vi "ZDataVIS_Stack_ITX_to_DATs.vi"(0 "File or Folder Path":path=path "G:/My Drive/ansom/Data/PPMS2/SA03008H.20180718/21-BG+SG_Sweep+OVERNIGHT", 1 "attempt to fix filtered time?":bool, 3 "length":i32=50, 5 "base processed path":path=path "C:/Users/voodoo/Desktop/IV_separat_Vsgsweep_2fields_Vbg-2.8V", 9 "pattern":string="*.itx", 12 "decimate files (1 for no)":i32=1, 14 "offset":i32) -> (4 "generated files":path[](array[path]), 6 "Index, Wavenames":string[][](table)=[["0", "'time.SA03008H.20180718.000049'\n"], ["1", "'temp.SA03008H.20180718.000049'\n"], ["2", "'B.SA03008H.20180718.000049'\n"], ["3", "'Vsource.SA03008H.20180718.000049'\n"], ["4", "'Lockin0.SA03008H.20180718.000049'\n"], ["5", "'Lockin1.SA03008H.20180718.000049'\n"], ["6", "'Lockin2.SA03008H.20180718.000049'\n"], ["7", "'Lockin3.SA03008H.20180718.000049'\n"], ["8", "'Lockin4.SA03008H.20180718.000049'\n"], ["9", "'Lockin5.SA03008H.20180718.000049'\n"], ["10", "'B_rate.SA03008H.20180718.000049'\n"], ["11", "'DC0.SA03008H.20180718.000049'\n"], ["12", "'DC1.SA03008H.20180718.000049'\n"], ["13", "'DC2.SA03008H.20180718.000049'\n"], ["14", "'DC3.SA03008H.20180718.000049'\n"], ["15", "'DC4.SA03008H.20180718.000049'\n"], ["16", "'DC5.SA03008H.20180718.000049'\n"], ["17", "'DC6.SA03008H.20180718.000049'\n"], ["18", "'DC7.SA03008H.20180718.000049'\n"], ["", ""]], 10 "\"notes \"":string[](array[string])=["IGOR\nX// Date: 7/18/2018 5:18 PM\nX// SA03008H\nX// \nX// Source 2 Drain 28 (lockin 1 and 7)\nX// Slow sweeping BG -5 to 5 inc. 0.1V \nX// Fast sweep SG -1 to 1 inc. 0.05V\n\nX// DSA_Vsg1=-1.000000\n\nX// \nX// B= 0.000000\n\n\n\n\n\n\n\n\n\n\n\n\n\n\n\n\n\n\n\n\n\n\n\n\n\n\n\n\n\n\n\n\n\n\n\n\n\n\n\n\nX \nX Display/R 'time.SA03008H.20180718.000000'\nX AppendToGraph 'temp.SA03008H.20180718.000000'\nX AppendToGraph 'B.SA03008H.20180718.000000'\nX AppendToGraph 'Vsource.SA03008H.20180718.000000'\nX AppendToGraph 'Lockin0.SA03008H.20180718.000000'\nX AppendToGraph 'Lockin1.SA03008H.20180718.000000'\nX AppendToGraph 'Lockin2.SA03008H.20180718.000000'\nX AppendToGraph 'Lockin3.SA03008H.20180718.000000'\nX AppendToGraph 'Lockin4.SA03008H.20180718.000000'\nX AppendToGraph 'Lockin5.SA03008H.20180718.000000'\nX AppendToGraph 'B_rate.SA03008H.20180718.000000'\nX AppendToGraph 'DC0.SA03008H.20180718.000000'\nX AppendToGraph 'DC1.SA03008H.20180718.000000'\nX AppendToGraph 'DC2.SA03008H.20180718.000000'\nX AppendToGraph 'DC3.SA03008H.20180718.000000'\nX AppendToGraph 'DC4.SA03008H.20180718.000000'\nX AppendToGraph 'DC5.SA03008H.20180718.000000'\nX AppendToGraph 'DC6.SA03008H.20180718.000000'\nX AppendToGraph 'DC7.SA03008H.20180718.000000'\nX Label bottom \"x label\"\nX Label left \"y label\"\nX ModifyGraph rgb('time.SA03008H.20180718.000000')=(65280,0,0)\nX ModifyGraph rgb('temp.SA03008H.20180718.000000')=(65280,18432,0)\nX ModifyGraph rgb('B.SA03008H.20180718.000000')=(65280,36864,0)\nX ModifyGraph rgb('Vsource.SA03008H.20180718.000000')=(65280,55296,0)\nX ModifyGraph rgb('Lockin0.SA03008H.20180718.000000')=(57344,65280,0)\nX ModifyGraph rgb('Lockin1.SA03008H.20180718.000000')=(37376,65280,0)\nX ModifyGraph rgb('Lockin2.SA03008H.20180718.000000')=(18944,65280,0)\nX ModifyGraph rgb('Lockin3.SA03008H.20180718.000000')=(512,65280,0)\nX ModifyGraph rgb('Lockin4.SA03008H.20180718.000000')=(0,65280,17920)\nX ModifyGraph rgb('Lockin5.SA03008H.20180718.000000')=(0,65280,36352)\nX ModifyGraph rgb('B_rate.SA03008H.20180718.000000')=(0,65280,54784)\nX ModifyGraph rgb('DC0.SA03008H.20180718.000000')=(0,57856,65280)\nX ModifyGraph rgb('DC1.SA03008H.20180718.000000')=(0,39424,65280)\nX ModifyGraph rgb('DC2.SA03008H.20180718.000000')=(0,20992,65280)\nX ModifyGraph rgb('DC3.SA03008H.20180718.000000')=(0,2560,65280)\nX ModifyGraph rgb('DC4.SA03008H.20180718.000000')=(17408,0,65280)\nX ModifyGraph rgb('DC5.SA03008H.20180718.000000')=(35840,0,65280)\nX ModifyGraph rgb('DC6.SA03008H.20180718.000000')=(54272,0,65280)\nX ModifyGraph rgb('DC7.SA03008H.20180718.000000')=(65280,0,58368)\nX Legend/C/N=text0/J \"\\\\s('time.SA03008H.20180718.000000') time\\r\\\\s('temp.SA03008H.20180718.000000') temp\\r\\\\s('B.SA03008H.20180718.000000') B\\r\\\\s('Vsource.SA03008H.20180718.000000') Vsource\\r\\\\s('Lockin0.SA03008H.20180718.000000') Lockin0\\r\\\\s('Lockin1.SA03008H.20180718.000000') Lockin1\\r\\\\s('Lockin2.SA03008H.20180718.000000') Lockin2\\r\\\\s('Lockin3.SA03008H.20180718.000000') Lockin3\\r\\\\s('Lockin4.SA03008H.20180718.000000') Lockin4\\r\\\\s('Lockin5.SA03008H.20180718.000000') Lockin5\\r\\\\s('B_rate.SA03008H.20180718.000000') B_rate\\r\\\\s('DC0.SA03008H.20180718.000000') DC0\\r\\\\s('DC1.SA03008H.20180718.000000') DC1\\r\\\\s('DC2.SA03008H.20180718.000000') DC2\\r\\\\s('DC3.SA03008H.20180718.000000') DC3\\r\\\\s('DC4.SA03008H.20180718.000000') DC4\\r\\\\s('DC5.SA03008H.20180718.000000') DC5\\r\\\\s('DC6.SA03008H.20180718.000000') DC6\\r\\\\s('DC7.SA03008H.20180718.000000') DC7\"\nX ModifyGraph mirror(bottom)=1\nX ModifyGraph width=216\nX ModifyGraph height={Aspect,0.6}\nX ModifyGraph Log(bottom)=0\nX ModifyGraph Log(left)=0\nX \n", "IGOR\nX// Date: 7/18/2018 5:18 PM\nX// SA03008H\nX// \nX// Source 2 Drain 28 (lockin 1 and 7)\nX// Slow sweeping BG -5 to 5 inc. 0.1V \nX// Fast sweep SG -1 to 1 inc. 0.05V\n\nX// DSA_Vsg1=-0.950000\n\nX// \nX// B= 0.000000\n\n\n\n\n\n\n\n\n\n\n\n\n\n\n\n\n\n\n\n\n\n\n\n\n\n\n\n\n\n\n\n\n\n\n\n\n\n\n\n\nX \nX Display/R 'time.SA03008H.20180718.000001'\nX AppendToGraph 'temp.SA03008H.20180718.000001'\nX AppendToGraph 'B.SA03008H.20180718.000001'\nX AppendToGraph 'Vsource.SA03008H.20180718.000001'\nX AppendToGraph 'Lockin0.SA03008H.20180718.000001'\nX AppendToGraph 'Lockin1.SA03008H.20180718.000001'\nX AppendToGraph 'Lockin2.SA03008H.20180718.000001'\nX AppendToGraph 'Lockin3.SA03008H.20180718.000001'\nX AppendToGraph 'Lockin4.SA03008H.20180718.000001'\nX AppendToGraph 'Lockin5.SA03008H.20180718.000001'\nX AppendToGraph 'B_rate.SA03008H.20180718.000001'\nX AppendToGraph 'DC0.SA03008H.20180718.000001'\nX AppendToGraph 'DC1.SA03008H.20180718.000001'\nX AppendToGraph 'DC2.SA03008H.20180718.000001'\nX AppendToGraph 'DC3.SA03008H.20180718.000001'\nX AppendToGraph 'DC4.SA03008H.20180718.000001'\nX AppendToGraph 'DC5.SA03008H.20180718.000001'\nX AppendToGraph 'DC6.SA03008H.20180718.000001'\nX AppendToGraph 'DC7.SA03008H.20180718.000001'\nX Label bottom \"x label\"\nX Label left \"y label\"\nX ModifyGraph rgb('time.SA03008H.20180718.000001')=(65280,0,0)\nX ModifyGraph rgb('temp.SA03008H.20180718.000001')=(65280,18432,0)\nX ModifyGraph rgb('B.SA03008H.20180718.000001')=(65280,36864,0)\nX ModifyGraph rgb('Vsource.SA03008H.20180718.000001')=(65280,55296,0)\nX ModifyGraph rgb('Lockin0.SA03008H.20180718.000001')=(57344,65280,0)\nX ModifyGraph rgb('Lockin1.SA03008H.20180718.000001')=(37376,65280,0)\nX ModifyGraph rgb('Lockin2.SA03008H.20180718.000001')=(18944,65280,0)\nX ModifyGraph rgb('Lockin3.SA03008H.20180718.000001')=(512,65280,0)\nX ModifyGraph rgb('Lockin4.SA03008H.20180718.000001')=(0,65280,17920)\nX ModifyGraph rgb('Lockin5.SA03008H.20180718.000001')=(0,65280,36352)\nX ModifyGraph rgb('B_rate.SA03008H.20180718.000001')=(0,65280,54784)\nX ModifyGraph rgb('DC0.SA03008H.20180718.000001')=(0,57856,65280)\nX ModifyGraph rgb('DC1.SA03008H.20180718.000001')=(0,39424,65280)\nX ModifyGraph rgb('DC2.SA03008H.20180718.000001')=(0,20992,65280)\nX ModifyGraph rgb('DC3.SA03008H.20180718.000001')=(0,2560,65280)\nX ModifyGraph rgb('DC4.SA03008H.20180718.000001')=(17408,0,65280)\nX ModifyGraph rgb('DC5.SA03008H.20180718.000001')=(35840,0,65280)\nX ModifyGraph rgb('DC6.SA03008H.20180718.000001')=(54272,0,65280)\nX ModifyGraph rgb('DC7.SA03008H.20180718.000001')=(65280,0,58368)\nX Legend/C/N=text0/J \"\\\\s('time.SA03008H.20180718.000001') time\\r\\\\s('temp.SA03008H.20180718.000001') temp\\r\\\\s('B.SA03008H.20180718.000001') B\\r\\\\s('Vsource.SA03008H.20180718.000001') Vsource\\r\\\\s('Lockin0.SA03008H.20180718.000001') Lockin0\\r\\\\s('Lockin1.SA03008H.20180718.000001') Lockin1\\r\\\\s('Lockin2.SA03008H.20180718.000001') Lockin2\\r\\\\s('Lockin3.SA03008H.20180718.000001') Lockin3\\r\\\\s('Lockin4.SA03008H.20180718.000001') Lockin4\\r\\\\s('Lockin5.SA03008H.20180718.000001') Lockin5\\r\\\\s('B_rate.SA03008H.20180718.000001') B_rate\\r\\\\s('DC0.SA03008H.20180718.000001') DC0\\r\\\\s('DC1.SA03008H.20180718.000001') DC1\\r\\\\s('DC2.SA03008H.20180718.000001') DC2\\r\\\\s('DC3.SA03008H.20180718.000001') DC3\\r\\\\s('DC4.SA03008H.20180718.000001') DC4\\r\\\\s('DC5.SA03008H.20180718.000001') DC5\\r\\\\s('DC6.SA03008H.20180718.000001') DC6\\r\\\\s('DC7.SA03008H.20180718.000001') DC7\"\nX ModifyGraph mirror(bottom)=1\nX ModifyGraph width=216\nX ModifyGraph height={Aspect,0.6}\nX ModifyGraph Log(bottom)=0\nX ModifyGraph Log(left)=0\nX \n", "IGOR\nX// Date: 7/18/2018 5:19 PM\nX// SA03008H\nX// \nX// Source 2 Drain 28 (lockin 1 and 7)\nX// Slow sweeping BG -5 to 5 inc. 0.1V \nX// Fast sweep SG -1 to 1 inc. 0.05V\n\nX// DSA_Vsg1=-0.900000\n\nX// \nX// B= 0.000000\n\n\n\n\n\n\n\n\n\n\n\n\n\n\n\n\n\n\n\n\n\n\n\n\n\n\n\n\n\n\n\n\n\n\n\n\n\n\n\n\nX \nX Display/R 'time.SA03008H.20180718.000002'\nX AppendToGraph 'temp.SA03008H.20180718.000002'\nX AppendToGraph 'B.SA03008H.20180718.000002'\nX AppendToGraph 'Vsource.SA03008H.20180718.000002'\nX AppendToGraph 'Lockin0.SA03008H.20180718.000002'\nX AppendToGraph 'Lockin1.SA03008H.20180718.000002'\nX AppendToGraph 'Lockin2.SA03008H.20180718.000002'\nX AppendToGraph 'Lockin3.SA03008H.20180718.000002'\nX AppendToGraph 'Lockin4.SA03008H.20180718.000002'\nX AppendToGraph 'Lockin5.SA03008H.20180718.000002'\nX AppendToGraph 'B_rate.SA03008H.20180718.000002'\nX AppendToGraph 'DC0.SA03008H.20180718.000002'\nX AppendToGraph 'DC1.SA03008H.20180718.000002'\nX AppendToGraph 'DC2.SA03008H.20180718.000002'\nX AppendToGraph 'DC3.SA03008H.20180718.000002'\nX AppendToGraph 'DC4.SA03008H.20180718.000002'\nX AppendToGraph 'DC5.SA03008H.20180718.000002'\nX AppendToGraph 'DC6.SA03008H.20180718.000002'\nX AppendToGraph 'DC7.SA03008H.20180718.000002'\nX Label bottom \"x label\"\nX Label left \"y label\"\nX ModifyGraph rgb('time.SA03008H.20180718.000002')=(65280,0,0)\nX ModifyGraph rgb('temp.SA03008H.20180718.000002')=(65280,18432,0)\nX ModifyGraph rgb('B.SA03008H.20180718.000002')=(65280,36864,0)\nX ModifyGraph rgb('Vsource.SA03008H.20180718.000002')=(65280,55296,0)\nX ModifyGraph rgb('Lockin0.SA03008H.20180718.000002')=(57344,65280,0)\nX ModifyGraph rgb('Lockin1.SA03008H.20180718.000002')=(37376,65280,0)\nX ModifyGraph rgb('Lockin2.SA03008H.20180718.000002')=(18944,65280,0)\nX ModifyGraph rgb('Lockin3.SA03008H.20180718.000002')=(512,65280,0)\nX ModifyGraph rgb('Lockin4.SA03008H.20180718.000002')=(0,65280,17920)\nX ModifyGraph rgb('Lockin5.SA03008H.20180718.000002')=(0,65280,36352)\nX ModifyGraph rgb('B_rate.SA03008H.20180718.000002')=(0,65280,54784)\nX ModifyGraph rgb('DC0.SA03008H.20180718.000002')=(0,57856,65280)\nX ModifyGraph rgb('DC1.SA03008H.20180718.000002')=(0,39424,65280)\nX ModifyGraph rgb('DC2.SA03008H.20180718.000002')=(0,20992,65280)\nX ModifyGraph rgb('DC3.SA03008H.20180718.000002')=(0,2560,65280)\nX ModifyGraph rgb('DC4.SA03008H.20180718.000002')=(17408,0,65280)\nX ModifyGraph rgb('DC5.SA03008H.20180718.000002')=(35840,0,65280)\nX ModifyGraph rgb('DC6.SA03008H.20180718.000002')=(54272,0,65280)\nX ModifyGraph rgb('DC7.SA03008H.20180718.000002')=(65280,0,58368)\nX Legend/C/N=text0/J \"\\\\s('time.SA03008H.20180718.000002') time\\r\\\\s('temp.SA03008H.20180718.000002') temp\\r\\\\s('B.SA03008H.20180718.000002') B\\r\\\\s('Vsource.SA03008H.20180718.000002') Vsource\\r\\\\s('Lockin0.SA03008H.20180718.000002') Lockin0\\r\\\\s('Lockin1.SA03008H.20180718.000002') Lockin1\\r\\\\s('Lockin2.SA03008H.20180718.000002') Lockin2\\r\\\\s('Lockin3.SA03008H.20180718.000002') Lockin3\\r\\\\s('Lockin4.SA03008H.20180718.000002') Lockin4\\r\\\\s('Lockin5.SA03008H.20180718.000002') Lockin5\\r\\\\s('B_rate.SA03008H.20180718.000002') B_rate\\r\\\\s('DC0.SA03008H.20180718.000002') DC0\\r\\\\s('DC1.SA03008H.20180718.000002') DC1\\r\\\\s('DC2.SA03008H.20180718.000002') DC2\\r\\\\s('DC3.SA03008H.20180718.000002') DC3\\r\\\\s('DC4.SA03008H.20180718.000002') DC4\\r\\\\s('DC5.SA03008H.20180718.000002') DC5\\r\\\\s('DC6.SA03008H.20180718.000002') DC6\\r\\\\s('DC7.SA03008H.20180718.000002') DC7\"\nX ModifyGraph mirror(bottom)=1\nX ModifyGraph width=216\nX ModifyGraph height={Aspect,0.6}\nX ModifyGraph Log(bottom)=0\nX ModifyGraph Log(left)=0\nX \n", "IGOR\nX// Date: 7/18/2018 5:19 PM\nX// SA03008H\nX// \nX// Source 2 Drain 28 (lockin 1 and 7)\nX// Slow sweeping BG -5 to 5 inc. 0.1V \nX// Fast sweep SG -1 to 1 inc. 0.05V\n\nX// DSA_Vsg1=-0.850000\n\nX// \nX// B= 0.000000\n\n\n\n\n\n\n\n\n\n\n\n\n\n\n\n\n\n\n\n\n\n\n\n\n\n\n\n\n\n\n\n\n\n\n\n\n\n\n\n\nX \nX Display/R 'time.SA03008H.20180718.000003'\nX AppendToGraph 'temp.SA03008H.20180718.000003'\nX AppendToGraph 'B.SA03008H.20180718.000003'\nX AppendToGraph 'Vsource.SA03008H.20180718.000003'\nX AppendToGraph 'Lockin0.SA03008H.20180718.000003'\nX AppendToGraph 'Lockin1.SA03008H.20180718.000003'\nX AppendToGraph 'Lockin2.SA03008H.20180718.000003'\nX AppendToGraph 'Lockin3.SA03008H.20180718.000003'\nX AppendToGraph 'Lockin4.SA03008H.20180718.000003'\nX AppendToGraph 'Lockin5.SA03008H.20180718.000003'\nX AppendToGraph 'B_rate.SA03008H.20180718.000003'\nX AppendToGraph 'DC0.SA03008H.20180718.000003'\nX AppendToGraph 'DC1.SA03008H.20180718.000003'\nX AppendToGraph 'DC2.SA03008H.20180718.000003'\nX AppendToGraph 'DC3.SA03008H.20180718.000003'\nX AppendToGraph 'DC4.SA03008H.20180718.000003'\nX AppendToGraph 'DC5.SA03008H.20180718.000003'\nX AppendToGraph 'DC6.SA03008H.20180718.000003'\nX AppendToGraph 'DC7.SA03008H.20180718.000003'\nX Label bottom \"x label\"\nX Label left \"y label\"\nX ModifyGraph rgb('time.SA03008H.20180718.000003')=(65280,0,0)\nX ModifyGraph rgb('temp.SA03008H.20180718.000003')=(65280,18432,0)\nX ModifyGraph rgb('B.SA03008H.20180718.000003')=(65280,36864,0)\nX ModifyGraph rgb('Vsource.SA03008H.20180718.000003')=(65280,55296,0)\nX ModifyGraph rgb('Lockin0.SA03008H.20180718.000003')=(57344,65280,0)\nX ModifyGraph rgb('Lockin1.SA03008H.20180718.000003')=(37376,65280,0)\nX ModifyGraph rgb('Lockin2.SA03008H.20180718.000003')=(18944,65280,0)\nX ModifyGraph rgb('Lockin3.SA03008H.20180718.000003')=(512,65280,0)\nX ModifyGraph rgb('Lockin4.SA03008H.20180718.000003')=(0,65280,17920)\nX ModifyGraph rgb('Lockin5.SA03008H.20180718.000003')=(0,65280,36352)\nX ModifyGraph rgb('B_rate.SA03008H.20180718.000003')=(0,65280,54784)\nX ModifyGraph rgb('DC0.SA03008H.20180718.000003')=(0,57856,65280)\nX ModifyGraph rgb('DC1.SA03008H.20180718.000003')=(0,39424,65280)\nX ModifyGraph rgb('DC2.SA03008H.20180718.000003')=(0,20992,65280)\nX ModifyGraph rgb('DC3.SA03008H.20180718.000003')=(0,2560,65280)\nX ModifyGraph rgb('DC4.SA03008H.20180718.000003')=(17408,0,65280)\nX ModifyGraph rgb('DC5.SA03008H.20180718.000003')=(35840,0,65280)\nX ModifyGraph rgb('DC6.SA03008H.20180718.000003')=(54272,0,65280)\nX ModifyGraph rgb('DC7.SA03008H.20180718.000003')=(65280,0,58368)\nX Legend/C/N=text0/J \"\\\\s('time.SA03008H.20180718.000003') time\\r\\\\s('temp.SA03008H.20180718.000003') temp\\r\\\\s('B.SA03008H.20180718.000003') B\\r\\\\s('Vsource.SA03008H.20180718.000003') Vsource\\r\\\\s('Lockin0.SA03008H.20180718.000003') Lockin0\\r\\\\s('Lockin1.SA03008H.20180718.000003') Lockin1\\r\\\\s('Lockin2.SA03008H.20180718.000003') Lockin2\\r\\\\s('Lockin3.SA03008H.20180718.000003') Lockin3\\r\\\\s('Lockin4.SA03008H.20180718.000003') Lockin4\\r\\\\s('Lockin5.SA03008H.20180718.000003') Lockin5\\r\\\\s('B_rate.SA03008H.20180718.000003') B_rate\\r\\\\s('DC0.SA03008H.20180718.000003') DC0\\r\\\\s('DC1.SA03008H.20180718.000003') DC1\\r\\\\s('DC2.SA03008H.20180718.000003') DC2\\r\\\\s('DC3.SA03008H.20180718.000003') DC3\\r\\\\s('DC4.SA03008H.20180718.000003') DC4\\r\\\\s('DC5.SA03008H.20180718.000003') DC5\\r\\\\s('DC6.SA03008H.20180718.000003') DC6\\r\\\\s('DC7.SA03008H.20180718.000003') DC7\"\nX ModifyGraph mirror(bottom)=1\nX ModifyGraph width=216\nX ModifyGraph height={Aspect,0.6}\nX ModifyGraph Log(bottom)=0\nX ModifyGraph Log(left)=0\nX \n", "IGOR\nX// Date: 7/18/2018 5:19 PM\nX// SA03008H\nX// \nX// Source 2 Drain 28 (lockin 1 and 7)\nX// Slow sweeping BG -5 to 5 inc. 0.1V \nX// Fast sweep SG -1 to 1 inc. 0.05V\n\nX// DSA_Vsg1=-0.800000\n\nX// \nX// B= 0.000000\n\n\n\n\n\n\n\n\n\n\n\n\n\n\n\n\n\n\n\n\n\n\n\n\n\n\n\n\n\n\n\n\n\n\n\n\n\n\n\n\nX \nX Display/R 'time.SA03008H.20180718.000004'\nX AppendToGraph 'temp.SA03008H.20180718.000004'\nX AppendToGraph 'B.SA03008H.20180718.000004'\nX AppendToGraph 'Vsource.SA03008H.20180718.000004'\nX AppendToGraph 'Lockin0.SA03008H.20180718.000004'\nX AppendToGraph 'Lockin1.SA03008H.20180718.000004'\nX AppendToGraph 'Lockin2.SA03008H.20180718.000004'\nX AppendToGraph 'Lockin3.SA03008H.20180718.000004'\nX AppendToGraph 'Lockin4.SA03008H.20180718.000004'\nX AppendToGraph 'Lockin5.SA03008H.20180718.000004'\nX AppendToGraph 'B_rate.SA03008H.20180718.000004'\nX AppendToGraph 'DC0.SA03008H.20180718.000004'\nX AppendToGraph 'DC1.SA03008H.20180718.000004'\nX AppendToGraph 'DC2.SA03008H.20180718.000004'\nX AppendToGraph 'DC3.SA03008H.20180718.000004'\nX AppendToGraph 'DC4.SA03008H.20180718.000004'\nX AppendToGraph 'DC5.SA03008H.20180718.000004'\nX AppendToGraph 'DC6.SA03008H.20180718.000004'\nX AppendToGraph 'DC7.SA03008H.20180718.000004'\nX Label bottom \"x label\"\nX Label left \"y label\"\nX ModifyGraph rgb('time.SA03008H.20180718.000004')=(65280,0,0)\nX ModifyGraph rgb('temp.SA03008H.20180718.000004')=(65280,18432,0)\nX ModifyGraph rgb('B.SA03008H.20180718.000004')=(65280,36864,0)\nX ModifyGraph rgb('Vsource.SA03008H.20180718.000004')=(65280,55296,0)\nX ModifyGraph rgb('Lockin0.SA03008H.20180718.000004')=(57344,65280,0)\nX ModifyGraph rgb('Lockin1.SA03008H.20180718.000004')=(37376,65280,0)\nX ModifyGraph rgb('Lockin2.SA03008H.20180718.000004')=(18944,65280,0)\nX ModifyGraph rgb('Lockin3.SA03008H.20180718.000004')=(512,65280,0)\nX ModifyGraph rgb('Lockin4.SA03008H.20180718.000004')=(0,65280,17920)\nX ModifyGraph rgb('Lockin5.SA03008H.20180718.000004')=(0,65280,36352)\nX ModifyGraph rgb('B_rate.SA03008H.20180718.000004')=(0,65280,54784)\nX ModifyGraph rgb('DC0.SA03008H.20180718.000004')=(0,57856,65280)\nX ModifyGraph rgb('DC1.SA03008H.20180718.000004')=(0,39424,65280)\nX ModifyGraph rgb('DC2.SA03008H.20180718.000004')=(0,20992,65280)\nX ModifyGraph rgb('DC3.SA03008H.20180718.000004')=(0,2560,65280)\nX ModifyGraph rgb('DC4.SA03008H.20180718.000004')=(17408,0,65280)\nX ModifyGraph rgb('DC5.SA03008H.20180718.000004')=(35840,0,65280)\nX ModifyGraph rgb('DC6.SA03008H.20180718.000004')=(54272,0,65280)\nX ModifyGraph rgb('DC7.SA03008H.20180718.000004')=(65280,0,58368)\nX Legend/C/N=text0/J \"\\\\s('time.SA03008H.20180718.000004') time\\r\\\\s('temp.SA03008H.20180718.000004') temp\\r\\\\s('B.SA03008H.20180718.000004') B\\r\\\\s('Vsource.SA03008H.20180718.000004') Vsource\\r\\\\s('Lockin0.SA03008H.20180718.000004') Lockin0\\r\\\\s('Lockin1.SA03008H.20180718.000004') Lockin1\\r\\\\s('Lockin2.SA03008H.20180718.000004') Lockin2\\r\\\\s('Lockin3.SA03008H.20180718.000004') Lockin3\\r\\\\s('Lockin4.SA03008H.20180718.000004') Lockin4\\r\\\\s('Lockin5.SA03008H.20180718.000004') Lockin5\\r\\\\s('B_rate.SA03008H.20180718.000004') B_rate\\r\\\\s('DC0.SA03008H.20180718.000004') DC0\\r\\\\s('DC1.SA03008H.20180718.000004') DC1\\r\\\\s('DC2.SA03008H.20180718.000004') DC2\\r\\\\s('DC3.SA03008H.20180718.000004') DC3\\r\\\\s('DC4.SA03008H.20180718.000004') DC4\\r\\\\s('DC5.SA03008H.20180718.000004') DC5\\r\\\\s('DC6.SA03008H.20180718.000004') DC6\\r\\\\s('DC7.SA03008H.20180718.000004') DC7\"\nX ModifyGraph mirror(bottom)=1\nX ModifyGraph width=216\nX ModifyGraph height={Aspect,0.6}\nX ModifyGraph Log(bottom)=0\nX ModifyGraph Log(left)=0\nX \n", "IGOR\nX// Date: 7/18/2018 5:19 PM\nX// SA03008H\nX// \nX// Source 2 Drain 28 (lockin 1 and 7)\nX// Slow sweeping BG -5 to 5 inc. 0.1V \nX// Fast sweep SG -1 to 1 inc. 0.05V\n\nX// DSA_Vsg1=-0.750000\n\nX// \nX// B= 0.000000\n\n\n\n\n\n\n\n\n\n\n\n\n\n\n\n\n\n\n\n\n\n\n\n\n\n\n\n\n\n\n\n\n\n\n\n\n\n\n\n\nX \nX Display/R 'time.SA03008H.20180718.000005'\nX AppendToGraph 'temp.SA03008H.20180718.000005'\nX AppendToGraph 'B.SA03008H.20180718.000005'\nX AppendToGraph 'Vsource.SA03008H.20180718.000005'\nX AppendToGraph 'Lockin0.SA03008H.20180718.000005'\nX AppendToGraph 'Lockin1.SA03008H.20180718.000005'\nX AppendToGraph 'Lockin2.SA03008H.20180718.000005'\nX AppendToGraph 'Lockin3.SA03008H.20180718.000005'\nX AppendToGraph 'Lockin4.SA03008H.20180718.000005'\nX AppendToGraph 'Lockin5.SA03008H.20180718.000005'\nX AppendToGraph 'B_rate.SA03008H.20180718.000005'\nX AppendToGraph 'DC0.SA03008H.20180718.000005'\nX AppendToGraph 'DC1.SA03008H.20180718.000005'\nX AppendToGraph 'DC2.SA03008H.20180718.000005'\nX AppendToGraph 'DC3.SA03008H.20180718.000005'\nX AppendToGraph 'DC4.SA03008H.20180718.000005'\nX AppendToGraph 'DC5.SA03008H.20180718.000005'\nX AppendToGraph 'DC6.SA03008H.20180718.000005'\nX AppendToGraph 'DC7.SA03008H.20180718.000005'\nX Label bottom \"x label\"\nX Label left \"y label\"\nX ModifyGraph rgb('time.SA03008H.20180718.000005')=(65280,0,0)\nX ModifyGraph rgb('temp.SA03008H.20180718.000005')=(65280,18432,0)\nX ModifyGraph rgb('B.SA03008H.20180718.000005')=(65280,36864,0)\nX ModifyGraph rgb('Vsource.SA03008H.20180718.000005')=(65280,55296,0)\nX ModifyGraph rgb('Lockin0.SA03008H.20180718.000005')=(57344,65280,0)\nX ModifyGraph rgb('Lockin1.SA03008H.20180718.000005')=(37376,65280,0)\nX ModifyGraph rgb('Lockin2.SA03008H.20180718.000005')=(18944,65280,0)\nX ModifyGraph rgb('Lockin3.SA03008H.20180718.000005')=(512,65280,0)\nX ModifyGraph rgb('Lockin4.SA03008H.20180718.000005')=(0,65280,17920)\nX ModifyGraph rgb('Lockin5.SA03008H.20180718.000005')=(0,65280,36352)\nX ModifyGraph rgb('B_rate.SA03008H.20180718.000005')=(0,65280,54784)\nX ModifyGraph rgb('DC0.SA03008H.20180718.000005')=(0,57856,65280)\nX ModifyGraph rgb('DC1.SA03008H.20180718.000005')=(0,39424,65280)\nX ModifyGraph rgb('DC2.SA03008H.20180718.000005')=(0,20992,65280)\nX ModifyGraph rgb('DC3.SA03008H.20180718.000005')=(0,2560,65280)\nX ModifyGraph rgb('DC4.SA03008H.20180718.000005')=(17408,0,65280)\nX ModifyGraph rgb('DC5.SA03008H.20180718.000005')=(35840,0,65280)\nX ModifyGraph rgb('DC6.SA03008H.20180718.000005')=(54272,0,65280)\nX ModifyGraph rgb('DC7.SA03008H.20180718.000005')=(65280,0,58368)\nX Legend/C/N=text0/J \"\\\\s('time.SA03008H.20180718.000005') time\\r\\\\s('temp.SA03008H.20180718.000005') temp\\r\\\\s('B.SA03008H.20180718.000005') B\\r\\\\s('Vsource.SA03008H.20180718.000005') Vsource\\r\\\\s('Lockin0.SA03008H.20180718.000005') Lockin0\\r\\\\s('Lockin1.SA03008H.20180718.000005') Lockin1\\r\\\\s('Lockin2.SA03008H.20180718.000005') Lockin2\\r\\\\s('Lockin3.SA03008H.20180718.000005') Lockin3\\r\\\\s('Lockin4.SA03008H.20180718.000005') Lockin4\\r\\\\s('Lockin5.SA03008H.20180718.000005') Lockin5\\r\\\\s('B_rate.SA03008H.20180718.000005') B_rate\\r\\\\s('DC0.SA03008H.20180718.000005') DC0\\r\\\\s('DC1.SA03008H.20180718.000005') DC1\\r\\\\s('DC2.SA03008H.20180718.000005') DC2\\r\\\\s('DC3.SA03008H.20180718.000005') DC3\\r\\\\s('DC4.SA03008H.20180718.000005') DC4\\r\\\\s('DC5.SA03008H.20180718.000005') DC5\\r\\\\s('DC6.SA03008H.20180718.000005') DC6\\r\\\\s('DC7.SA03008H.20180718.000005') DC7\"\nX ModifyGraph mirror(bottom)=1\nX ModifyGraph width=216\nX ModifyGraph height={Aspect,0.6}\nX ModifyGraph Log(bottom)=0\nX ModifyGraph Log(left)=0\nX \n", "IGOR\nX// Date: 7/18/2018 5:19 PM\nX// SA03008H\nX// \nX// Source 2 Drain 28 (lockin 1 and 7)\nX// Slow sweeping BG -5 to 5 inc. 0.1V \nX// Fast sweep SG -1 to 1 inc. 0.05V\n\nX// DSA_Vsg1=-0.700000\n\nX// \nX// B= 0.000000\n\n\n\n\n\n\n\n\n\n\n\n\n\n\n\n\n\n\n\n\n\n\n\n\n\n\n\n\n\n\n\n\n\n\n\n\n\n\n\n\nX \nX Display/R 'time.SA03008H.20180718.000006'\nX AppendToGraph 'temp.SA03008H.20180718.000006'\nX AppendToGraph 'B.SA03008H.20180718.000006'\nX AppendToGraph 'Vsource.SA03008H.20180718.000006'\nX AppendToGraph 'Lockin0.SA03008H.20180718.000006'\nX AppendToGraph 'Lockin1.SA03008H.20180718.000006'\nX AppendToGraph 'Lockin2.SA03008H.20180718.000006'\nX AppendToGraph 'Lockin3.SA03008H.20180718.000006'\nX AppendToGraph 'Lockin4.SA03008H.20180718.000006'\nX AppendToGraph 'Lockin5.SA03008H.20180718.000006'\nX AppendToGraph 'B_rate.SA03008H.20180718.000006'\nX AppendToGraph 'DC0.SA03008H.20180718.000006'\nX AppendToGraph 'DC1.SA03008H.20180718.000006'\nX AppendToGraph 'DC2.SA03008H.20180718.000006'\nX AppendToGraph 'DC3.SA03008H.20180718.000006'\nX AppendToGraph 'DC4.SA03008H.20180718.000006'\nX AppendToGraph 'DC5.SA03008H.20180718.000006'\nX AppendToGraph 'DC6.SA03008H.20180718.000006'\nX AppendToGraph 'DC7.SA03008H.20180718.000006'\nX Label bottom \"x label\"\nX Label left \"y label\"\nX ModifyGraph rgb('time.SA03008H.20180718.000006')=(65280,0,0)\nX ModifyGraph rgb('temp.SA03008H.20180718.000006')=(65280,18432,0)\nX ModifyGraph rgb('B.SA03008H.20180718.000006')=(65280,36864,0)\nX ModifyGraph rgb('Vsource.SA03008H.20180718.000006')=(65280,55296,0)\nX ModifyGraph rgb('Lockin0.SA03008H.20180718.000006')=(57344,65280,0)\nX ModifyGraph rgb('Lockin1.SA03008H.20180718.000006')=(37376,65280,0)\nX ModifyGraph rgb('Lockin2.SA03008H.20180718.000006')=(18944,65280,0)\nX ModifyGraph rgb('Lockin3.SA03008H.20180718.000006')=(512,65280,0)\nX ModifyGraph rgb('Lockin4.SA03008H.20180718.000006')=(0,65280,17920)\nX ModifyGraph rgb('Lockin5.SA03008H.20180718.000006')=(0,65280,36352)\nX ModifyGraph rgb('B_rate.SA03008H.20180718.000006')=(0,65280,54784)\nX ModifyGraph rgb('DC0.SA03008H.20180718.000006')=(0,57856,65280)\nX ModifyGraph rgb('DC1.SA03008H.20180718.000006')=(0,39424,65280)\nX ModifyGraph rgb('DC2.SA03008H.20180718.000006')=(0,20992,65280)\nX ModifyGraph rgb('DC3.SA03008H.20180718.000006')=(0,2560,65280)\nX ModifyGraph rgb('DC4.SA03008H.20180718.000006')=(17408,0,65280)\nX ModifyGraph rgb('DC5.SA03008H.20180718.000006')=(35840,0,65280)\nX ModifyGraph rgb('DC6.SA03008H.20180718.000006')=(54272,0,65280)\nX ModifyGraph rgb('DC7.SA03008H.20180718.000006')=(65280,0,58368)\nX Legend/C/N=text0/J \"\\\\s('time.SA03008H.20180718.000006') time\\r\\\\s('temp.SA03008H.20180718.000006') temp\\r\\\\s('B.SA03008H.20180718.000006') B\\r\\\\s('Vsource.SA03008H.20180718.000006') Vsource\\r\\\\s('Lockin0.SA03008H.20180718.000006') Lockin0\\r\\\\s('Lockin1.SA03008H.20180718.000006') Lockin1\\r\\\\s('Lockin2.SA03008H.20180718.000006') Lockin2\\r\\\\s('Lockin3.SA03008H.20180718.000006') Lockin3\\r\\\\s('Lockin4.SA03008H.20180718.000006') Lockin4\\r\\\\s('Lockin5.SA03008H.20180718.000006') Lockin5\\r\\\\s('B_rate.SA03008H.20180718.000006') B_rate\\r\\\\s('DC0.SA03008H.20180718.000006') DC0\\r\\\\s('DC1.SA03008H.20180718.000006') DC1\\r\\\\s('DC2.SA03008H.20180718.000006') DC2\\r\\\\s('DC3.SA03008H.20180718.000006') DC3\\r\\\\s('DC4.SA03008H.20180718.000006') DC4\\r\\\\s('DC5.SA03008H.20180718.000006') DC5\\r\\\\s('DC6.SA03008H.20180718.000006') DC6\\r\\\\s('DC7.SA03008H.20180718.000006') DC7\"\nX ModifyGraph mirror(bottom)=1\nX ModifyGraph width=216\nX ModifyGraph height={Aspect,0.6}\nX ModifyGraph Log(bottom)=0\nX ModifyGraph Log(left)=0\nX \n", "IGOR\nX// Date: 7/18/2018 5:20 PM\nX// SA03008H\nX// \nX// Source 2 Drain 28 (lockin 1 and 7)\nX// Slow sweeping BG -5 to 5 inc. 0.1V \nX// Fast sweep SG -1 to 1 inc. 0.05V\n\nX// DSA_Vsg1=-0.650000\n\nX// \nX// B= 0.000000\n\n\n\n\n\n\n\n\n\n\n\n\n\n\n\n\n\n\n\n\n\n\n\n\n\n\n\n\n\n\n\n\n\n\n\n\n\n\n\n\nX \nX Display/R 'time.SA03008H.20180718.000007'\nX AppendToGraph 'temp.SA03008H.20180718.000007'\nX AppendToGraph 'B.SA03008H.20180718.000007'\nX AppendToGraph 'Vsource.SA03008H.20180718.000007'\nX AppendToGraph 'Lockin0.SA03008H.20180718.000007'\nX AppendToGraph 'Lockin1.SA03008H.20180718.000007'\nX AppendToGraph 'Lockin2.SA03008H.20180718.000007'\nX AppendToGraph 'Lockin3.SA03008H.20180718.000007'\nX AppendToGraph 'Lockin4.SA03008H.20180718.000007'\nX AppendToGraph 'Lockin5.SA03008H.20180718.000007'\nX AppendToGraph 'B_rate.SA03008H.20180718.000007'\nX AppendToGraph 'DC0.SA03008H.20180718.000007'\nX AppendToGraph 'DC1.SA03008H.20180718.000007'\nX AppendToGraph 'DC2.SA03008H.20180718.000007'\nX AppendToGraph 'DC3.SA03008H.20180718.000007'\nX AppendToGraph 'DC4.SA03008H.20180718.000007'\nX AppendToGraph 'DC5.SA03008H.20180718.000007'\nX AppendToGraph 'DC6.SA03008H.20180718.000007'\nX AppendToGraph 'DC7.SA03008H.20180718.000007'\nX Label bottom \"x label\"\nX Label left \"y label\"\nX ModifyGraph rgb('time.SA03008H.20180718.000007')=(65280,0,0)\nX ModifyGraph rgb('temp.SA03008H.20180718.000007')=(65280,18432,0)\nX ModifyGraph rgb('B.SA03008H.20180718.000007')=(65280,36864,0)\nX ModifyGraph rgb('Vsource.SA03008H.20180718.000007')=(65280,55296,0)\nX ModifyGraph rgb('Lockin0.SA03008H.20180718.000007')=(57344,65280,0)\nX ModifyGraph rgb('Lockin1.SA03008H.20180718.000007')=(37376,65280,0)\nX ModifyGraph rgb('Lockin2.SA03008H.20180718.000007')=(18944,65280,0)\nX ModifyGraph rgb('Lockin3.SA03008H.20180718.000007')=(512,65280,0)\nX ModifyGraph rgb('Lockin4.SA03008H.20180718.000007')=(0,65280,17920)\nX ModifyGraph rgb('Lockin5.SA03008H.20180718.000007')=(0,65280,36352)\nX ModifyGraph rgb('B_rate.SA03008H.20180718.000007')=(0,65280,54784)\nX ModifyGraph rgb('DC0.SA03008H.20180718.000007')=(0,57856,65280)\nX ModifyGraph rgb('DC1.SA03008H.20180718.000007')=(0,39424,65280)\nX ModifyGraph rgb('DC2.SA03008H.20180718.000007')=(0,20992,65280)\nX ModifyGraph rgb('DC3.SA03008H.20180718.000007')=(0,2560,65280)\nX ModifyGraph rgb('DC4.SA03008H.20180718.000007')=(17408,0,65280)\nX ModifyGraph rgb('DC5.SA03008H.20180718.000007')=(35840,0,65280)\nX ModifyGraph rgb('DC6.SA03008H.20180718.000007')=(54272,0,65280)\nX ModifyGraph rgb('DC7.SA03008H.20180718.000007')=(65280,0,58368)\nX Legend/C/N=text0/J \"\\\\s('time.SA03008H.20180718.000007') time\\r\\\\s('temp.SA03008H.20180718.000007') temp\\r\\\\s('B.SA03008H.20180718.000007') B\\r\\\\s('Vsource.SA03008H.20180718.000007') Vsource\\r\\\\s('Lockin0.SA03008H.20180718.000007') Lockin0\\r\\\\s('Lockin1.SA03008H.20180718.000007') Lockin1\\r\\\\s('Lockin2.SA03008H.20180718.000007') Lockin2\\r\\\\s('Lockin3.SA03008H.20180718.000007') Lockin3\\r\\\\s('Lockin4.SA03008H.20180718.000007') Lockin4\\r\\\\s('Lockin5.SA03008H.20180718.000007') Lockin5\\r\\\\s('B_rate.SA03008H.20180718.000007') B_rate\\r\\\\s('DC0.SA03008H.20180718.000007') DC0\\r\\\\s('DC1.SA03008H.20180718.000007') DC1\\r\\\\s('DC2.SA03008H.20180718.000007') DC2\\r\\\\s('DC3.SA03008H.20180718.000007') DC3\\r\\\\s('DC4.SA03008H.20180718.000007') DC4\\r\\\\s('DC5.SA03008H.20180718.000007') DC5\\r\\\\s('DC6.SA03008H.20180718.000007') DC6\\r\\\\s('DC7.SA03008H.20180718.000007') DC7\"\nX ModifyGraph mirror(bottom)=1\nX ModifyGraph width=216\nX ModifyGraph height={Aspect,0.6}\nX ModifyGraph Log(bottom)=0\nX ModifyGraph Log(left)=0\nX \n", "IGOR\nX// Date: 7/18/2018 5:20 PM\nX// SA03008H\nX// \nX// Source 2 Drain 28 (lockin 1 and 7)\nX// Slow sweeping BG -5 to 5 inc. 0.1V \nX// Fast sweep SG -1 to 1 inc. 0.05V\n\nX// DSA_Vsg1=-0.600000\n\nX// \nX// B= 0.000000\n\n\n\n\n\n\n\n\n\n\n\n\n\n\n\n\n\n\n\n\n\n\n\n\n\n\n\n\n\n\n\n\n\n\n\n\n\n\n\n\nX \nX Display/R 'time.SA03008H.20180718.000008'\nX AppendToGraph 'temp.SA03008H.20180718.000008'\nX AppendToGraph 'B.SA03008H.20180718.000008'\nX AppendToGraph 'Vsource.SA03008H.20180718.000008'\nX AppendToGraph 'Lockin0.SA03008H.20180718.000008'\nX AppendToGraph 'Lockin1.SA03008H.20180718.000008'\nX AppendToGraph 'Lockin2.SA03008H.20180718.000008'\nX AppendToGraph 'Lockin3.SA03008H.20180718.000008'\nX AppendToGraph 'Lockin4.SA03008H.20180718.000008'\nX AppendToGraph 'Lockin5.SA03008H.20180718.000008'\nX AppendToGraph 'B_rate.SA03008H.20180718.000008'\nX AppendToGraph 'DC0.SA03008H.20180718.000008'\nX AppendToGraph 'DC1.SA03008H.20180718.000008'\nX AppendToGraph 'DC2.SA03008H.20180718.000008'\nX AppendToGraph 'DC3.SA03008H.20180718.000008'\nX AppendToGraph 'DC4.SA03008H.20180718.000008'\nX AppendToGraph 'DC5.SA03008H.20180718.000008'\nX AppendToGraph 'DC6.SA03008H.20180718.000008'\nX AppendToGraph 'DC7.SA03008H.20180718.000008'\nX Label bottom \"x label\"\nX Label left \"y label\"\nX ModifyGraph rgb('time.SA03008H.20180718.000008')=(65280,0,0)\nX ModifyGraph rgb('temp.SA03008H.20180718.000008')=(65280,18432,0)\nX ModifyGraph rgb('B.SA03008H.20180718.000008')=(65280,36864,0)\nX ModifyGraph rgb('Vsource.SA03008H.20180718.000008')=(65280,55296,0)\nX ModifyGraph rgb('Lockin0.SA03008H.20180718.000008')=(57344,65280,0)\nX ModifyGraph rgb('Lockin1.SA03008H.20180718.000008')=(37376,65280,0)\nX ModifyGraph rgb('Lockin2.SA03008H.20180718.000008')=(18944,65280,0)\nX ModifyGraph rgb('Lockin3.SA03008H.20180718.000008')=(512,65280,0)\nX ModifyGraph rgb('Lockin4.SA03008H.20180718.000008')=(0,65280,17920)\nX ModifyGraph rgb('Lockin5.SA03008H.20180718.000008')=(0,65280,36352)\nX ModifyGraph rgb('B_rate.SA03008H.20180718.000008')=(0,65280,54784)\nX ModifyGraph rgb('DC0.SA03008H.20180718.000008')=(0,57856,65280)\nX ModifyGraph rgb('DC1.SA03008H.20180718.000008')=(0,39424,65280)\nX ModifyGraph rgb('DC2.SA03008H.20180718.000008')=(0,20992,65280)\nX ModifyGraph rgb('DC3.SA03008H.20180718.000008')=(0,2560,65280)\nX ModifyGraph rgb('DC4.SA03008H.20180718.000008')=(17408,0,65280)\nX ModifyGraph rgb('DC5.SA03008H.20180718.000008')=(35840,0,65280)\nX ModifyGraph rgb('DC6.SA03008H.20180718.000008')=(54272,0,65280)\nX ModifyGraph rgb('DC7.SA03008H.20180718.000008')=(65280,0,58368)\nX Legend/C/N=text0/J \"\\\\s('time.SA03008H.20180718.000008') time\\r\\\\s('temp.SA03008H.20180718.000008') temp\\r\\\\s('B.SA03008H.20180718.000008') B\\r\\\\s('Vsource.SA03008H.20180718.000008') Vsource\\r\\\\s('Lockin0.SA03008H.20180718.000008') Lockin0\\r\\\\s('Lockin1.SA03008H.20180718.000008') Lockin1\\r\\\\s('Lockin2.SA03008H.20180718.000008') Lockin2\\r\\\\s('Lockin3.SA03008H.20180718.000008') Lockin3\\r\\\\s('Lockin4.SA03008H.20180718.000008') Lockin4\\r\\\\s('Lockin5.SA03008H.20180718.000008') Lockin5\\r\\\\s('B_rate.SA03008H.20180718.000008') B_rate\\r\\\\s('DC0.SA03008H.20180718.000008') DC0\\r\\\\s('DC1.SA03008H.20180718.000008') DC1\\r\\\\s('DC2.SA03008H.20180718.000008') DC2\\r\\\\s('DC3.SA03008H.20180718.000008') DC3\\r\\\\s('DC4.SA03008H.20180718.000008') DC4\\r\\\\s('DC5.SA03008H.20180718.000008') DC5\\r\\\\s('DC6.SA03008H.20180718.000008') DC6\\r\\\\s('DC7.SA03008H.20180718.000008') DC7\"\nX ModifyGraph mirror(bottom)=1\nX ModifyGraph width=216\nX ModifyGraph height={Aspect,0.6}\nX ModifyGraph Log(bottom)=0\nX ModifyGraph Log(left)=0\nX \n", "IGOR\nX// Date: 7/18/2018 5:20 PM\nX// SA03008H\nX// \nX// Source 2 Drain 28 (lockin 1 and 7)\nX// Slow sweeping BG -5 to 5 inc. 0.1V \nX// Fast sweep SG -1 to 1 inc. 0.05V\n\nX// DSA_Vsg1=-0.550000\n\nX// \nX// B= 0.000000\n\n\n\n\n\n\n\n\n\n\n\n\n\n\n\n\n\n\n\n\n\n\n\n\n\n\n\n\n\n\n\n\n\n\n\n\n\n\n\n\nX \nX Display/R 'time.SA03008H.20180718.000009'\nX AppendToGraph 'temp.SA03008H.20180718.000009'\nX AppendToGraph 'B.SA03008H.20180718.000009'\nX AppendToGraph 'Vsource.SA03008H.20180718.000009'\nX AppendToGraph 'Lockin0.SA03008H.20180718.000009'\nX AppendToGraph 'Lockin1.SA03008H.20180718.000009'\nX AppendToGraph 'Lockin2.SA03008H.20180718.000009'\nX AppendToGraph 'Lockin3.SA03008H.20180718.000009'\nX AppendToGraph 'Lockin4.SA03008H.20180718.000009'\nX AppendToGraph 'Lockin5.SA03008H.20180718.000009'\nX AppendToGraph 'B_rate.SA03008H.20180718.000009'\nX AppendToGraph 'DC0.SA03008H.20180718.000009'\nX AppendToGraph 'DC1.SA03008H.20180718.000009'\nX AppendToGraph 'DC2.SA03008H.20180718.000009'\nX AppendToGraph 'DC3.SA03008H.20180718.000009'\nX AppendToGraph 'DC4.SA03008H.20180718.000009'\nX AppendToGraph 'DC5.SA03008H.20180718.000009'\nX AppendToGraph 'DC6.SA03008H.20180718.000009'\nX AppendToGraph 'DC7.SA03008H.20180718.000009'\nX Label bottom \"x label\"\nX Label left \"y label\"\nX ModifyGraph rgb('time.SA03008H.20180718.000009')=(65280,0,0)\nX ModifyGraph rgb('temp.SA03008H.20180718.000009')=(65280,18432,0)\nX ModifyGraph rgb('B.SA03008H.20180718.000009')=(65280,36864,0)\nX ModifyGraph rgb('Vsource.SA03008H.20180718.000009')=(65280,55296,0)\nX ModifyGraph rgb('Lockin0.SA03008H.20180718.000009')=(57344,65280,0)\nX ModifyGraph rgb('Lockin1.SA03008H.20180718.000009')=(37376,65280,0)\nX ModifyGraph rgb('Lockin2.SA03008H.20180718.000009')=(18944,65280,0)\nX ModifyGraph rgb('Lockin3.SA03008H.20180718.000009')=(512,65280,0)\nX ModifyGraph rgb('Lockin4.SA03008H.20180718.000009')=(0,65280,17920)\nX ModifyGraph rgb('Lockin5.SA03008H.20180718.000009')=(0,65280,36352)\nX ModifyGraph rgb('B_rate.SA03008H.20180718.000009')=(0,65280,54784)\nX ModifyGraph rgb('DC0.SA03008H.20180718.000009')=(0,57856,65280)\nX ModifyGraph rgb('DC1.SA03008H.20180718.000009')=(0,39424,65280)\nX ModifyGraph rgb('DC2.SA03008H.20180718.000009')=(0,20992,65280)\nX ModifyGraph rgb('DC3.SA03008H.20180718.000009')=(0,2560,65280)\nX ModifyGraph rgb('DC4.SA03008H.20180718.000009')=(17408,0,65280)\nX ModifyGraph rgb('DC5.SA03008H.20180718.000009')=(35840,0,65280)\nX ModifyGraph rgb('DC6.SA03008H.20180718.000009')=(54272,0,65280)\nX ModifyGraph rgb('DC7.SA03008H.20180718.000009')=(65280,0,58368)\nX Legend/C/N=text0/J \"\\\\s('time.SA03008H.20180718.000009') time\\r\\\\s('temp.SA03008H.20180718.000009') temp\\r\\\\s('B.SA03008H.20180718.000009') B\\r\\\\s('Vsource.SA03008H.20180718.000009') Vsource\\r\\\\s('Lockin0.SA03008H.20180718.000009') Lockin0\\r\\\\s('Lockin1.SA03008H.20180718.000009') Lockin1\\r\\\\s('Lockin2.SA03008H.20180718.000009') Lockin2\\r\\\\s('Lockin3.SA03008H.20180718.000009') Lockin3\\r\\\\s('Lockin4.SA03008H.20180718.000009') Lockin4\\r\\\\s('Lockin5.SA03008H.20180718.000009') Lockin5\\r\\\\s('B_rate.SA03008H.20180718.000009') B_rate\\r\\\\s('DC0.SA03008H.20180718.000009') DC0\\r\\\\s('DC1.SA03008H.20180718.000009') DC1\\r\\\\s('DC2.SA03008H.20180718.000009') DC2\\r\\\\s('DC3.SA03008H.20180718.000009') DC3\\r\\\\s('DC4.SA03008H.20180718.000009') DC4\\r\\\\s('DC5.SA03008H.20180718.000009') DC5\\r\\\\s('DC6.SA03008H.20180718.000009') DC6\\r\\\\s('DC7.SA03008H.20180718.000009') DC7\"\nX ModifyGraph mirror(bottom)=1\nX ModifyGraph width=216\nX ModifyGraph height={Aspect,0.6}\nX ModifyGraph Log(bottom)=0\nX ModifyGraph Log(left)=0\nX \n", "IGOR\nX// Date: 7/18/2018 5:20 PM\nX// SA03008H\nX// \nX// Source 2 Drain 28 (lockin 1 and 7)\nX// Slow sweeping BG -5 to 5 inc. 0.1V \nX// Fast sweep SG -1 to 1 inc. 0.05V\n\nX// DSA_Vsg1=-0.500000\n\nX// \nX// B= 0.000000\n\n\n\n\n\n\n\n\n\n\n\n\n\n\n\n\n\n\n\n\n\n\n\n\n\n\n\n\n\n\n\n\n\n\n\n\n\n\n\n\nX \nX Display/R 'time.SA03008H.20180718.000010'\nX AppendToGraph 'temp.SA03008H.20180718.000010'\nX AppendToGraph 'B.SA03008H.20180718.000010'\nX AppendToGraph 'Vsource.SA03008H.20180718.000010'\nX AppendToGraph 'Lockin0.SA03008H.20180718.000010'\nX AppendToGraph 'Lockin1.SA03008H.20180718.000010'\nX AppendToGraph 'Lockin2.SA03008H.20180718.000010'\nX AppendToGraph 'Lockin3.SA03008H.20180718.000010'\nX AppendToGraph 'Lockin4.SA03008H.20180718.000010'\nX AppendToGraph 'Lockin5.SA03008H.20180718.000010'\nX AppendToGraph 'B_rate.SA03008H.20180718.000010'\nX AppendToGraph 'DC0.SA03008H.20180718.000010'\nX AppendToGraph 'DC1.SA03008H.20180718.000010'\nX AppendToGraph 'DC2.SA03008H.20180718.000010'\nX AppendToGraph 'DC3.SA03008H.20180718.000010'\nX AppendToGraph 'DC4.SA03008H.20180718.000010'\nX AppendToGraph 'DC5.SA03008H.20180718.000010'\nX AppendToGraph 'DC6.SA03008H.20180718.000010'\nX AppendToGraph 'DC7.SA03008H.20180718.000010'\nX Label bottom \"x label\"\nX Label left \"y label\"\nX ModifyGraph rgb('time.SA03008H.20180718.000010')=(65280,0,0)\nX ModifyGraph rgb('temp.SA03008H.20180718.000010')=(65280,18432,0)\nX ModifyGraph rgb('B.SA03008H.20180718.000010')=(65280,36864,0)\nX ModifyGraph rgb('Vsource.SA03008H.20180718.000010')=(65280,55296,0)\nX ModifyGraph rgb('Lockin0.SA03008H.20180718.000010')=(57344,65280,0)\nX ModifyGraph rgb('Lockin1.SA03008H.20180718.000010')=(37376,65280,0)\nX ModifyGraph rgb('Lockin2.SA03008H.20180718.000010')=(18944,65280,0)\nX ModifyGraph rgb('Lockin3.SA03008H.20180718.000010')=(512,65280,0)\nX ModifyGraph rgb('Lockin4.SA03008H.20180718.000010')=(0,65280,17920)\nX ModifyGraph rgb('Lockin5.SA03008H.20180718.000010')=(0,65280,36352)\nX ModifyGraph rgb('B_rate.SA03008H.20180718.000010')=(0,65280,54784)\nX ModifyGraph rgb('DC0.SA03008H.20180718.000010')=(0,57856,65280)\nX ModifyGraph rgb('DC1.SA03008H.20180718.000010')=(0,39424,65280)\nX ModifyGraph rgb('DC2.SA03008H.20180718.000010')=(0,20992,65280)\nX ModifyGraph rgb('DC3.SA03008H.20180718.000010')=(0,2560,65280)\nX ModifyGraph rgb('DC4.SA03008H.20180718.000010')=(17408,0,65280)\nX ModifyGraph rgb('DC5.SA03008H.20180718.000010')=(35840,0,65280)\nX ModifyGraph rgb('DC6.SA03008H.20180718.000010')=(54272,0,65280)\nX ModifyGraph rgb('DC7.SA03008H.20180718.000010')=(65280,0,58368)\nX Legend/C/N=text0/J \"\\\\s('time.SA03008H.20180718.000010') time\\r\\\\s('temp.SA03008H.20180718.000010') temp\\r\\\\s('B.SA03008H.20180718.000010') B\\r\\\\s('Vsource.SA03008H.20180718.000010') Vsource\\r\\\\s('Lockin0.SA03008H.20180718.000010') Lockin0\\r\\\\s('Lockin1.SA03008H.20180718.000010') Lockin1\\r\\\\s('Lockin2.SA03008H.20180718.000010') Lockin2\\r\\\\s('Lockin3.SA03008H.20180718.000010') Lockin3\\r\\\\s('Lockin4.SA03008H.20180718.000010') Lockin4\\r\\\\s('Lockin5.SA03008H.20180718.000010') Lockin5\\r\\\\s('B_rate.SA03008H.20180718.000010') B_rate\\r\\\\s('DC0.SA03008H.20180718.000010') DC0\\r\\\\s('DC1.SA03008H.20180718.000010') DC1\\r\\\\s('DC2.SA03008H.20180718.000010') DC2\\r\\\\s('DC3.SA03008H.20180718.000010') DC3\\r\\\\s('DC4.SA03008H.20180718.000010') DC4\\r\\\\s('DC5.SA03008H.20180718.000010') DC5\\r\\\\s('DC6.SA03008H.20180718.000010') DC6\\r\\\\s('DC7.SA03008H.20180718.000010') DC7\"\nX ModifyGraph mirror(bottom)=1\nX ModifyGraph width=216\nX ModifyGraph height={Aspect,0.6}\nX ModifyGraph Log(bottom)=0\nX ModifyGraph Log(left)=0\nX \n", "IGOR\nX// Date: 7/18/2018 5:20 PM\nX// SA03008H\nX// \nX// Source 2 Drain 28 (lockin 1 and 7)\nX// Slow sweeping BG -5 to 5 inc. 0.1V \nX// Fast sweep SG -1 to 1 inc. 0.05V\n\nX// DSA_Vsg1=-0.450000\n\nX// \nX// B= 0.000000\n\n\n\n\n\n\n\n\n\n\n\n\n\n\n\n\n\n\n\n\n\n\n\n\n\n\n\n\n\n\n\n\n\n\n\n\n\n\n\n\nX \nX Display/R 'time.SA03008H.20180718.000011'\nX AppendToGraph 'temp.SA03008H.20180718.000011'\nX AppendToGraph 'B.SA03008H.20180718.000011'\nX AppendToGraph 'Vsource.SA03008H.20180718.000011'\nX AppendToGraph 'Lockin0.SA03008H.20180718.000011'\nX AppendToGraph 'Lockin1.SA03008H.20180718.000011'\nX AppendToGraph 'Lockin2.SA03008H.20180718.000011'\nX AppendToGraph 'Lockin3.SA03008H.20180718.000011'\nX AppendToGraph 'Lockin4.SA03008H.20180718.000011'\nX AppendToGraph 'Lockin5.SA03008H.20180718.000011'\nX AppendToGraph 'B_rate.SA03008H.20180718.000011'\nX AppendToGraph 'DC0.SA03008H.20180718.000011'\nX AppendToGraph 'DC1.SA03008H.20180718.000011'\nX AppendToGraph 'DC2.SA03008H.20180718.000011'\nX AppendToGraph 'DC3.SA03008H.20180718.000011'\nX AppendToGraph 'DC4.SA03008H.20180718.000011'\nX AppendToGraph 'DC5.SA03008H.20180718.000011'\nX AppendToGraph 'DC6.SA03008H.20180718.000011'\nX AppendToGraph 'DC7.SA03008H.20180718.000011'\nX Label bottom \"x label\"\nX Label left \"y label\"\nX ModifyGraph rgb('time.SA03008H.20180718.000011')=(65280,0,0)\nX ModifyGraph rgb('temp.SA03008H.20180718.000011')=(65280,18432,0)\nX ModifyGraph rgb('B.SA03008H.20180718.000011')=(65280,36864,0)\nX ModifyGraph rgb('Vsource.SA03008H.20180718.000011')=(65280,55296,0)\nX ModifyGraph rgb('Lockin0.SA03008H.20180718.000011')=(57344,65280,0)\nX ModifyGraph rgb('Lockin1.SA03008H.20180718.000011')=(37376,65280,0)\nX ModifyGraph rgb('Lockin2.SA03008H.20180718.000011')=(18944,65280,0)\nX ModifyGraph rgb('Lockin3.SA03008H.20180718.000011')=(512,65280,0)\nX ModifyGraph rgb('Lockin4.SA03008H.20180718.000011')=(0,65280,17920)\nX ModifyGraph rgb('Lockin5.SA03008H.20180718.000011')=(0,65280,36352)\nX ModifyGraph rgb('B_rate.SA03008H.20180718.000011')=(0,65280,54784)\nX ModifyGraph rgb('DC0.SA03008H.20180718.000011')=(0,57856,65280)\nX ModifyGraph rgb('DC1.SA03008H.20180718.000011')=(0,39424,65280)\nX ModifyGraph rgb('DC2.SA03008H.20180718.000011')=(0,20992,65280)\nX ModifyGraph rgb('DC3.SA03008H.20180718.000011')=(0,2560,65280)\nX ModifyGraph rgb('DC4.SA03008H.20180718.000011')=(17408,0,65280)\nX ModifyGraph rgb('DC5.SA03008H.20180718.000011')=(35840,0,65280)\nX ModifyGraph rgb('DC6.SA03008H.20180718.000011')=(54272,0,65280)\nX ModifyGraph rgb('DC7.SA03008H.20180718.000011')=(65280,0,58368)\nX Legend/C/N=text0/J \"\\\\s('time.SA03008H.20180718.000011') time\\r\\\\s('temp.SA03008H.20180718.000011') temp\\r\\\\s('B.SA03008H.20180718.000011') B\\r\\\\s('Vsource.SA03008H.20180718.000011') Vsource\\r\\\\s('Lockin0.SA03008H.20180718.000011') Lockin0\\r\\\\s('Lockin1.SA03008H.20180718.000011') Lockin1\\r\\\\s('Lockin2.SA03008H.20180718.000011') Lockin2\\r\\\\s('Lockin3.SA03008H.20180718.000011') Lockin3\\r\\\\s('Lockin4.SA03008H.20180718.000011') Lockin4\\r\\\\s('Lockin5.SA03008H.20180718.000011') Lockin5\\r\\\\s('B_rate.SA03008H.20180718.000011') B_rate\\r\\\\s('DC0.SA03008H.20180718.000011') DC0\\r\\\\s('DC1.SA03008H.20180718.000011') DC1\\r\\\\s('DC2.SA03008H.20180718.000011') DC2\\r\\\\s('DC3.SA03008H.20180718.000011') DC3\\r\\\\s('DC4.SA03008H.20180718.000011') DC4\\r\\\\s('DC5.SA03008H.20180718.000011') DC5\\r\\\\s('DC6.SA03008H.20180718.000011') DC6\\r\\\\s('DC7.SA03008H.20180718.000011') DC7\"\nX ModifyGraph mirror(bottom)=1\nX ModifyGraph width=216\nX ModifyGraph height={Aspect,0.6}\nX ModifyGraph Log(bottom)=0\nX ModifyGraph Log(left)=0\nX \n", "IGOR\nX// Date: 7/18/2018 5:21 PM\nX// SA03008H\nX// \nX// Source 2 Drain 28 (lockin 1 and 7)\nX// Slow sweeping BG -5 to 5 inc. 0.1V \nX// Fast sweep SG -1 to 1 inc. 0.05V\n\nX// DSA_Vsg1=-0.400000\n\nX// \nX// B= 0.000000\n\n\n\n\n\n\n\n\n\n\n\n\n\n\n\n\n\n\n\n\n\n\n\n\n\n\n\n\n\n\n\n\n\n\n\n\n\n\n\n\nX \nX Display/R 'time.SA03008H.20180718.000012'\nX AppendToGraph 'temp.SA03008H.20180718.000012'\nX AppendToGraph 'B.SA03008H.20180718.000012'\nX AppendToGraph 'Vsource.SA03008H.20180718.000012'\nX AppendToGraph 'Lockin0.SA03008H.20180718.000012'\nX AppendToGraph 'Lockin1.SA03008H.20180718.000012'\nX AppendToGraph 'Lockin2.SA03008H.20180718.000012'\nX AppendToGraph 'Lockin3.SA03008H.20180718.000012'\nX AppendToGraph 'Lockin4.SA03008H.20180718.000012'\nX AppendToGraph 'Lockin5.SA03008H.20180718.000012'\nX AppendToGraph 'B_rate.SA03008H.20180718.000012'\nX AppendToGraph 'DC0.SA03008H.20180718.000012'\nX AppendToGraph 'DC1.SA03008H.20180718.000012'\nX AppendToGraph 'DC2.SA03008H.20180718.000012'\nX AppendToGraph 'DC3.SA03008H.20180718.000012'\nX AppendToGraph 'DC4.SA03008H.20180718.000012'\nX AppendToGraph 'DC5.SA03008H.20180718.000012'\nX AppendToGraph 'DC6.SA03008H.20180718.000012'\nX AppendToGraph 'DC7.SA03008H.20180718.000012'\nX Label bottom \"x label\"\nX Label left \"y label\"\nX ModifyGraph rgb('time.SA03008H.20180718.000012')=(65280,0,0)\nX ModifyGraph rgb('temp.SA03008H.20180718.000012')=(65280,18432,0)\nX ModifyGraph rgb('B.SA03008H.20180718.000012')=(65280,36864,0)\nX ModifyGraph rgb('Vsource.SA03008H.20180718.000012')=(65280,55296,0)\nX ModifyGraph rgb('Lockin0.SA03008H.20180718.000012')=(57344,65280,0)\nX ModifyGraph rgb('Lockin1.SA03008H.20180718.000012')=(37376,65280,0)\nX ModifyGraph rgb('Lockin2.SA03008H.20180718.000012')=(18944,65280,0)\nX ModifyGraph rgb('Lockin3.SA03008H.20180718.000012')=(512,65280,0)\nX ModifyGraph rgb('Lockin4.SA03008H.20180718.000012')=(0,65280,17920)\nX ModifyGraph rgb('Lockin5.SA03008H.20180718.000012')=(0,65280,36352)\nX ModifyGraph rgb('B_rate.SA03008H.20180718.000012')=(0,65280,54784)\nX ModifyGraph rgb('DC0.SA03008H.20180718.000012')=(0,57856,65280)\nX ModifyGraph rgb('DC1.SA03008H.20180718.000012')=(0,39424,65280)\nX ModifyGraph rgb('DC2.SA03008H.20180718.000012')=(0,20992,65280)\nX ModifyGraph rgb('DC3.SA03008H.20180718.000012')=(0,2560,65280)\nX ModifyGraph rgb('DC4.SA03008H.20180718.000012')=(17408,0,65280)\nX ModifyGraph rgb('DC5.SA03008H.20180718.000012')=(35840,0,65280)\nX ModifyGraph rgb('DC6.SA03008H.20180718.000012')=(54272,0,65280)\nX ModifyGraph rgb('DC7.SA03008H.20180718.000012')=(65280,0,58368)\nX Legend/C/N=text0/J \"\\\\s('time.SA03008H.20180718.000012') time\\r\\\\s('temp.SA03008H.20180718.000012') temp\\r\\\\s('B.SA03008H.20180718.000012') B\\r\\\\s('Vsource.SA03008H.20180718.000012') Vsource\\r\\\\s('Lockin0.SA03008H.20180718.000012') Lockin0\\r\\\\s('Lockin1.SA03008H.20180718.000012') Lockin1\\r\\\\s('Lockin2.SA03008H.20180718.000012') Lockin2\\r\\\\s('Lockin3.SA03008H.20180718.000012') Lockin3\\r\\\\s('Lockin4.SA03008H.20180718.000012') Lockin4\\r\\\\s('Lockin5.SA03008H.20180718.000012') Lockin5\\r\\\\s('B_rate.SA03008H.20180718.000012') B_rate\\r\\\\s('DC0.SA03008H.20180718.000012') DC0\\r\\\\s('DC1.SA03008H.20180718.000012') DC1\\r\\\\s('DC2.SA03008H.20180718.000012') DC2\\r\\\\s('DC3.SA03008H.20180718.000012') DC3\\r\\\\s('DC4.SA03008H.20180718.000012') DC4\\r\\\\s('DC5.SA03008H.20180718.000012') DC5\\r\\\\s('DC6.SA03008H.20180718.000012') DC6\\r\\\\s('DC7.SA03008H.20180718.000012') DC7\"\nX ModifyGraph mirror(bottom)=1\nX ModifyGraph width=216\nX ModifyGraph height={Aspect,0.6}\nX ModifyGraph Log(bottom)=0\nX ModifyGraph Log(left)=0\nX \n", "IGOR\nX// Date: 7/18/2018 5:21 PM\nX// SA03008H\nX// \nX// Source 2 Drain 28 (lockin 1 and 7)\nX// Slow sweeping BG -5 to 5 inc. 0.1V \nX// Fast sweep SG -1 to 1 inc. 0.05V\n\nX// DSA_Vsg1=-0.350000\n\nX// \nX// B= 0.000000\n\n\n\n\n\n\n\n\n\n\n\n\n\n\n\n\n\n\n\n\n\n\n\n\n\n\n\n\n\n\n\n\n\n\n\n\n\n\n\n\nX \nX Display/R 'time.SA03008H.20180718.000013'\nX AppendToGraph 'temp.SA03008H.20180718.000013'\nX AppendToGraph 'B.SA03008H.20180718.000013'\nX AppendToGraph 'Vsource.SA03008H.20180718.000013'\nX AppendToGraph 'Lockin0.SA03008H.20180718.000013'\nX AppendToGraph 'Lockin1.SA03008H.20180718.000013'\nX AppendToGraph 'Lockin2.SA03008H.20180718.000013'\nX AppendToGraph 'Lockin3.SA03008H.20180718.000013'\nX AppendToGraph 'Lockin4.SA03008H.20180718.000013'\nX AppendToGraph 'Lockin5.SA03008H.20180718.000013'\nX AppendToGraph 'B_rate.SA03008H.20180718.000013'\nX AppendToGraph 'DC0.SA03008H.20180718.000013'\nX AppendToGraph 'DC1.SA03008H.20180718.000013'\nX AppendToGraph 'DC2.SA03008H.20180718.000013'\nX AppendToGraph 'DC3.SA03008H.20180718.000013'\nX AppendToGraph 'DC4.SA03008H.20180718.000013'\nX AppendToGraph 'DC5.SA03008H.20180718.000013'\nX AppendToGraph 'DC6.SA03008H.20180718.000013'\nX AppendToGraph 'DC7.SA03008H.20180718.000013'\nX Label bottom \"x label\"\nX Label left \"y label\"\nX ModifyGraph rgb('time.SA03008H.20180718.000013')=(65280,0,0)\nX ModifyGraph rgb('temp.SA03008H.20180718.000013')=(65280,18432,0)\nX ModifyGraph rgb('B.SA03008H.20180718.000013')=(65280,36864,0)\nX ModifyGraph rgb('Vsource.SA03008H.20180718.000013')=(65280,55296,0)\nX ModifyGraph rgb('Lockin0.SA03008H.20180718.000013')=(57344,65280,0)\nX ModifyGraph rgb('Lockin1.SA03008H.20180718.000013')=(37376,65280,0)\nX ModifyGraph rgb('Lockin2.SA03008H.20180718.000013')=(18944,65280,0)\nX ModifyGraph rgb('Lockin3.SA03008H.20180718.000013')=(512,65280,0)\nX ModifyGraph rgb('Lockin4.SA03008H.20180718.000013')=(0,65280,17920)\nX ModifyGraph rgb('Lockin5.SA03008H.20180718.000013')=(0,65280,36352)\nX ModifyGraph rgb('B_rate.SA03008H.20180718.000013')=(0,65280,54784)\nX ModifyGraph rgb('DC0.SA03008H.20180718.000013')=(0,57856,65280)\nX ModifyGraph rgb('DC1.SA03008H.20180718.000013')=(0,39424,65280)\nX ModifyGraph rgb('DC2.SA03008H.20180718.000013')=(0,20992,65280)\nX ModifyGraph rgb('DC3.SA03008H.20180718.000013')=(0,2560,65280)\nX ModifyGraph rgb('DC4.SA03008H.20180718.000013')=(17408,0,65280)\nX ModifyGraph rgb('DC5.SA03008H.20180718.000013')=(35840,0,65280)\nX ModifyGraph rgb('DC6.SA03008H.20180718.000013')=(54272,0,65280)\nX ModifyGraph rgb('DC7.SA03008H.20180718.000013')=(65280,0,58368)\nX Legend/C/N=text0/J \"\\\\s('time.SA03008H.20180718.000013') time\\r\\\\s('temp.SA03008H.20180718.000013') temp\\r\\\\s('B.SA03008H.20180718.000013') B\\r\\\\s('Vsource.SA03008H.20180718.000013') Vsource\\r\\\\s('Lockin0.SA03008H.20180718.000013') Lockin0\\r\\\\s('Lockin1.SA03008H.20180718.000013') Lockin1\\r\\\\s('Lockin2.SA03008H.20180718.000013') Lockin2\\r\\\\s('Lockin3.SA03008H.20180718.000013') Lockin3\\r\\\\s('Lockin4.SA03008H.20180718.000013') Lockin4\\r\\\\s('Lockin5.SA03008H.20180718.000013') Lockin5\\r\\\\s('B_rate.SA03008H.20180718.000013') B_rate\\r\\\\s('DC0.SA03008H.20180718.000013') DC0\\r\\\\s('DC1.SA03008H.20180718.000013') DC1\\r\\\\s('DC2.SA03008H.20180718.000013') DC2\\r\\\\s('DC3.SA03008H.20180718.000013') DC3\\r\\\\s('DC4.SA03008H.20180718.000013') DC4\\r\\\\s('DC5.SA03008H.20180718.000013') DC5\\r\\\\s('DC6.SA03008H.20180718.000013') DC6\\r\\\\s('DC7.SA03008H.20180718.000013') DC7\"\nX ModifyGraph mirror(bottom)=1\nX ModifyGraph width=216\nX ModifyGraph height={Aspect,0.6}\nX ModifyGraph Log(bottom)=0\nX ModifyGraph Log(left)=0\nX \n", "IGOR\nX// Date: 7/18/2018 5:21 PM\nX// SA03008H\nX// \nX// Source 2 Drain 28 (lockin 1 and 7)\nX// Slow sweeping BG -5 to 5 inc. 0.1V \nX// Fast sweep SG -1 to 1 inc. 0.05V\n\nX// DSA_Vsg1=-0.300000\n\nX// \nX// B= 0.000000\n\n\n\n\n\n\n\n\n\n\n\n\n\n\n\n\n\n\n\n\n\n\n\n\n\n\n\n\n\n\n\n\n\n\n\n\n\n\n\n\nX \nX Display/R 'time.SA03008H.20180718.000014'\nX AppendToGraph 'temp.SA03008H.20180718.000014'\nX AppendToGraph 'B.SA03008H.20180718.000014'\nX AppendToGraph 'Vsource.SA03008H.20180718.000014'\nX AppendToGraph 'Lockin0.SA03008H.20180718.000014'\nX AppendToGraph 'Lockin1.SA03008H.20180718.000014'\nX AppendToGraph 'Lockin2.SA03008H.20180718.000014'\nX AppendToGraph 'Lockin3.SA03008H.20180718.000014'\nX AppendToGraph 'Lockin4.SA03008H.20180718.000014'\nX AppendToGraph 'Lockin5.SA03008H.20180718.000014'\nX AppendToGraph 'B_rate.SA03008H.20180718.000014'\nX AppendToGraph 'DC0.SA03008H.20180718.000014'\nX AppendToGraph 'DC1.SA03008H.20180718.000014'\nX AppendToGraph 'DC2.SA03008H.20180718.000014'\nX AppendToGraph 'DC3.SA03008H.20180718.000014'\nX AppendToGraph 'DC4.SA03008H.20180718.000014'\nX AppendToGraph 'DC5.SA03008H.20180718.000014'\nX AppendToGraph 'DC6.SA03008H.20180718.000014'\nX AppendToGraph 'DC7.SA03008H.20180718.000014'\nX Label bottom \"x label\"\nX Label left \"y label\"\nX ModifyGraph rgb('time.SA03008H.20180718.000014')=(65280,0,0)\nX ModifyGraph rgb('temp.SA03008H.20180718.000014')=(65280,18432,0)\nX ModifyGraph rgb('B.SA03008H.20180718.000014')=(65280,36864,0)\nX ModifyGraph rgb('Vsource.SA03008H.20180718.000014')=(65280,55296,0)\nX ModifyGraph rgb('Lockin0.SA03008H.20180718.000014')=(57344,65280,0)\nX ModifyGraph rgb('Lockin1.SA03008H.20180718.000014')=(37376,65280,0)\nX ModifyGraph rgb('Lockin2.SA03008H.20180718.000014')=(18944,65280,0)\nX ModifyGraph rgb('Lockin3.SA03008H.20180718.000014')=(512,65280,0)\nX ModifyGraph rgb('Lockin4.SA03008H.20180718.000014')=(0,65280,17920)\nX ModifyGraph rgb('Lockin5.SA03008H.20180718.000014')=(0,65280,36352)\nX ModifyGraph rgb('B_rate.SA03008H.20180718.000014')=(0,65280,54784)\nX ModifyGraph rgb('DC0.SA03008H.20180718.000014')=(0,57856,65280)\nX ModifyGraph rgb('DC1.SA03008H.20180718.000014')=(0,39424,65280)\nX ModifyGraph rgb('DC2.SA03008H.20180718.000014')=(0,20992,65280)\nX ModifyGraph rgb('DC3.SA03008H.20180718.000014')=(0,2560,65280)\nX ModifyGraph rgb('DC4.SA03008H.20180718.000014')=(17408,0,65280)\nX ModifyGraph rgb('DC5.SA03008H.20180718.000014')=(35840,0,65280)\nX ModifyGraph rgb('DC6.SA03008H.20180718.000014')=(54272,0,65280)\nX ModifyGraph rgb('DC7.SA03008H.20180718.000014')=(65280,0,58368)\nX Legend/C/N=text0/J \"\\\\s('time.SA03008H.20180718.000014') time\\r\\\\s('temp.SA03008H.20180718.000014') temp\\r\\\\s('B.SA03008H.20180718.000014') B\\r\\\\s('Vsource.SA03008H.20180718.000014') Vsource\\r\\\\s('Lockin0.SA03008H.20180718.000014') Lockin0\\r\\\\s('Lockin1.SA03008H.20180718.000014') Lockin1\\r\\\\s('Lockin2.SA03008H.20180718.000014') Lockin2\\r\\\\s('Lockin3.SA03008H.20180718.000014') Lockin3\\r\\\\s('Lockin4.SA03008H.20180718.000014') Lockin4\\r\\\\s('Lockin5.SA03008H.20180718.000014') Lockin5\\r\\\\s('B_rate.SA03008H.20180718.000014') B_rate\\r\\\\s('DC0.SA03008H.20180718.000014') DC0\\r\\\\s('DC1.SA03008H.20180718.000014') DC1\\r\\\\s('DC2.SA03008H.20180718.000014') DC2\\r\\\\s('DC3.SA03008H.20180718.000014') DC3\\r\\\\s('DC4.SA03008H.20180718.000014') DC4\\r\\\\s('DC5.SA03008H.20180718.000014') DC5\\r\\\\s('DC6.SA03008H.20180718.000014') DC6\\r\\\\s('DC7.SA03008H.20180718.000014') DC7\"\nX ModifyGraph mirror(bottom)=1\nX ModifyGraph width=216\nX ModifyGraph height={Aspect,0.6}\nX ModifyGraph Log(bottom)=0\nX ModifyGraph Log(left)=0\nX \n", "IGOR\nX// Date: 7/18/2018 5:21 PM\nX// SA03008H\nX// \nX// Source 2 Drain 28 (lockin 1 and 7)\nX// Slow sweeping BG -5 to 5 inc. 0.1V \nX// Fast sweep SG -1 to 1 inc. 0.05V\n\nX// DSA_Vsg1=-0.250000\n\nX// \nX// B= 0.000000\n\n\n\n\n\n\n\n\n\n\n\n\n\n\n\n\n\n\n\n\n\n\n\n\n\n\n\n\n\n\n\n\n\n\n\n\n\n\n\n\nX \nX Display/R 'time.SA03008H.20180718.000015'\nX AppendToGraph 'temp.SA03008H.20180718.000015'\nX AppendToGraph 'B.SA03008H.20180718.000015'\nX AppendToGraph 'Vsource.SA03008H.20180718.000015'\nX AppendToGraph 'Lockin0.SA03008H.20180718.000015'\nX AppendToGraph 'Lockin1.SA03008H.20180718.000015'\nX AppendToGraph 'Lockin2.SA03008H.20180718.000015'\nX AppendToGraph 'Lockin3.SA03008H.20180718.000015'\nX AppendToGraph 'Lockin4.SA03008H.20180718.000015'\nX AppendToGraph 'Lockin5.SA03008H.20180718.000015'\nX AppendToGraph 'B_rate.SA03008H.20180718.000015'\nX AppendToGraph 'DC0.SA03008H.20180718.000015'\nX AppendToGraph 'DC1.SA03008H.20180718.000015'\nX AppendToGraph 'DC2.SA03008H.20180718.000015'\nX AppendToGraph 'DC3.SA03008H.20180718.000015'\nX AppendToGraph 'DC4.SA03008H.20180718.000015'\nX AppendToGraph 'DC5.SA03008H.20180718.000015'\nX AppendToGraph 'DC6.SA03008H.20180718.000015'\nX AppendToGraph 'DC7.SA03008H.20180718.000015'\nX Label bottom \"x label\"\nX Label left \"y label\"\nX ModifyGraph rgb('time.SA03008H.20180718.000015')=(65280,0,0)\nX ModifyGraph rgb('temp.SA03008H.20180718.000015')=(65280,18432,0)\nX ModifyGraph rgb('B.SA03008H.20180718.000015')=(65280,36864,0)\nX ModifyGraph rgb('Vsource.SA03008H.20180718.000015')=(65280,55296,0)\nX ModifyGraph rgb('Lockin0.SA03008H.20180718.000015')=(57344,65280,0)\nX ModifyGraph rgb('Lockin1.SA03008H.20180718.000015')=(37376,65280,0)\nX ModifyGraph rgb('Lockin2.SA03008H.20180718.000015')=(18944,65280,0)\nX ModifyGraph rgb('Lockin3.SA03008H.20180718.000015')=(512,65280,0)\nX ModifyGraph rgb('Lockin4.SA03008H.20180718.000015')=(0,65280,17920)\nX ModifyGraph rgb('Lockin5.SA03008H.20180718.000015')=(0,65280,36352)\nX ModifyGraph rgb('B_rate.SA03008H.20180718.000015')=(0,65280,54784)\nX ModifyGraph rgb('DC0.SA03008H.20180718.000015')=(0,57856,65280)\nX ModifyGraph rgb('DC1.SA03008H.20180718.000015')=(0,39424,65280)\nX ModifyGraph rgb('DC2.SA03008H.20180718.000015')=(0,20992,65280)\nX ModifyGraph rgb('DC3.SA03008H.20180718.000015')=(0,2560,65280)\nX ModifyGraph rgb('DC4.SA03008H.20180718.000015')=(17408,0,65280)\nX ModifyGraph rgb('DC5.SA03008H.20180718.000015')=(35840,0,65280)\nX ModifyGraph rgb('DC6.SA03008H.20180718.000015')=(54272,0,65280)\nX ModifyGraph rgb('DC7.SA03008H.20180718.000015')=(65280,0,58368)\nX Legend/C/N=text0/J \"\\\\s('time.SA03008H.20180718.000015') time\\r\\\\s('temp.SA03008H.20180718.000015') temp\\r\\\\s('B.SA03008H.20180718.000015') B\\r\\\\s('Vsource.SA03008H.20180718.000015') Vsource\\r\\\\s('Lockin0.SA03008H.20180718.000015') Lockin0\\r\\\\s('Lockin1.SA03008H.20180718.000015') Lockin1\\r\\\\s('Lockin2.SA03008H.20180718.000015') Lockin2\\r\\\\s('Lockin3.SA03008H.20180718.000015') Lockin3\\r\\\\s('Lockin4.SA03008H.20180718.000015') Lockin4\\r\\\\s('Lockin5.SA03008H.20180718.000015') Lockin5\\r\\\\s('B_rate.SA03008H.20180718.000015') B_rate\\r\\\\s('DC0.SA03008H.20180718.000015') DC0\\r\\\\s('DC1.SA03008H.20180718.000015') DC1\\r\\\\s('DC2.SA03008H.20180718.000015') DC2\\r\\\\s('DC3.SA03008H.20180718.000015') DC3\\r\\\\s('DC4.SA03008H.20180718.000015') DC4\\r\\\\s('DC5.SA03008H.20180718.000015') DC5\\r\\\\s('DC6.SA03008H.20180718.000015') DC6\\r\\\\s('DC7.SA03008H.20180718.000015') DC7\"\nX ModifyGraph mirror(bottom)=1\nX ModifyGraph width=216\nX ModifyGraph height={Aspect,0.6}\nX ModifyGraph Log(bottom)=0\nX ModifyGraph Log(left)=0\nX \n", "IGOR\nX// Date: 7/18/2018 5:21 PM\nX// SA03008H\nX// \nX// Source 2 Drain 28 (lockin 1 and 7)\nX// Slow sweeping BG -5 to 5 inc. 0.1V \nX// Fast sweep SG -1 to 1 inc. 0.05V\n\nX// DSA_Vsg1=-0.200000\n\nX// \nX// B= 0.000000\n\n\n\n\n\n\n\n\n\n\n\n\n\n\n\n\n\n\n\n\n\n\n\n\n\n\n\n\n\n\n\n\n\n\n\n\n\n\n\n\nX \nX Display/R 'time.SA03008H.20180718.000016'\nX AppendToGraph 'temp.SA03008H.20180718.000016'\nX AppendToGraph 'B.SA03008H.20180718.000016'\nX AppendToGraph 'Vsource.SA03008H.20180718.000016'\nX AppendToGraph 'Lockin0.SA03008H.20180718.000016'\nX AppendToGraph 'Lockin1.SA03008H.20180718.000016'\nX AppendToGraph 'Lockin2.SA03008H.20180718.000016'\nX AppendToGraph 'Lockin3.SA03008H.20180718.000016'\nX AppendToGraph 'Lockin4.SA03008H.20180718.000016'\nX AppendToGraph 'Lockin5.SA03008H.20180718.000016'\nX AppendToGraph 'B_rate.SA03008H.20180718.000016'\nX AppendToGraph 'DC0.SA03008H.20180718.000016'\nX AppendToGraph 'DC1.SA03008H.20180718.000016'\nX AppendToGraph 'DC2.SA03008H.20180718.000016'\nX AppendToGraph 'DC3.SA03008H.20180718.000016'\nX AppendToGraph 'DC4.SA03008H.20180718.000016'\nX AppendToGraph 'DC5.SA03008H.20180718.000016'\nX AppendToGraph 'DC6.SA03008H.20180718.000016'\nX AppendToGraph 'DC7.SA03008H.20180718.000016'\nX Label bottom \"x label\"\nX Label left \"y label\"\nX ModifyGraph rgb('time.SA03008H.20180718.000016')=(65280,0,0)\nX ModifyGraph rgb('temp.SA03008H.20180718.000016')=(65280,18432,0)\nX ModifyGraph rgb('B.SA03008H.20180718.000016')=(65280,36864,0)\nX ModifyGraph rgb('Vsource.SA03008H.20180718.000016')=(65280,55296,0)\nX ModifyGraph rgb('Lockin0.SA03008H.20180718.000016')=(57344,65280,0)\nX ModifyGraph rgb('Lockin1.SA03008H.20180718.000016')=(37376,65280,0)\nX ModifyGraph rgb('Lockin2.SA03008H.20180718.000016')=(18944,65280,0)\nX ModifyGraph rgb('Lockin3.SA03008H.20180718.000016')=(512,65280,0)\nX ModifyGraph rgb('Lockin4.SA03008H.20180718.000016')=(0,65280,17920)\nX ModifyGraph rgb('Lockin5.SA03008H.20180718.000016')=(0,65280,36352)\nX ModifyGraph rgb('B_rate.SA03008H.20180718.000016')=(0,65280,54784)\nX ModifyGraph rgb('DC0.SA03008H.20180718.000016')=(0,57856,65280)\nX ModifyGraph rgb('DC1.SA03008H.20180718.000016')=(0,39424,65280)\nX ModifyGraph rgb('DC2.SA03008H.20180718.000016')=(0,20992,65280)\nX ModifyGraph rgb('DC3.SA03008H.20180718.000016')=(0,2560,65280)\nX ModifyGraph rgb('DC4.SA03008H.20180718.000016')=(17408,0,65280)\nX ModifyGraph rgb('DC5.SA03008H.20180718.000016')=(35840,0,65280)\nX ModifyGraph rgb('DC6.SA03008H.20180718.000016')=(54272,0,65280)\nX ModifyGraph rgb('DC7.SA03008H.20180718.000016')=(65280,0,58368)\nX Legend/C/N=text0/J \"\\\\s('time.SA03008H.20180718.000016') time\\r\\\\s('temp.SA03008H.20180718.000016') temp\\r\\\\s('B.SA03008H.20180718.000016') B\\r\\\\s('Vsource.SA03008H.20180718.000016') Vsource\\r\\\\s('Lockin0.SA03008H.20180718.000016') Lockin0\\r\\\\s('Lockin1.SA03008H.20180718.000016') Lockin1\\r\\\\s('Lockin2.SA03008H.20180718.000016') Lockin2\\r\\\\s('Lockin3.SA03008H.20180718.000016') Lockin3\\r\\\\s('Lockin4.SA03008H.20180718.000016') Lockin4\\r\\\\s('Lockin5.SA03008H.20180718.000016') Lockin5\\r\\\\s('B_rate.SA03008H.20180718.000016') B_rate\\r\\\\s('DC0.SA03008H.20180718.000016') DC0\\r\\\\s('DC1.SA03008H.20180718.000016') DC1\\r\\\\s('DC2.SA03008H.20180718.000016') DC2\\r\\\\s('DC3.SA03008H.20180718.000016') DC3\\r\\\\s('DC4.SA03008H.20180718.000016') DC4\\r\\\\s('DC5.SA03008H.20180718.000016') DC5\\r\\\\s('DC6.SA03008H.20180718.000016') DC6\\r\\\\s('DC7.SA03008H.20180718.000016') DC7\"\nX ModifyGraph mirror(bottom)=1\nX ModifyGraph width=216\nX ModifyGraph height={Aspect,0.6}\nX ModifyGraph Log(bottom)=0\nX ModifyGraph Log(left)=0\nX \n", "IGOR\nX// Date: 7/18/2018 5:22 PM\nX// SA03008H\nX// \nX// Source 2 Drain 28 (lockin 1 and 7)\nX// Slow sweeping BG -5 to 5 inc. 0.1V \nX// Fast sweep SG -1 to 1 inc. 0.05V\n\nX// DSA_Vsg1=-0.150000\n\nX// \nX// B= 0.000000\n\n\n\n\n\n\n\n\n\n\n\n\n\n\n\n\n\n\n\n\n\n\n\n\n\n\n\n\n\n\n\n\n\n\n\n\n\n\n\n\nX \nX Display/R 'time.SA03008H.20180718.000017'\nX AppendToGraph 'temp.SA03008H.20180718.000017'\nX AppendToGraph 'B.SA03008H.20180718.000017'\nX AppendToGraph 'Vsource.SA03008H.20180718.000017'\nX AppendToGraph 'Lockin0.SA03008H.20180718.000017'\nX AppendToGraph 'Lockin1.SA03008H.20180718.000017'\nX AppendToGraph 'Lockin2.SA03008H.20180718.000017'\nX AppendToGraph 'Lockin3.SA03008H.20180718.000017'\nX AppendToGraph 'Lockin4.SA03008H.20180718.000017'\nX AppendToGraph 'Lockin5.SA03008H.20180718.000017'\nX AppendToGraph 'B_rate.SA03008H.20180718.000017'\nX AppendToGraph 'DC0.SA03008H.20180718.000017'\nX AppendToGraph 'DC1.SA03008H.20180718.000017'\nX AppendToGraph 'DC2.SA03008H.20180718.000017'\nX AppendToGraph 'DC3.SA03008H.20180718.000017'\nX AppendToGraph 'DC4.SA03008H.20180718.000017'\nX AppendToGraph 'DC5.SA03008H.20180718.000017'\nX AppendToGraph 'DC6.SA03008H.20180718.000017'\nX AppendToGraph 'DC7.SA03008H.20180718.000017'\nX Label bottom \"x label\"\nX Label left \"y label\"\nX ModifyGraph rgb('time.SA03008H.20180718.000017')=(65280,0,0)\nX ModifyGraph rgb('temp.SA03008H.20180718.000017')=(65280,18432,0)\nX ModifyGraph rgb('B.SA03008H.20180718.000017')=(65280,36864,0)\nX ModifyGraph rgb('Vsource.SA03008H.20180718.000017')=(65280,55296,0)\nX ModifyGraph rgb('Lockin0.SA03008H.20180718.000017')=(57344,65280,0)\nX ModifyGraph rgb('Lockin1.SA03008H.20180718.000017')=(37376,65280,0)\nX ModifyGraph rgb('Lockin2.SA03008H.20180718.000017')=(18944,65280,0)\nX ModifyGraph rgb('Lockin3.SA03008H.20180718.000017')=(512,65280,0)\nX ModifyGraph rgb('Lockin4.SA03008H.20180718.000017')=(0,65280,17920)\nX ModifyGraph rgb('Lockin5.SA03008H.20180718.000017')=(0,65280,36352)\nX ModifyGraph rgb('B_rate.SA03008H.20180718.000017')=(0,65280,54784)\nX ModifyGraph rgb('DC0.SA03008H.20180718.000017')=(0,57856,65280)\nX ModifyGraph rgb('DC1.SA03008H.20180718.000017')=(0,39424,65280)\nX ModifyGraph rgb('DC2.SA03008H.20180718.000017')=(0,20992,65280)\nX ModifyGraph rgb('DC3.SA03008H.20180718.000017')=(0,2560,65280)\nX ModifyGraph rgb('DC4.SA03008H.20180718.000017')=(17408,0,65280)\nX ModifyGraph rgb('DC5.SA03008H.20180718.000017')=(35840,0,65280)\nX ModifyGraph rgb('DC6.SA03008H.20180718.000017')=(54272,0,65280)\nX ModifyGraph rgb('DC7.SA03008H.20180718.000017')=(65280,0,58368)\nX Legend/C/N=text0/J \"\\\\s('time.SA03008H.20180718.000017') time\\r\\\\s('temp.SA03008H.20180718.000017') temp\\r\\\\s('B.SA03008H.20180718.000017') B\\r\\\\s('Vsource.SA03008H.20180718.000017') Vsource\\r\\\\s('Lockin0.SA03008H.20180718.000017') Lockin0\\r\\\\s('Lockin1.SA03008H.20180718.000017') Lockin1\\r\\\\s('Lockin2.SA03008H.20180718.000017') Lockin2\\r\\\\s('Lockin3.SA03008H.20180718.000017') Lockin3\\r\\\\s('Lockin4.SA03008H.20180718.000017') Lockin4\\r\\\\s('Lockin5.SA03008H.20180718.000017') Lockin5\\r\\\\s('B_rate.SA03008H.20180718.000017') B_rate\\r\\\\s('DC0.SA03008H.20180718.000017') DC0\\r\\\\s('DC1.SA03008H.20180718.000017') DC1\\r\\\\s('DC2.SA03008H.20180718.000017') DC2\\r\\\\s('DC3.SA03008H.20180718.000017') DC3\\r\\\\s('DC4.SA03008H.20180718.000017') DC4\\r\\\\s('DC5.SA03008H.20180718.000017') DC5\\r\\\\s('DC6.SA03008H.20180718.000017') DC6\\r\\\\s('DC7.SA03008H.20180718.000017') DC7\"\nX ModifyGraph mirror(bottom)=1\nX ModifyGraph width=216\nX ModifyGraph height={Aspect,0.6}\nX ModifyGraph Log(bottom)=0\nX ModifyGraph Log(left)=0\nX \n", "IGOR\nX// Date: 7/18/2018 5:22 PM\nX// SA03008H\nX// \nX// Source 2 Drain 28 (lockin 1 and 7)\nX// Slow sweeping BG -5 to 5 inc. 0.1V \nX// Fast sweep SG -1 to 1 inc. 0.05V\n\nX// DSA_Vsg1=-0.100000\n\nX// \nX// B= 0.000000\n\n\n\n\n\n\n\n\n\n\n\n\n\n\n\n\n\n\n\n\n\n\n\n\n\n\n\n\n\n\n\n\n\n\n\n\n\n\n\n\nX \nX Display/R 'time.SA03008H.20180718.000018'\nX AppendToGraph 'temp.SA03008H.20180718.000018'\nX AppendToGraph 'B.SA03008H.20180718.000018'\nX AppendToGraph 'Vsource.SA03008H.20180718.000018'\nX AppendToGraph 'Lockin0.SA03008H.20180718.000018'\nX AppendToGraph 'Lockin1.SA03008H.20180718.000018'\nX AppendToGraph 'Lockin2.SA03008H.20180718.000018'\nX AppendToGraph 'Lockin3.SA03008H.20180718.000018'\nX AppendToGraph 'Lockin4.SA03008H.20180718.000018'\nX AppendToGraph 'Lockin5.SA03008H.20180718.000018'\nX AppendToGraph 'B_rate.SA03008H.20180718.000018'\nX AppendToGraph 'DC0.SA03008H.20180718.000018'\nX AppendToGraph 'DC1.SA03008H.20180718.000018'\nX AppendToGraph 'DC2.SA03008H.20180718.000018'\nX AppendToGraph 'DC3.SA03008H.20180718.000018'\nX AppendToGraph 'DC4.SA03008H.20180718.000018'\nX AppendToGraph 'DC5.SA03008H.20180718.000018'\nX AppendToGraph 'DC6.SA03008H.20180718.000018'\nX AppendToGraph 'DC7.SA03008H.20180718.000018'\nX Label bottom \"x label\"\nX Label left \"y label\"\nX ModifyGraph rgb('time.SA03008H.20180718.000018')=(65280,0,0)\nX ModifyGraph rgb('temp.SA03008H.20180718.000018')=(65280,18432,0)\nX ModifyGraph rgb('B.SA03008H.20180718.000018')=(65280,36864,0)\nX ModifyGraph rgb('Vsource.SA03008H.20180718.000018')=(65280,55296,0)\nX ModifyGraph rgb('Lockin0.SA03008H.20180718.000018')=(57344,65280,0)\nX ModifyGraph rgb('Lockin1.SA03008H.20180718.000018')=(37376,65280,0)\nX ModifyGraph rgb('Lockin2.SA03008H.20180718.000018')=(18944,65280,0)\nX ModifyGraph rgb('Lockin3.SA03008H.20180718.000018')=(512,65280,0)\nX ModifyGraph rgb('Lockin4.SA03008H.20180718.000018')=(0,65280,17920)\nX ModifyGraph rgb('Lockin5.SA03008H.20180718.000018')=(0,65280,36352)\nX ModifyGraph rgb('B_rate.SA03008H.20180718.000018')=(0,65280,54784)\nX ModifyGraph rgb('DC0.SA03008H.20180718.000018')=(0,57856,65280)\nX ModifyGraph rgb('DC1.SA03008H.20180718.000018')=(0,39424,65280)\nX ModifyGraph rgb('DC2.SA03008H.20180718.000018')=(0,20992,65280)\nX ModifyGraph rgb('DC3.SA03008H.20180718.000018')=(0,2560,65280)\nX ModifyGraph rgb('DC4.SA03008H.20180718.000018')=(17408,0,65280)\nX ModifyGraph rgb('DC5.SA03008H.20180718.000018')=(35840,0,65280)\nX ModifyGraph rgb('DC6.SA03008H.20180718.000018')=(54272,0,65280)\nX ModifyGraph rgb('DC7.SA03008H.20180718.000018')=(65280,0,58368)\nX Legend/C/N=text0/J \"\\\\s('time.SA03008H.20180718.000018') time\\r\\\\s('temp.SA03008H.20180718.000018') temp\\r\\\\s('B.SA03008H.20180718.000018') B\\r\\\\s('Vsource.SA03008H.20180718.000018') Vsource\\r\\\\s('Lockin0.SA03008H.20180718.000018') Lockin0\\r\\\\s('Lockin1.SA03008H.20180718.000018') Lockin1\\r\\\\s('Lockin2.SA03008H.20180718.000018') Lockin2\\r\\\\s('Lockin3.SA03008H.20180718.000018') Lockin3\\r\\\\s('Lockin4.SA03008H.20180718.000018') Lockin4\\r\\\\s('Lockin5.SA03008H.20180718.000018') Lockin5\\r\\\\s('B_rate.SA03008H.20180718.000018') B_rate\\r\\\\s('DC0.SA03008H.20180718.000018') DC0\\r\\\\s('DC1.SA03008H.20180718.000018') DC1\\r\\\\s('DC2.SA03008H.20180718.000018') DC2\\r\\\\s('DC3.SA03008H.20180718.000018') DC3\\r\\\\s('DC4.SA03008H.20180718.000018') DC4\\r\\\\s('DC5.SA03008H.20180718.000018') DC5\\r\\\\s('DC6.SA03008H.20180718.000018') DC6\\r\\\\s('DC7.SA03008H.20180718.000018') DC7\"\nX ModifyGraph mirror(bottom)=1\nX ModifyGraph width=216\nX ModifyGraph height={Aspect,0.6}\nX ModifyGraph Log(bottom)=0\nX ModifyGraph Log(left)=0\nX \n", "IGOR\nX// Date: 7/18/2018 5:22 PM\nX// SA03008H\nX// \nX// Source 2 Drain 28 (lockin 1 and 7)\nX// Slow sweeping BG -5 to 5 inc. 0.1V \nX// Fast sweep SG -1 to 1 inc. 0.05V\n\nX// DSA_Vsg1=-0.050000\n\nX// \nX// B= 0.000000\n\n\n\n\n\n\n\n\n\n\n\n\n\n\n\n\n\n\n\n\n\n\n\n\n\n\n\n\n\n\n\n\n\n\n\n\n\n\n\n\nX \nX Display/R 'time.SA03008H.20180718.000019'\nX AppendToGraph 'temp.SA03008H.20180718.000019'\nX AppendToGraph 'B.SA03008H.20180718.000019'\nX AppendToGraph 'Vsource.SA03008H.20180718.000019'\nX AppendToGraph 'Lockin0.SA03008H.20180718.000019'\nX AppendToGraph 'Lockin1.SA03008H.20180718.000019'\nX AppendToGraph 'Lockin2.SA03008H.20180718.000019'\nX AppendToGraph 'Lockin3.SA03008H.20180718.000019'\nX AppendToGraph 'Lockin4.SA03008H.20180718.000019'\nX AppendToGraph 'Lockin5.SA03008H.20180718.000019'\nX AppendToGraph 'B_rate.SA03008H.20180718.000019'\nX AppendToGraph 'DC0.SA03008H.20180718.000019'\nX AppendToGraph 'DC1.SA03008H.20180718.000019'\nX AppendToGraph 'DC2.SA03008H.20180718.000019'\nX AppendToGraph 'DC3.SA03008H.20180718.000019'\nX AppendToGraph 'DC4.SA03008H.20180718.000019'\nX AppendToGraph 'DC5.SA03008H.20180718.000019'\nX AppendToGraph 'DC6.SA03008H.20180718.000019'\nX AppendToGraph 'DC7.SA03008H.20180718.000019'\nX Label bottom \"x label\"\nX Label left \"y label\"\nX ModifyGraph rgb('time.SA03008H.20180718.000019')=(65280,0,0)\nX ModifyGraph rgb('temp.SA03008H.20180718.000019')=(65280,18432,0)\nX ModifyGraph rgb('B.SA03008H.20180718.000019')=(65280,36864,0)\nX ModifyGraph rgb('Vsource.SA03008H.20180718.000019')=(65280,55296,0)\nX ModifyGraph rgb('Lockin0.SA03008H.20180718.000019')=(57344,65280,0)\nX ModifyGraph rgb('Lockin1.SA03008H.20180718.000019')=(37376,65280,0)\nX ModifyGraph rgb('Lockin2.SA03008H.20180718.000019')=(18944,65280,0)\nX ModifyGraph rgb('Lockin3.SA03008H.20180718.000019')=(512,65280,0)\nX ModifyGraph rgb('Lockin4.SA03008H.20180718.000019')=(0,65280,17920)\nX ModifyGraph rgb('Lockin5.SA03008H.20180718.000019')=(0,65280,36352)\nX ModifyGraph rgb('B_rate.SA03008H.20180718.000019')=(0,65280,54784)\nX ModifyGraph rgb('DC0.SA03008H.20180718.000019')=(0,57856,65280)\nX ModifyGraph rgb('DC1.SA03008H.20180718.000019')=(0,39424,65280)\nX ModifyGraph rgb('DC2.SA03008H.20180718.000019')=(0,20992,65280)\nX ModifyGraph rgb('DC3.SA03008H.20180718.000019')=(0,2560,65280)\nX ModifyGraph rgb('DC4.SA03008H.20180718.000019')=(17408,0,65280)\nX ModifyGraph rgb('DC5.SA03008H.20180718.000019')=(35840,0,65280)\nX ModifyGraph rgb('DC6.SA03008H.20180718.000019')=(54272,0,65280)\nX ModifyGraph rgb('DC7.SA03008H.20180718.000019')=(65280,0,58368)\nX Legend/C/N=text0/J \"\\\\s('time.SA03008H.20180718.000019') time\\r\\\\s('temp.SA03008H.20180718.000019') temp\\r\\\\s('B.SA03008H.20180718.000019') B\\r\\\\s('Vsource.SA03008H.20180718.000019') Vsource\\r\\\\s('Lockin0.SA03008H.20180718.000019') Lockin0\\r\\\\s('Lockin1.SA03008H.20180718.000019') Lockin1\\r\\\\s('Lockin2.SA03008H.20180718.000019') Lockin2\\r\\\\s('Lockin3.SA03008H.20180718.000019') Lockin3\\r\\\\s('Lockin4.SA03008H.20180718.000019') Lockin4\\r\\\\s('Lockin5.SA03008H.20180718.000019') Lockin5\\r\\\\s('B_rate.SA03008H.20180718.000019') B_rate\\r\\\\s('DC0.SA03008H.20180718.000019') DC0\\r\\\\s('DC1.SA03008H.20180718.000019') DC1\\r\\\\s('DC2.SA03008H.20180718.000019') DC2\\r\\\\s('DC3.SA03008H.20180718.000019') DC3\\r\\\\s('DC4.SA03008H.20180718.000019') DC4\\r\\\\s('DC5.SA03008H.20180718.000019') DC5\\r\\\\s('DC6.SA03008H.20180718.000019') DC6\\r\\\\s('DC7.SA03008H.20180718.000019') DC7\"\nX ModifyGraph mirror(bottom)=1\nX ModifyGraph width=216\nX ModifyGraph height={Aspect,0.6}\nX ModifyGraph Log(bottom)=0\nX ModifyGraph Log(left)=0\nX \n", "IGOR\nX// Date: 7/18/2018 5:22 PM\nX// SA03008H\nX// \nX// Source 2 Drain 28 (lockin 1 and 7)\nX// Slow sweeping BG -5 to 5 inc. 0.1V \nX// Fast sweep SG -1 to 1 inc. 0.05V\n\nX// DSA_Vsg1=0.000000\n\nX// \nX// B= 0.000000\n\n\n\n\n\n\n\n\n\n\n\n\n\n\n\n\n\n\n\n\n\n\n\n\n\n\n\n\n\n\n\n\n\n\n\n\n\n\n\n\nX \nX Display/R 'time.SA03008H.20180718.000020'\nX AppendToGraph 'temp.SA03008H.20180718.000020'\nX AppendToGraph 'B.SA03008H.20180718.000020'\nX AppendToGraph 'Vsource.SA03008H.20180718.000020'\nX AppendToGraph 'Lockin0.SA03008H.20180718.000020'\nX AppendToGraph 'Lockin1.SA03008H.20180718.000020'\nX AppendToGraph 'Lockin2.SA03008H.20180718.000020'\nX AppendToGraph 'Lockin3.SA03008H.20180718.000020'\nX AppendToGraph 'Lockin4.SA03008H.20180718.000020'\nX AppendToGraph 'Lockin5.SA03008H.20180718.000020'\nX AppendToGraph 'B_rate.SA03008H.20180718.000020'\nX AppendToGraph 'DC0.SA03008H.20180718.000020'\nX AppendToGraph 'DC1.SA03008H.20180718.000020'\nX AppendToGraph 'DC2.SA03008H.20180718.000020'\nX AppendToGraph 'DC3.SA03008H.20180718.000020'\nX AppendToGraph 'DC4.SA03008H.20180718.000020'\nX AppendToGraph 'DC5.SA03008H.20180718.000020'\nX AppendToGraph 'DC6.SA03008H.20180718.000020'\nX AppendToGraph 'DC7.SA03008H.20180718.000020'\nX Label bottom \"x label\"\nX Label left \"y label\"\nX ModifyGraph rgb('time.SA03008H.20180718.000020')=(65280,0,0)\nX ModifyGraph rgb('temp.SA03008H.20180718.000020')=(65280,18432,0)\nX ModifyGraph rgb('B.SA03008H.20180718.000020')=(65280,36864,0)\nX ModifyGraph rgb('Vsource.SA03008H.20180718.000020')=(65280,55296,0)\nX ModifyGraph rgb('Lockin0.SA03008H.20180718.000020')=(57344,65280,0)\nX ModifyGraph rgb('Lockin1.SA03008H.20180718.000020')=(37376,65280,0)\nX ModifyGraph rgb('Lockin2.SA03008H.20180718.000020')=(18944,65280,0)\nX ModifyGraph rgb('Lockin3.SA03008H.20180718.000020')=(512,65280,0)\nX ModifyGraph rgb('Lockin4.SA03008H.20180718.000020')=(0,65280,17920)\nX ModifyGraph rgb('Lockin5.SA03008H.20180718.000020')=(0,65280,36352)\nX ModifyGraph rgb('B_rate.SA03008H.20180718.000020')=(0,65280,54784)\nX ModifyGraph rgb('DC0.SA03008H.20180718.000020')=(0,57856,65280)\nX ModifyGraph rgb('DC1.SA03008H.20180718.000020')=(0,39424,65280)\nX ModifyGraph rgb('DC2.SA03008H.20180718.000020')=(0,20992,65280)\nX ModifyGraph rgb('DC3.SA03008H.20180718.000020')=(0,2560,65280)\nX ModifyGraph rgb('DC4.SA03008H.20180718.000020')=(17408,0,65280)\nX ModifyGraph rgb('DC5.SA03008H.20180718.000020')=(35840,0,65280)\nX ModifyGraph rgb('DC6.SA03008H.20180718.000020')=(54272,0,65280)\nX ModifyGraph rgb('DC7.SA03008H.20180718.000020')=(65280,0,58368)\nX Legend/C/N=text0/J \"\\\\s('time.SA03008H.20180718.000020') time\\r\\\\s('temp.SA03008H.20180718.000020') temp\\r\\\\s('B.SA03008H.20180718.000020') B\\r\\\\s('Vsource.SA03008H.20180718.000020') Vsource\\r\\\\s('Lockin0.SA03008H.20180718.000020') Lockin0\\r\\\\s('Lockin1.SA03008H.20180718.000020') Lockin1\\r\\\\s('Lockin2.SA03008H.20180718.000020') Lockin2\\r\\\\s('Lockin3.SA03008H.20180718.000020') Lockin3\\r\\\\s('Lockin4.SA03008H.20180718.000020') Lockin4\\r\\\\s('Lockin5.SA03008H.20180718.000020') Lockin5\\r\\\\s('B_rate.SA03008H.20180718.000020') B_rate\\r\\\\s('DC0.SA03008H.20180718.000020') DC0\\r\\\\s('DC1.SA03008H.20180718.000020') DC1\\r\\\\s('DC2.SA03008H.20180718.000020') DC2\\r\\\\s('DC3.SA03008H.20180718.000020') DC3\\r\\\\s('DC4.SA03008H.20180718.000020') DC4\\r\\\\s('DC5.SA03008H.20180718.000020') DC5\\r\\\\s('DC6.SA03008H.20180718.000020') DC6\\r\\\\s('DC7.SA03008H.20180718.000020') DC7\"\nX ModifyGraph mirror(bottom)=1\nX ModifyGraph width=216\nX ModifyGraph height={Aspect,0.6}\nX ModifyGraph Log(bottom)=0\nX ModifyGraph Log(left)=0\nX \n", "IGOR\nX// Date: 7/18/2018 5:22 PM\nX// SA03008H\nX// \nX// Source 2 Drain 28 (lockin 1 and 7)\nX// Slow sweeping BG -5 to 5 inc. 0.1V \nX// Fast sweep SG -1 to 1 inc. 0.05V\n\nX// DSA_Vsg1=0.050000\n\nX// \nX// B= 0.000000\n\n\n\n\n\n\n\n\n\n\n\n\n\n\n\n\n\n\n\n\n\n\n\n\n\n\n\n\n\n\n\n\n\n\n\n\n\n\n\n\nX \nX Display/R 'time.SA03008H.20180718.000021'\nX AppendToGraph 'temp.SA03008H.20180718.000021'\nX AppendToGraph 'B.SA03008H.20180718.000021'\nX AppendToGraph 'Vsource.SA03008H.20180718.000021'\nX AppendToGraph 'Lockin0.SA03008H.20180718.000021'\nX AppendToGraph 'Lockin1.SA03008H.20180718.000021'\nX AppendToGraph 'Lockin2.SA03008H.20180718.000021'\nX AppendToGraph 'Lockin3.SA03008H.20180718.000021'\nX AppendToGraph 'Lockin4.SA03008H.20180718.000021'\nX AppendToGraph 'Lockin5.SA03008H.20180718.000021'\nX AppendToGraph 'B_rate.SA03008H.20180718.000021'\nX AppendToGraph 'DC0.SA03008H.20180718.000021'\nX AppendToGraph 'DC1.SA03008H.20180718.000021'\nX AppendToGraph 'DC2.SA03008H.20180718.000021'\nX AppendToGraph 'DC3.SA03008H.20180718.000021'\nX AppendToGraph 'DC4.SA03008H.20180718.000021'\nX AppendToGraph 'DC5.SA03008H.20180718.000021'\nX AppendToGraph 'DC6.SA03008H.20180718.000021'\nX AppendToGraph 'DC7.SA03008H.20180718.000021'\nX Label bottom \"x label\"\nX Label left \"y label\"\nX ModifyGraph rgb('time.SA03008H.20180718.000021')=(65280,0,0)\nX ModifyGraph rgb('temp.SA03008H.20180718.000021')=(65280,18432,0)\nX ModifyGraph rgb('B.SA03008H.20180718.000021')=(65280,36864,0)\nX ModifyGraph rgb('Vsource.SA03008H.20180718.000021')=(65280,55296,0)\nX ModifyGraph rgb('Lockin0.SA03008H.20180718.000021')=(57344,65280,0)\nX ModifyGraph rgb('Lockin1.SA03008H.20180718.000021')=(37376,65280,0)\nX ModifyGraph rgb('Lockin2.SA03008H.20180718.000021')=(18944,65280,0)\nX ModifyGraph rgb('Lockin3.SA03008H.20180718.000021')=(512,65280,0)\nX ModifyGraph rgb('Lockin4.SA03008H.20180718.000021')=(0,65280,17920)\nX ModifyGraph rgb('Lockin5.SA03008H.20180718.000021')=(0,65280,36352)\nX ModifyGraph rgb('B_rate.SA03008H.20180718.000021')=(0,65280,54784)\nX ModifyGraph rgb('DC0.SA03008H.20180718.000021')=(0,57856,65280)\nX ModifyGraph rgb('DC1.SA03008H.20180718.000021')=(0,39424,65280)\nX ModifyGraph rgb('DC2.SA03008H.20180718.000021')=(0,20992,65280)\nX ModifyGraph rgb('DC3.SA03008H.20180718.000021')=(0,2560,65280)\nX ModifyGraph rgb('DC4.SA03008H.20180718.000021')=(17408,0,65280)\nX ModifyGraph rgb('DC5.SA03008H.20180718.000021')=(35840,0,65280)\nX ModifyGraph rgb('DC6.SA03008H.20180718.000021')=(54272,0,65280)\nX ModifyGraph rgb('DC7.SA03008H.20180718.000021')=(65280,0,58368)\nX Legend/C/N=text0/J \"\\\\s('time.SA03008H.20180718.000021') time\\r\\\\s('temp.SA03008H.20180718.000021') temp\\r\\\\s('B.SA03008H.20180718.000021') B\\r\\\\s('Vsource.SA03008H.20180718.000021') Vsource\\r\\\\s('Lockin0.SA03008H.20180718.000021') Lockin0\\r\\\\s('Lockin1.SA03008H.20180718.000021') Lockin1\\r\\\\s('Lockin2.SA03008H.20180718.000021') Lockin2\\r\\\\s('Lockin3.SA03008H.20180718.000021') Lockin3\\r\\\\s('Lockin4.SA03008H.20180718.000021') Lockin4\\r\\\\s('Lockin5.SA03008H.20180718.000021') Lockin5\\r\\\\s('B_rate.SA03008H.20180718.000021') B_rate\\r\\\\s('DC0.SA03008H.20180718.000021') DC0\\r\\\\s('DC1.SA03008H.20180718.000021') DC1\\r\\\\s('DC2.SA03008H.20180718.000021') DC2\\r\\\\s('DC3.SA03008H.20180718.000021') DC3\\r\\\\s('DC4.SA03008H.20180718.000021') DC4\\r\\\\s('DC5.SA03008H.20180718.000021') DC5\\r\\\\s('DC6.SA03008H.20180718.000021') DC6\\r\\\\s('DC7.SA03008H.20180718.000021') DC7\"\nX ModifyGraph mirror(bottom)=1\nX ModifyGraph width=216\nX ModifyGraph height={Aspect,0.6}\nX ModifyGraph Log(bottom)=0\nX ModifyGraph Log(left)=0\nX \n", "IGOR\nX// Date: 7/18/2018 5:23 PM\nX// SA03008H\nX// \nX// Source 2 Drain 28 (lockin 1 and 7)\nX// Slow sweeping BG -5 to 5 inc. 0.1V \nX// Fast sweep SG -1 to 1 inc. 0.05V\n\nX// DSA_Vsg1=0.100000\n\nX// \nX// B= 0.000000\n\n\n\n\n\n\n\n\n\n\n\n\n\n\n\n\n\n\n\n\n\n\n\n\n\n\n\n\n\n\n\n\n\n\n\n\n\n\n\n\nX \nX Display/R 'time.SA03008H.20180718.000022'\nX AppendToGraph 'temp.SA03008H.20180718.000022'\nX AppendToGraph 'B.SA03008H.20180718.000022'\nX AppendToGraph 'Vsource.SA03008H.20180718.000022'\nX AppendToGraph 'Lockin0.SA03008H.20180718.000022'\nX AppendToGraph 'Lockin1.SA03008H.20180718.000022'\nX AppendToGraph 'Lockin2.SA03008H.20180718.000022'\nX AppendToGraph 'Lockin3.SA03008H.20180718.000022'\nX AppendToGraph 'Lockin4.SA03008H.20180718.000022'\nX AppendToGraph 'Lockin5.SA03008H.20180718.000022'\nX AppendToGraph 'B_rate.SA03008H.20180718.000022'\nX AppendToGraph 'DC0.SA03008H.20180718.000022'\nX AppendToGraph 'DC1.SA03008H.20180718.000022'\nX AppendToGraph 'DC2.SA03008H.20180718.000022'\nX AppendToGraph 'DC3.SA03008H.20180718.000022'\nX AppendToGraph 'DC4.SA03008H.20180718.000022'\nX AppendToGraph 'DC5.SA03008H.20180718.000022'\nX AppendToGraph 'DC6.SA03008H.20180718.000022'\nX AppendToGraph 'DC7.SA03008H.20180718.000022'\nX Label bottom \"x label\"\nX Label left \"y label\"\nX ModifyGraph rgb('time.SA03008H.20180718.000022')=(65280,0,0)\nX ModifyGraph rgb('temp.SA03008H.20180718.000022')=(65280,18432,0)\nX ModifyGraph rgb('B.SA03008H.20180718.000022')=(65280,36864,0)\nX ModifyGraph rgb('Vsource.SA03008H.20180718.000022')=(65280,55296,0)\nX ModifyGraph rgb('Lockin0.SA03008H.20180718.000022')=(57344,65280,0)\nX ModifyGraph rgb('Lockin1.SA03008H.20180718.000022')=(37376,65280,0)\nX ModifyGraph rgb('Lockin2.SA03008H.20180718.000022')=(18944,65280,0)\nX ModifyGraph rgb('Lockin3.SA03008H.20180718.000022')=(512,65280,0)\nX ModifyGraph rgb('Lockin4.SA03008H.20180718.000022')=(0,65280,17920)\nX ModifyGraph rgb('Lockin5.SA03008H.20180718.000022')=(0,65280,36352)\nX ModifyGraph rgb('B_rate.SA03008H.20180718.000022')=(0,65280,54784)\nX ModifyGraph rgb('DC0.SA03008H.20180718.000022')=(0,57856,65280)\nX ModifyGraph rgb('DC1.SA03008H.20180718.000022')=(0,39424,65280)\nX ModifyGraph rgb('DC2.SA03008H.20180718.000022')=(0,20992,65280)\nX ModifyGraph rgb('DC3.SA03008H.20180718.000022')=(0,2560,65280)\nX ModifyGraph rgb('DC4.SA03008H.20180718.000022')=(17408,0,65280)\nX ModifyGraph rgb('DC5.SA03008H.20180718.000022')=(35840,0,65280)\nX ModifyGraph rgb('DC6.SA03008H.20180718.000022')=(54272,0,65280)\nX ModifyGraph rgb('DC7.SA03008H.20180718.000022')=(65280,0,58368)\nX Legend/C/N=text0/J \"\\\\s('time.SA03008H.20180718.000022') time\\r\\\\s('temp.SA03008H.20180718.000022') temp\\r\\\\s('B.SA03008H.20180718.000022') B\\r\\\\s('Vsource.SA03008H.20180718.000022') Vsource\\r\\\\s('Lockin0.SA03008H.20180718.000022') Lockin0\\r\\\\s('Lockin1.SA03008H.20180718.000022') Lockin1\\r\\\\s('Lockin2.SA03008H.20180718.000022') Lockin2\\r\\\\s('Lockin3.SA03008H.20180718.000022') Lockin3\\r\\\\s('Lockin4.SA03008H.20180718.000022') Lockin4\\r\\\\s('Lockin5.SA03008H.20180718.000022') Lockin5\\r\\\\s('B_rate.SA03008H.20180718.000022') B_rate\\r\\\\s('DC0.SA03008H.20180718.000022') DC0\\r\\\\s('DC1.SA03008H.20180718.000022') DC1\\r\\\\s('DC2.SA03008H.20180718.000022') DC2\\r\\\\s('DC3.SA03008H.20180718.000022') DC3\\r\\\\s('DC4.SA03008H.20180718.000022') DC4\\r\\\\s('DC5.SA03008H.20180718.000022') DC5\\r\\\\s('DC6.SA03008H.20180718.000022') DC6\\r\\\\s('DC7.SA03008H.20180718.000022') DC7\"\nX ModifyGraph mirror(bottom)=1\nX ModifyGraph width=216\nX ModifyGraph height={Aspect,0.6}\nX ModifyGraph Log(bottom)=0\nX ModifyGraph Log(left)=0\nX \n", "IGOR\nX// Date: 7/18/2018 5:23 PM\nX// SA03008H\nX// \nX// Source 2 Drain 28 (lockin 1 and 7)\nX// Slow sweeping BG -5 to 5 inc. 0.1V \nX// Fast sweep SG -1 to 1 inc. 0.05V\n\nX// DSA_Vsg1=0.150000\n\nX// \nX// B= 0.000000\n\n\n\n\n\n\n\n\n\n\n\n\n\n\n\n\n\n\n\n\n\n\n\n\n\n\n\n\n\n\n\n\n\n\n\n\n\n\n\n\nX \nX Display/R 'time.SA03008H.20180718.000023'\nX AppendToGraph 'temp.SA03008H.20180718.000023'\nX AppendToGraph 'B.SA03008H.20180718.000023'\nX AppendToGraph 'Vsource.SA03008H.20180718.000023'\nX AppendToGraph 'Lockin0.SA03008H.20180718.000023'\nX AppendToGraph 'Lockin1.SA03008H.20180718.000023'\nX AppendToGraph 'Lockin2.SA03008H.20180718.000023'\nX AppendToGraph 'Lockin3.SA03008H.20180718.000023'\nX AppendToGraph 'Lockin4.SA03008H.20180718.000023'\nX AppendToGraph 'Lockin5.SA03008H.20180718.000023'\nX AppendToGraph 'B_rate.SA03008H.20180718.000023'\nX AppendToGraph 'DC0.SA03008H.20180718.000023'\nX AppendToGraph 'DC1.SA03008H.20180718.000023'\nX AppendToGraph 'DC2.SA03008H.20180718.000023'\nX AppendToGraph 'DC3.SA03008H.20180718.000023'\nX AppendToGraph 'DC4.SA03008H.20180718.000023'\nX AppendToGraph 'DC5.SA03008H.20180718.000023'\nX AppendToGraph 'DC6.SA03008H.20180718.000023'\nX AppendToGraph 'DC7.SA03008H.20180718.000023'\nX Label bottom \"x label\"\nX Label left \"y label\"\nX ModifyGraph rgb('time.SA03008H.20180718.000023')=(65280,0,0)\nX ModifyGraph rgb('temp.SA03008H.20180718.000023')=(65280,18432,0)\nX ModifyGraph rgb('B.SA03008H.20180718.000023')=(65280,36864,0)\nX ModifyGraph rgb('Vsource.SA03008H.20180718.000023')=(65280,55296,0)\nX ModifyGraph rgb('Lockin0.SA03008H.20180718.000023')=(57344,65280,0)\nX ModifyGraph rgb('Lockin1.SA03008H.20180718.000023')=(37376,65280,0)\nX ModifyGraph rgb('Lockin2.SA03008H.20180718.000023')=(18944,65280,0)\nX ModifyGraph rgb('Lockin3.SA03008H.20180718.000023')=(512,65280,0)\nX ModifyGraph rgb('Lockin4.SA03008H.20180718.000023')=(0,65280,17920)\nX ModifyGraph rgb('Lockin5.SA03008H.20180718.000023')=(0,65280,36352)\nX ModifyGraph rgb('B_rate.SA03008H.20180718.000023')=(0,65280,54784)\nX ModifyGraph rgb('DC0.SA03008H.20180718.000023')=(0,57856,65280)\nX ModifyGraph rgb('DC1.SA03008H.20180718.000023')=(0,39424,65280)\nX ModifyGraph rgb('DC2.SA03008H.20180718.000023')=(0,20992,65280)\nX ModifyGraph rgb('DC3.SA03008H.20180718.000023')=(0,2560,65280)\nX ModifyGraph rgb('DC4.SA03008H.20180718.000023')=(17408,0,65280)\nX ModifyGraph rgb('DC5.SA03008H.20180718.000023')=(35840,0,65280)\nX ModifyGraph rgb('DC6.SA03008H.20180718.000023')=(54272,0,65280)\nX ModifyGraph rgb('DC7.SA03008H.20180718.000023')=(65280,0,58368)\nX Legend/C/N=text0/J \"\\\\s('time.SA03008H.20180718.000023') time\\r\\\\s('temp.SA03008H.20180718.000023') temp\\r\\\\s('B.SA03008H.20180718.000023') B\\r\\\\s('Vsource.SA03008H.20180718.000023') Vsource\\r\\\\s('Lockin0.SA03008H.20180718.000023') Lockin0\\r\\\\s('Lockin1.SA03008H.20180718.000023') Lockin1\\r\\\\s('Lockin2.SA03008H.20180718.000023') Lockin2\\r\\\\s('Lockin3.SA03008H.20180718.000023') Lockin3\\r\\\\s('Lockin4.SA03008H.20180718.000023') Lockin4\\r\\\\s('Lockin5.SA03008H.20180718.000023') Lockin5\\r\\\\s('B_rate.SA03008H.20180718.000023') B_rate\\r\\\\s('DC0.SA03008H.20180718.000023') DC0\\r\\\\s('DC1.SA03008H.20180718.000023') DC1\\r\\\\s('DC2.SA03008H.20180718.000023') DC2\\r\\\\s('DC3.SA03008H.20180718.000023') DC3\\r\\\\s('DC4.SA03008H.20180718.000023') DC4\\r\\\\s('DC5.SA03008H.20180718.000023') DC5\\r\\\\s('DC6.SA03008H.20180718.000023') DC6\\r\\\\s('DC7.SA03008H.20180718.000023') DC7\"\nX ModifyGraph mirror(bottom)=1\nX ModifyGraph width=216\nX ModifyGraph height={Aspect,0.6}\nX ModifyGraph Log(bottom)=0\nX ModifyGraph Log(left)=0\nX \n", "IGOR\nX// Date: 7/18/2018 5:23 PM\nX// SA03008H\nX// \nX// Source 2 Drain 28 (lockin 1 and 7)\nX// Slow sweeping BG -5 to 5 inc. 0.1V \nX// Fast sweep SG -1 to 1 inc. 0.05V\n\nX// DSA_Vsg1=0.200000\n\nX// \nX// B= 0.000000\n\n\n\n\n\n\n\n\n\n\n\n\n\n\n\n\n\n\n\n\n\n\n\n\n\n\n\n\n\n\n\n\n\n\n\n\n\n\n\n\nX \nX Display/R 'time.SA03008H.20180718.000024'\nX AppendToGraph 'temp.SA03008H.20180718.000024'\nX AppendToGraph 'B.SA03008H.20180718.000024'\nX AppendToGraph 'Vsource.SA03008H.20180718.000024'\nX AppendToGraph 'Lockin0.SA03008H.20180718.000024'\nX AppendToGraph 'Lockin1.SA03008H.20180718.000024'\nX AppendToGraph 'Lockin2.SA03008H.20180718.000024'\nX AppendToGraph 'Lockin3.SA03008H.20180718.000024'\nX AppendToGraph 'Lockin4.SA03008H.20180718.000024'\nX AppendToGraph 'Lockin5.SA03008H.20180718.000024'\nX AppendToGraph 'B_rate.SA03008H.20180718.000024'\nX AppendToGraph 'DC0.SA03008H.20180718.000024'\nX AppendToGraph 'DC1.SA03008H.20180718.000024'\nX AppendToGraph 'DC2.SA03008H.20180718.000024'\nX AppendToGraph 'DC3.SA03008H.20180718.000024'\nX AppendToGraph 'DC4.SA03008H.20180718.000024'\nX AppendToGraph 'DC5.SA03008H.20180718.000024'\nX AppendToGraph 'DC6.SA03008H.20180718.000024'\nX AppendToGraph 'DC7.SA03008H.20180718.000024'\nX Label bottom \"x label\"\nX Label left \"y label\"\nX ModifyGraph rgb('time.SA03008H.20180718.000024')=(65280,0,0)\nX ModifyGraph rgb('temp.SA03008H.20180718.000024')=(65280,18432,0)\nX ModifyGraph rgb('B.SA03008H.20180718.000024')=(65280,36864,0)\nX ModifyGraph rgb('Vsource.SA03008H.20180718.000024')=(65280,55296,0)\nX ModifyGraph rgb('Lockin0.SA03008H.20180718.000024')=(57344,65280,0)\nX ModifyGraph rgb('Lockin1.SA03008H.20180718.000024')=(37376,65280,0)\nX ModifyGraph rgb('Lockin2.SA03008H.20180718.000024')=(18944,65280,0)\nX ModifyGraph rgb('Lockin3.SA03008H.20180718.000024')=(512,65280,0)\nX ModifyGraph rgb('Lockin4.SA03008H.20180718.000024')=(0,65280,17920)\nX ModifyGraph rgb('Lockin5.SA03008H.20180718.000024')=(0,65280,36352)\nX ModifyGraph rgb('B_rate.SA03008H.20180718.000024')=(0,65280,54784)\nX ModifyGraph rgb('DC0.SA03008H.20180718.000024')=(0,57856,65280)\nX ModifyGraph rgb('DC1.SA03008H.20180718.000024')=(0,39424,65280)\nX ModifyGraph rgb('DC2.SA03008H.20180718.000024')=(0,20992,65280)\nX ModifyGraph rgb('DC3.SA03008H.20180718.000024')=(0,2560,65280)\nX ModifyGraph rgb('DC4.SA03008H.20180718.000024')=(17408,0,65280)\nX ModifyGraph rgb('DC5.SA03008H.20180718.000024')=(35840,0,65280)\nX ModifyGraph rgb('DC6.SA03008H.20180718.000024')=(54272,0,65280)\nX ModifyGraph rgb('DC7.SA03008H.20180718.000024')=(65280,0,58368)\nX Legend/C/N=text0/J \"\\\\s('time.SA03008H.20180718.000024') time\\r\\\\s('temp.SA03008H.20180718.000024') temp\\r\\\\s('B.SA03008H.20180718.000024') B\\r\\\\s('Vsource.SA03008H.20180718.000024') Vsource\\r\\\\s('Lockin0.SA03008H.20180718.000024') Lockin0\\r\\\\s('Lockin1.SA03008H.20180718.000024') Lockin1\\r\\\\s('Lockin2.SA03008H.20180718.000024') Lockin2\\r\\\\s('Lockin3.SA03008H.20180718.000024') Lockin3\\r\\\\s('Lockin4.SA03008H.20180718.000024') Lockin4\\r\\\\s('Lockin5.SA03008H.20180718.000024') Lockin5\\r\\\\s('B_rate.SA03008H.20180718.000024') B_rate\\r\\\\s('DC0.SA03008H.20180718.000024') DC0\\r\\\\s('DC1.SA03008H.20180718.000024') DC1\\r\\\\s('DC2.SA03008H.20180718.000024') DC2\\r\\\\s('DC3.SA03008H.20180718.000024') DC3\\r\\\\s('DC4.SA03008H.20180718.000024') DC4\\r\\\\s('DC5.SA03008H.20180718.000024') DC5\\r\\\\s('DC6.SA03008H.20180718.000024') DC6\\r\\\\s('DC7.SA03008H.20180718.000024') DC7\"\nX ModifyGraph mirror(bottom)=1\nX ModifyGraph width=216\nX ModifyGraph height={Aspect,0.6}\nX ModifyGraph Log(bottom)=0\nX ModifyGraph Log(left)=0\nX \n", "IGOR\nX// Date: 7/18/2018 5:23 PM\nX// SA03008H\nX// \nX// Source 2 Drain 28 (lockin 1 and 7)\nX// Slow sweeping BG -5 to 5 inc. 0.1V \nX// Fast sweep SG -1 to 1 inc. 0.05V\n\nX// DSA_Vsg1=0.250000\n\nX// \nX// B= 0.000000\n\n\n\n\n\n\n\n\n\n\n\n\n\n\n\n\n\n\n\n\n\n\n\n\n\n\n\n\n\n\n\n\n\n\n\n\n\n\n\n\nX \nX Display/R 'time.SA03008H.20180718.000025'\nX AppendToGraph 'temp.SA03008H.20180718.000025'\nX AppendToGraph 'B.SA03008H.20180718.000025'\nX AppendToGraph 'Vsource.SA03008H.20180718.000025'\nX AppendToGraph 'Lockin0.SA03008H.20180718.000025'\nX AppendToGraph 'Lockin1.SA03008H.20180718.000025'\nX AppendToGraph 'Lockin2.SA03008H.20180718.000025'\nX AppendToGraph 'Lockin3.SA03008H.20180718.000025'\nX AppendToGraph 'Lockin4.SA03008H.20180718.000025'\nX AppendToGraph 'Lockin5.SA03008H.20180718.000025'\nX AppendToGraph 'B_rate.SA03008H.20180718.000025'\nX AppendToGraph 'DC0.SA03008H.20180718.000025'\nX AppendToGraph 'DC1.SA03008H.20180718.000025'\nX AppendToGraph 'DC2.SA03008H.20180718.000025'\nX AppendToGraph 'DC3.SA03008H.20180718.000025'\nX AppendToGraph 'DC4.SA03008H.20180718.000025'\nX AppendToGraph 'DC5.SA03008H.20180718.000025'\nX AppendToGraph 'DC6.SA03008H.20180718.000025'\nX AppendToGraph 'DC7.SA03008H.20180718.000025'\nX Label bottom \"x label\"\nX Label left \"y label\"\nX ModifyGraph rgb('time.SA03008H.20180718.000025')=(65280,0,0)\nX ModifyGraph rgb('temp.SA03008H.20180718.000025')=(65280,18432,0)\nX ModifyGraph rgb('B.SA03008H.20180718.000025')=(65280,36864,0)\nX ModifyGraph rgb('Vsource.SA03008H.20180718.000025')=(65280,55296,0)\nX ModifyGraph rgb('Lockin0.SA03008H.20180718.000025')=(57344,65280,0)\nX ModifyGraph rgb('Lockin1.SA03008H.20180718.000025')=(37376,65280,0)\nX ModifyGraph rgb('Lockin2.SA03008H.20180718.000025')=(18944,65280,0)\nX ModifyGraph rgb('Lockin3.SA03008H.20180718.000025')=(512,65280,0)\nX ModifyGraph rgb('Lockin4.SA03008H.20180718.000025')=(0,65280,17920)\nX ModifyGraph rgb('Lockin5.SA03008H.20180718.000025')=(0,65280,36352)\nX ModifyGraph rgb('B_rate.SA03008H.20180718.000025')=(0,65280,54784)\nX ModifyGraph rgb('DC0.SA03008H.20180718.000025')=(0,57856,65280)\nX ModifyGraph rgb('DC1.SA03008H.20180718.000025')=(0,39424,65280)\nX ModifyGraph rgb('DC2.SA03008H.20180718.000025')=(0,20992,65280)\nX ModifyGraph rgb('DC3.SA03008H.20180718.000025')=(0,2560,65280)\nX ModifyGraph rgb('DC4.SA03008H.20180718.000025')=(17408,0,65280)\nX ModifyGraph rgb('DC5.SA03008H.20180718.000025')=(35840,0,65280)\nX ModifyGraph rgb('DC6.SA03008H.20180718.000025')=(54272,0,65280)\nX ModifyGraph rgb('DC7.SA03008H.20180718.000025')=(65280,0,58368)\nX Legend/C/N=text0/J \"\\\\s('time.SA03008H.20180718.000025') time\\r\\\\s('temp.SA03008H.20180718.000025') temp\\r\\\\s('B.SA03008H.20180718.000025') B\\r\\\\s('Vsource.SA03008H.20180718.000025') Vsource\\r\\\\s('Lockin0.SA03008H.20180718.000025') Lockin0\\r\\\\s('Lockin1.SA03008H.20180718.000025') Lockin1\\r\\\\s('Lockin2.SA03008H.20180718.000025') Lockin2\\r\\\\s('Lockin3.SA03008H.20180718.000025') Lockin3\\r\\\\s('Lockin4.SA03008H.20180718.000025') Lockin4\\r\\\\s('Lockin5.SA03008H.20180718.000025') Lockin5\\r\\\\s('B_rate.SA03008H.20180718.000025') B_rate\\r\\\\s('DC0.SA03008H.20180718.000025') DC0\\r\\\\s('DC1.SA03008H.20180718.000025') DC1\\r\\\\s('DC2.SA03008H.20180718.000025') DC2\\r\\\\s('DC3.SA03008H.20180718.000025') DC3\\r\\\\s('DC4.SA03008H.20180718.000025') DC4\\r\\\\s('DC5.SA03008H.20180718.000025') DC5\\r\\\\s('DC6.SA03008H.20180718.000025') DC6\\r\\\\s('DC7.SA03008H.20180718.000025') DC7\"\nX ModifyGraph mirror(bottom)=1\nX ModifyGraph width=216\nX ModifyGraph height={Aspect,0.6}\nX ModifyGraph Log(bottom)=0\nX ModifyGraph Log(left)=0\nX \n", "IGOR\nX// Date: 7/18/2018 5:23 PM\nX// SA03008H\nX// \nX// Source 2 Drain 28 (lockin 1 and 7)\nX// Slow sweeping BG -5 to 5 inc. 0.1V \nX// Fast sweep SG -1 to 1 inc. 0.05V\n\nX// DSA_Vsg1=0.300000\n\nX// \nX// B= 0.000000\n\n\n\n\n\n\n\n\n\n\n\n\n\n\n\n\n\n\n\n\n\n\n\n\n\n\n\n\n\n\n\n\n\n\n\n\n\n\n\n\nX \nX Display/R 'time.SA03008H.20180718.000026'\nX AppendToGraph 'temp.SA03008H.20180718.000026'\nX AppendToGraph 'B.SA03008H.20180718.000026'\nX AppendToGraph 'Vsource.SA03008H.20180718.000026'\nX AppendToGraph 'Lockin0.SA03008H.20180718.000026'\nX AppendToGraph 'Lockin1.SA03008H.20180718.000026'\nX AppendToGraph 'Lockin2.SA03008H.20180718.000026'\nX AppendToGraph 'Lockin3.SA03008H.20180718.000026'\nX AppendToGraph 'Lockin4.SA03008H.20180718.000026'\nX AppendToGraph 'Lockin5.SA03008H.20180718.000026'\nX AppendToGraph 'B_rate.SA03008H.20180718.000026'\nX AppendToGraph 'DC0.SA03008H.20180718.000026'\nX AppendToGraph 'DC1.SA03008H.20180718.000026'\nX AppendToGraph 'DC2.SA03008H.20180718.000026'\nX AppendToGraph 'DC3.SA03008H.20180718.000026'\nX AppendToGraph 'DC4.SA03008H.20180718.000026'\nX AppendToGraph 'DC5.SA03008H.20180718.000026'\nX AppendToGraph 'DC6.SA03008H.20180718.000026'\nX AppendToGraph 'DC7.SA03008H.20180718.000026'\nX Label bottom \"x label\"\nX Label left \"y label\"\nX ModifyGraph rgb('time.SA03008H.20180718.000026')=(65280,0,0)\nX ModifyGraph rgb('temp.SA03008H.20180718.000026')=(65280,18432,0)\nX ModifyGraph rgb('B.SA03008H.20180718.000026')=(65280,36864,0)\nX ModifyGraph rgb('Vsource.SA03008H.20180718.000026')=(65280,55296,0)\nX ModifyGraph rgb('Lockin0.SA03008H.20180718.000026')=(57344,65280,0)\nX ModifyGraph rgb('Lockin1.SA03008H.20180718.000026')=(37376,65280,0)\nX ModifyGraph rgb('Lockin2.SA03008H.20180718.000026')=(18944,65280,0)\nX ModifyGraph rgb('Lockin3.SA03008H.20180718.000026')=(512,65280,0)\nX ModifyGraph rgb('Lockin4.SA03008H.20180718.000026')=(0,65280,17920)\nX ModifyGraph rgb('Lockin5.SA03008H.20180718.000026')=(0,65280,36352)\nX ModifyGraph rgb('B_rate.SA03008H.20180718.000026')=(0,65280,54784)\nX ModifyGraph rgb('DC0.SA03008H.20180718.000026')=(0,57856,65280)\nX ModifyGraph rgb('DC1.SA03008H.20180718.000026')=(0,39424,65280)\nX ModifyGraph rgb('DC2.SA03008H.20180718.000026')=(0,20992,65280)\nX ModifyGraph rgb('DC3.SA03008H.20180718.000026')=(0,2560,65280)\nX ModifyGraph rgb('DC4.SA03008H.20180718.000026')=(17408,0,65280)\nX ModifyGraph rgb('DC5.SA03008H.20180718.000026')=(35840,0,65280)\nX ModifyGraph rgb('DC6.SA03008H.20180718.000026')=(54272,0,65280)\nX ModifyGraph rgb('DC7.SA03008H.20180718.000026')=(65280,0,58368)\nX Legend/C/N=text0/J \"\\\\s('time.SA03008H.20180718.000026') time\\r\\\\s('temp.SA03008H.20180718.000026') temp\\r\\\\s('B.SA03008H.20180718.000026') B\\r\\\\s('Vsource.SA03008H.20180718.000026') Vsource\\r\\\\s('Lockin0.SA03008H.20180718.000026') Lockin0\\r\\\\s('Lockin1.SA03008H.20180718.000026') Lockin1\\r\\\\s('Lockin2.SA03008H.20180718.000026') Lockin2\\r\\\\s('Lockin3.SA03008H.20180718.000026') Lockin3\\r\\\\s('Lockin4.SA03008H.20180718.000026') Lockin4\\r\\\\s('Lockin5.SA03008H.20180718.000026') Lockin5\\r\\\\s('B_rate.SA03008H.20180718.000026') B_rate\\r\\\\s('DC0.SA03008H.20180718.000026') DC0\\r\\\\s('DC1.SA03008H.20180718.000026') DC1\\r\\\\s('DC2.SA03008H.20180718.000026') DC2\\r\\\\s('DC3.SA03008H.20180718.000026') DC3\\r\\\\s('DC4.SA03008H.20180718.000026') DC4\\r\\\\s('DC5.SA03008H.20180718.000026') DC5\\r\\\\s('DC6.SA03008H.20180718.000026') DC6\\r\\\\s('DC7.SA03008H.20180718.000026') DC7\"\nX ModifyGraph mirror(bottom)=1\nX ModifyGraph width=216\nX ModifyGraph height={Aspect,0.6}\nX ModifyGraph Log(bottom)=0\nX ModifyGraph Log(left)=0\nX \n", "IGOR\nX// Date: 7/18/2018 5:24 PM\nX// SA03008H\nX// \nX// Source 2 Drain 28 (lockin 1 and 7)\nX// Slow sweeping BG -5 to 5 inc. 0.1V \nX// Fast sweep SG -1 to 1 inc. 0.05V\n\nX// DSA_Vsg1=0.350000\n\nX// \nX// B= 0.000000\n\n\n\n\n\n\n\n\n\n\n\n\n\n\n\n\n\n\n\n\n\n\n\n\n\n\n\n\n\n\n\n\n\n\n\n\n\n\n\n\nX \nX Display/R 'time.SA03008H.20180718.000027'\nX AppendToGraph 'temp.SA03008H.20180718.000027'\nX AppendToGraph 'B.SA03008H.20180718.000027'\nX AppendToGraph 'Vsource.SA03008H.20180718.000027'\nX AppendToGraph 'Lockin0.SA03008H.20180718.000027'\nX AppendToGraph 'Lockin1.SA03008H.20180718.000027'\nX AppendToGraph 'Lockin2.SA03008H.20180718.000027'\nX AppendToGraph 'Lockin3.SA03008H.20180718.000027'\nX AppendToGraph 'Lockin4.SA03008H.20180718.000027'\nX AppendToGraph 'Lockin5.SA03008H.20180718.000027'\nX AppendToGraph 'B_rate.SA03008H.20180718.000027'\nX AppendToGraph 'DC0.SA03008H.20180718.000027'\nX AppendToGraph 'DC1.SA03008H.20180718.000027'\nX AppendToGraph 'DC2.SA03008H.20180718.000027'\nX AppendToGraph 'DC3.SA03008H.20180718.000027'\nX AppendToGraph 'DC4.SA03008H.20180718.000027'\nX AppendToGraph 'DC5.SA03008H.20180718.000027'\nX AppendToGraph 'DC6.SA03008H.20180718.000027'\nX AppendToGraph 'DC7.SA03008H.20180718.000027'\nX Label bottom \"x label\"\nX Label left \"y label\"\nX ModifyGraph rgb('time.SA03008H.20180718.000027')=(65280,0,0)\nX ModifyGraph rgb('temp.SA03008H.20180718.000027')=(65280,18432,0)\nX ModifyGraph rgb('B.SA03008H.20180718.000027')=(65280,36864,0)\nX ModifyGraph rgb('Vsource.SA03008H.20180718.000027')=(65280,55296,0)\nX ModifyGraph rgb('Lockin0.SA03008H.20180718.000027')=(57344,65280,0)\nX ModifyGraph rgb('Lockin1.SA03008H.20180718.000027')=(37376,65280,0)\nX ModifyGraph rgb('Lockin2.SA03008H.20180718.000027')=(18944,65280,0)\nX ModifyGraph rgb('Lockin3.SA03008H.20180718.000027')=(512,65280,0)\nX ModifyGraph rgb('Lockin4.SA03008H.20180718.000027')=(0,65280,17920)\nX ModifyGraph rgb('Lockin5.SA03008H.20180718.000027')=(0,65280,36352)\nX ModifyGraph rgb('B_rate.SA03008H.20180718.000027')=(0,65280,54784)\nX ModifyGraph rgb('DC0.SA03008H.20180718.000027')=(0,57856,65280)\nX ModifyGraph rgb('DC1.SA03008H.20180718.000027')=(0,39424,65280)\nX ModifyGraph rgb('DC2.SA03008H.20180718.000027')=(0,20992,65280)\nX ModifyGraph rgb('DC3.SA03008H.20180718.000027')=(0,2560,65280)\nX ModifyGraph rgb('DC4.SA03008H.20180718.000027')=(17408,0,65280)\nX ModifyGraph rgb('DC5.SA03008H.20180718.000027')=(35840,0,65280)\nX ModifyGraph rgb('DC6.SA03008H.20180718.000027')=(54272,0,65280)\nX ModifyGraph rgb('DC7.SA03008H.20180718.000027')=(65280,0,58368)\nX Legend/C/N=text0/J \"\\\\s('time.SA03008H.20180718.000027') time\\r\\\\s('temp.SA03008H.20180718.000027') temp\\r\\\\s('B.SA03008H.20180718.000027') B\\r\\\\s('Vsource.SA03008H.20180718.000027') Vsource\\r\\\\s('Lockin0.SA03008H.20180718.000027') Lockin0\\r\\\\s('Lockin1.SA03008H.20180718.000027') Lockin1\\r\\\\s('Lockin2.SA03008H.20180718.000027') Lockin2\\r\\\\s('Lockin3.SA03008H.20180718.000027') Lockin3\\r\\\\s('Lockin4.SA03008H.20180718.000027') Lockin4\\r\\\\s('Lockin5.SA03008H.20180718.000027') Lockin5\\r\\\\s('B_rate.SA03008H.20180718.000027') B_rate\\r\\\\s('DC0.SA03008H.20180718.000027') DC0\\r\\\\s('DC1.SA03008H.20180718.000027') DC1\\r\\\\s('DC2.SA03008H.20180718.000027') DC2\\r\\\\s('DC3.SA03008H.20180718.000027') DC3\\r\\\\s('DC4.SA03008H.20180718.000027') DC4\\r\\\\s('DC5.SA03008H.20180718.000027') DC5\\r\\\\s('DC6.SA03008H.20180718.000027') DC6\\r\\\\s('DC7.SA03008H.20180718.000027') DC7\"\nX ModifyGraph mirror(bottom)=1\nX ModifyGraph width=216\nX ModifyGraph height={Aspect,0.6}\nX ModifyGraph Log(bottom)=0\nX ModifyGraph Log(left)=0\nX \n", "IGOR\nX// Date: 7/18/2018 5:24 PM\nX// SA03008H\nX// \nX// Source 2 Drain 28 (lockin 1 and 7)\nX// Slow sweeping BG -5 to 5 inc. 0.1V \nX// Fast sweep SG -1 to 1 inc. 0.05V\n\nX// DSA_Vsg1=0.400000\n\nX// \nX// B= 0.000000\n\n\n\n\n\n\n\n\n\n\n\n\n\n\n\n\n\n\n\n\n\n\n\n\n\n\n\n\n\n\n\n\n\n\n\n\n\n\n\n\nX \nX Display/R 'time.SA03008H.20180718.000028'\nX AppendToGraph 'temp.SA03008H.20180718.000028'\nX AppendToGraph 'B.SA03008H.20180718.000028'\nX AppendToGraph 'Vsource.SA03008H.20180718.000028'\nX AppendToGraph 'Lockin0.SA03008H.20180718.000028'\nX AppendToGraph 'Lockin1.SA03008H.20180718.000028'\nX AppendToGraph 'Lockin2.SA03008H.20180718.000028'\nX AppendToGraph 'Lockin3.SA03008H.20180718.000028'\nX AppendToGraph 'Lockin4.SA03008H.20180718.000028'\nX AppendToGraph 'Lockin5.SA03008H.20180718.000028'\nX AppendToGraph 'B_rate.SA03008H.20180718.000028'\nX AppendToGraph 'DC0.SA03008H.20180718.000028'\nX AppendToGraph 'DC1.SA03008H.20180718.000028'\nX AppendToGraph 'DC2.SA03008H.20180718.000028'\nX AppendToGraph 'DC3.SA03008H.20180718.000028'\nX AppendToGraph 'DC4.SA03008H.20180718.000028'\nX AppendToGraph 'DC5.SA03008H.20180718.000028'\nX AppendToGraph 'DC6.SA03008H.20180718.000028'\nX AppendToGraph 'DC7.SA03008H.20180718.000028'\nX Label bottom \"x label\"\nX Label left \"y label\"\nX ModifyGraph rgb('time.SA03008H.20180718.000028')=(65280,0,0)\nX ModifyGraph rgb('temp.SA03008H.20180718.000028')=(65280,18432,0)\nX ModifyGraph rgb('B.SA03008H.20180718.000028')=(65280,36864,0)\nX ModifyGraph rgb('Vsource.SA03008H.20180718.000028')=(65280,55296,0)\nX ModifyGraph rgb('Lockin0.SA03008H.20180718.000028')=(57344,65280,0)\nX ModifyGraph rgb('Lockin1.SA03008H.20180718.000028')=(37376,65280,0)\nX ModifyGraph rgb('Lockin2.SA03008H.20180718.000028')=(18944,65280,0)\nX ModifyGraph rgb('Lockin3.SA03008H.20180718.000028')=(512,65280,0)\nX ModifyGraph rgb('Lockin4.SA03008H.20180718.000028')=(0,65280,17920)\nX ModifyGraph rgb('Lockin5.SA03008H.20180718.000028')=(0,65280,36352)\nX ModifyGraph rgb('B_rate.SA03008H.20180718.000028')=(0,65280,54784)\nX ModifyGraph rgb('DC0.SA03008H.20180718.000028')=(0,57856,65280)\nX ModifyGraph rgb('DC1.SA03008H.20180718.000028')=(0,39424,65280)\nX ModifyGraph rgb('DC2.SA03008H.20180718.000028')=(0,20992,65280)\nX ModifyGraph rgb('DC3.SA03008H.20180718.000028')=(0,2560,65280)\nX ModifyGraph rgb('DC4.SA03008H.20180718.000028')=(17408,0,65280)\nX ModifyGraph rgb('DC5.SA03008H.20180718.000028')=(35840,0,65280)\nX ModifyGraph rgb('DC6.SA03008H.20180718.000028')=(54272,0,65280)\nX ModifyGraph rgb('DC7.SA03008H.20180718.000028')=(65280,0,58368)\nX Legend/C/N=text0/J \"\\\\s('time.SA03008H.20180718.000028') time\\r\\\\s('temp.SA03008H.20180718.000028') temp\\r\\\\s('B.SA03008H.20180718.000028') B\\r\\\\s('Vsource.SA03008H.20180718.000028') Vsource\\r\\\\s('Lockin0.SA03008H.20180718.000028') Lockin0\\r\\\\s('Lockin1.SA03008H.20180718.000028') Lockin1\\r\\\\s('Lockin2.SA03008H.20180718.000028') Lockin2\\r\\\\s('Lockin3.SA03008H.20180718.000028') Lockin3\\r\\\\s('Lockin4.SA03008H.20180718.000028') Lockin4\\r\\\\s('Lockin5.SA03008H.20180718.000028') Lockin5\\r\\\\s('B_rate.SA03008H.20180718.000028') B_rate\\r\\\\s('DC0.SA03008H.20180718.000028') DC0\\r\\\\s('DC1.SA03008H.20180718.000028') DC1\\r\\\\s('DC2.SA03008H.20180718.000028') DC2\\r\\\\s('DC3.SA03008H.20180718.000028') DC3\\r\\\\s('DC4.SA03008H.20180718.000028') DC4\\r\\\\s('DC5.SA03008H.20180718.000028') DC5\\r\\\\s('DC6.SA03008H.20180718.000028') DC6\\r\\\\s('DC7.SA03008H.20180718.000028') DC7\"\nX ModifyGraph mirror(bottom)=1\nX ModifyGraph width=216\nX ModifyGraph height={Aspect,0.6}\nX ModifyGraph Log(bottom)=0\nX ModifyGraph Log(left)=0\nX \n", "IGOR\nX// Date: 7/18/2018 5:24 PM\nX// SA03008H\nX// \nX// Source 2 Drain 28 (lockin 1 and 7)\nX// Slow sweeping BG -5 to 5 inc. 0.1V \nX// Fast sweep SG -1 to 1 inc. 0.05V\n\nX// DSA_Vsg1=0.450000\n\nX// \nX// B= 0.000000\n\n\n\n\n\n\n\n\n\n\n\n\n\n\n\n\n\n\n\n\n\n\n\n\n\n\n\n\n\n\n\n\n\n\n\n\n\n\n\n\nX \nX Display/R 'time.SA03008H.20180718.000029'\nX AppendToGraph 'temp.SA03008H.20180718.000029'\nX AppendToGraph 'B.SA03008H.20180718.000029'\nX AppendToGraph 'Vsource.SA03008H.20180718.000029'\nX AppendToGraph 'Lockin0.SA03008H.20180718.000029'\nX AppendToGraph 'Lockin1.SA03008H.20180718.000029'\nX AppendToGraph 'Lockin2.SA03008H.20180718.000029'\nX AppendToGraph 'Lockin3.SA03008H.20180718.000029'\nX AppendToGraph 'Lockin4.SA03008H.20180718.000029'\nX AppendToGraph 'Lockin5.SA03008H.20180718.000029'\nX AppendToGraph 'B_rate.SA03008H.20180718.000029'\nX AppendToGraph 'DC0.SA03008H.20180718.000029'\nX AppendToGraph 'DC1.SA03008H.20180718.000029'\nX AppendToGraph 'DC2.SA03008H.20180718.000029'\nX AppendToGraph 'DC3.SA03008H.20180718.000029'\nX AppendToGraph 'DC4.SA03008H.20180718.000029'\nX AppendToGraph 'DC5.SA03008H.20180718.000029'\nX AppendToGraph 'DC6.SA03008H.20180718.000029'\nX AppendToGraph 'DC7.SA03008H.20180718.000029'\nX Label bottom \"x label\"\nX Label left \"y label\"\nX ModifyGraph rgb('time.SA03008H.20180718.000029')=(65280,0,0)\nX ModifyGraph rgb('temp.SA03008H.20180718.000029')=(65280,18432,0)\nX ModifyGraph rgb('B.SA03008H.20180718.000029')=(65280,36864,0)\nX ModifyGraph rgb('Vsource.SA03008H.20180718.000029')=(65280,55296,0)\nX ModifyGraph rgb('Lockin0.SA03008H.20180718.000029')=(57344,65280,0)\nX ModifyGraph rgb('Lockin1.SA03008H.20180718.000029')=(37376,65280,0)\nX ModifyGraph rgb('Lockin2.SA03008H.20180718.000029')=(18944,65280,0)\nX ModifyGraph rgb('Lockin3.SA03008H.20180718.000029')=(512,65280,0)\nX ModifyGraph rgb('Lockin4.SA03008H.20180718.000029')=(0,65280,17920)\nX ModifyGraph rgb('Lockin5.SA03008H.20180718.000029')=(0,65280,36352)\nX ModifyGraph rgb('B_rate.SA03008H.20180718.000029')=(0,65280,54784)\nX ModifyGraph rgb('DC0.SA03008H.20180718.000029')=(0,57856,65280)\nX ModifyGraph rgb('DC1.SA03008H.20180718.000029')=(0,39424,65280)\nX ModifyGraph rgb('DC2.SA03008H.20180718.000029')=(0,20992,65280)\nX ModifyGraph rgb('DC3.SA03008H.20180718.000029')=(0,2560,65280)\nX ModifyGraph rgb('DC4.SA03008H.20180718.000029')=(17408,0,65280)\nX ModifyGraph rgb('DC5.SA03008H.20180718.000029')=(35840,0,65280)\nX ModifyGraph rgb('DC6.SA03008H.20180718.000029')=(54272,0,65280)\nX ModifyGraph rgb('DC7.SA03008H.20180718.000029')=(65280,0,58368)\nX Legend/C/N=text0/J \"\\\\s('time.SA03008H.20180718.000029') time\\r\\\\s('temp.SA03008H.20180718.000029') temp\\r\\\\s('B.SA03008H.20180718.000029') B\\r\\\\s('Vsource.SA03008H.20180718.000029') Vsource\\r\\\\s('Lockin0.SA03008H.20180718.000029') Lockin0\\r\\\\s('Lockin1.SA03008H.20180718.000029') Lockin1\\r\\\\s('Lockin2.SA03008H.20180718.000029') Lockin2\\r\\\\s('Lockin3.SA03008H.20180718.000029') Lockin3\\r\\\\s('Lockin4.SA03008H.20180718.000029') Lockin4\\r\\\\s('Lockin5.SA03008H.20180718.000029') Lockin5\\r\\\\s('B_rate.SA03008H.20180718.000029') B_rate\\r\\\\s('DC0.SA03008H.20180718.000029') DC0\\r\\\\s('DC1.SA03008H.20180718.000029') DC1\\r\\\\s('DC2.SA03008H.20180718.000029') DC2\\r\\\\s('DC3.SA03008H.20180718.000029') DC3\\r\\\\s('DC4.SA03008H.20180718.000029') DC4\\r\\\\s('DC5.SA03008H.20180718.000029') DC5\\r\\\\s('DC6.SA03008H.20180718.000029') DC6\\r\\\\s('DC7.SA03008H.20180718.000029') DC7\"\nX ModifyGraph mirror(bottom)=1\nX ModifyGraph width=216\nX ModifyGraph height={Aspect,0.6}\nX ModifyGraph Log(bottom)=0\nX ModifyGraph Log(left)=0\nX \n", "IGOR\nX// Date: 7/18/2018 5:24 PM\nX// SA03008H\nX// \nX// Source 2 Drain 28 (lockin 1 and 7)\nX// Slow sweeping BG -5 to 5 inc. 0.1V \nX// Fast sweep SG -1 to 1 inc. 0.05V\n\nX// DSA_Vsg1=0.500000\n\nX// \nX// B= 0.000000\n\n\n\n\n\n\n\n\n\n\n\n\n\n\n\n\n\n\n\n\n\n\n\n\n\n\n\n\n\n\n\n\n\n\n\n\n\n\n\n\nX \nX Display/R 'time.SA03008H.20180718.000030'\nX AppendToGraph 'temp.SA03008H.20180718.000030'\nX AppendToGraph 'B.SA03008H.20180718.000030'\nX AppendToGraph 'Vsource.SA03008H.20180718.000030'\nX AppendToGraph 'Lockin0.SA03008H.20180718.000030'\nX AppendToGraph 'Lockin1.SA03008H.20180718.000030'\nX AppendToGraph 'Lockin2.SA03008H.20180718.000030'\nX AppendToGraph 'Lockin3.SA03008H.20180718.000030'\nX AppendToGraph 'Lockin4.SA03008H.20180718.000030'\nX AppendToGraph 'Lockin5.SA03008H.20180718.000030'\nX AppendToGraph 'B_rate.SA03008H.20180718.000030'\nX AppendToGraph 'DC0.SA03008H.20180718.000030'\nX AppendToGraph 'DC1.SA03008H.20180718.000030'\nX AppendToGraph 'DC2.SA03008H.20180718.000030'\nX AppendToGraph 'DC3.SA03008H.20180718.000030'\nX AppendToGraph 'DC4.SA03008H.20180718.000030'\nX AppendToGraph 'DC5.SA03008H.20180718.000030'\nX AppendToGraph 'DC6.SA03008H.20180718.000030'\nX AppendToGraph 'DC7.SA03008H.20180718.000030'\nX Label bottom \"x label\"\nX Label left \"y label\"\nX ModifyGraph rgb('time.SA03008H.20180718.000030')=(65280,0,0)\nX ModifyGraph rgb('temp.SA03008H.20180718.000030')=(65280,18432,0)\nX ModifyGraph rgb('B.SA03008H.20180718.000030')=(65280,36864,0)\nX ModifyGraph rgb('Vsource.SA03008H.20180718.000030')=(65280,55296,0)\nX ModifyGraph rgb('Lockin0.SA03008H.20180718.000030')=(57344,65280,0)\nX ModifyGraph rgb('Lockin1.SA03008H.20180718.000030')=(37376,65280,0)\nX ModifyGraph rgb('Lockin2.SA03008H.20180718.000030')=(18944,65280,0)\nX ModifyGraph rgb('Lockin3.SA03008H.20180718.000030')=(512,65280,0)\nX ModifyGraph rgb('Lockin4.SA03008H.20180718.000030')=(0,65280,17920)\nX ModifyGraph rgb('Lockin5.SA03008H.20180718.000030')=(0,65280,36352)\nX ModifyGraph rgb('B_rate.SA03008H.20180718.000030')=(0,65280,54784)\nX ModifyGraph rgb('DC0.SA03008H.20180718.000030')=(0,57856,65280)\nX ModifyGraph rgb('DC1.SA03008H.20180718.000030')=(0,39424,65280)\nX ModifyGraph rgb('DC2.SA03008H.20180718.000030')=(0,20992,65280)\nX ModifyGraph rgb('DC3.SA03008H.20180718.000030')=(0,2560,65280)\nX ModifyGraph rgb('DC4.SA03008H.20180718.000030')=(17408,0,65280)\nX ModifyGraph rgb('DC5.SA03008H.20180718.000030')=(35840,0,65280)\nX ModifyGraph rgb('DC6.SA03008H.20180718.000030')=(54272,0,65280)\nX ModifyGraph rgb('DC7.SA03008H.20180718.000030')=(65280,0,58368)\nX Legend/C/N=text0/J \"\\\\s('time.SA03008H.20180718.000030') time\\r\\\\s('temp.SA03008H.20180718.000030') temp\\r\\\\s('B.SA03008H.20180718.000030') B\\r\\\\s('Vsource.SA03008H.20180718.000030') Vsource\\r\\\\s('Lockin0.SA03008H.20180718.000030') Lockin0\\r\\\\s('Lockin1.SA03008H.20180718.000030') Lockin1\\r\\\\s('Lockin2.SA03008H.20180718.000030') Lockin2\\r\\\\s('Lockin3.SA03008H.20180718.000030') Lockin3\\r\\\\s('Lockin4.SA03008H.20180718.000030') Lockin4\\r\\\\s('Lockin5.SA03008H.20180718.000030') Lockin5\\r\\\\s('B_rate.SA03008H.20180718.000030') B_rate\\r\\\\s('DC0.SA03008H.20180718.000030') DC0\\r\\\\s('DC1.SA03008H.20180718.000030') DC1\\r\\\\s('DC2.SA03008H.20180718.000030') DC2\\r\\\\s('DC3.SA03008H.20180718.000030') DC3\\r\\\\s('DC4.SA03008H.20180718.000030') DC4\\r\\\\s('DC5.SA03008H.20180718.000030') DC5\\r\\\\s('DC6.SA03008H.20180718.000030') DC6\\r\\\\s('DC7.SA03008H.20180718.000030') DC7\"\nX ModifyGraph mirror(bottom)=1\nX ModifyGraph width=216\nX ModifyGraph height={Aspect,0.6}\nX ModifyGraph Log(bottom)=0\nX ModifyGraph Log(left)=0\nX \n", "IGOR\nX// Date: 7/18/2018 5:24 PM\nX// SA03008H\nX// \nX// Source 2 Drain 28 (lockin 1 and 7)\nX// Slow sweeping BG -5 to 5 inc. 0.1V \nX// Fast sweep SG -1 to 1 inc. 0.05V\n\nX// DSA_Vsg1=0.550000\n\nX// \nX// B= 0.000000\n\n\n\n\n\n\n\n\n\n\n\n\n\n\n\n\n\n\n\n\n\n\n\n\n\n\n\n\n\n\n\n\n\n\n\n\n\n\n\n\nX \nX Display/R 'time.SA03008H.20180718.000031'\nX AppendToGraph 'temp.SA03008H.20180718.000031'\nX AppendToGraph 'B.SA03008H.20180718.000031'\nX AppendToGraph 'Vsource.SA03008H.20180718.000031'\nX AppendToGraph 'Lockin0.SA03008H.20180718.000031'\nX AppendToGraph 'Lockin1.SA03008H.20180718.000031'\nX AppendToGraph 'Lockin2.SA03008H.20180718.000031'\nX AppendToGraph 'Lockin3.SA03008H.20180718.000031'\nX AppendToGraph 'Lockin4.SA03008H.20180718.000031'\nX AppendToGraph 'Lockin5.SA03008H.20180718.000031'\nX AppendToGraph 'B_rate.SA03008H.20180718.000031'\nX AppendToGraph 'DC0.SA03008H.20180718.000031'\nX AppendToGraph 'DC1.SA03008H.20180718.000031'\nX AppendToGraph 'DC2.SA03008H.20180718.000031'\nX AppendToGraph 'DC3.SA03008H.20180718.000031'\nX AppendToGraph 'DC4.SA03008H.20180718.000031'\nX AppendToGraph 'DC5.SA03008H.20180718.000031'\nX AppendToGraph 'DC6.SA03008H.20180718.000031'\nX AppendToGraph 'DC7.SA03008H.20180718.000031'\nX Label bottom \"x label\"\nX Label left \"y label\"\nX ModifyGraph rgb('time.SA03008H.20180718.000031')=(65280,0,0)\nX ModifyGraph rgb('temp.SA03008H.20180718.000031')=(65280,18432,0)\nX ModifyGraph rgb('B.SA03008H.20180718.000031')=(65280,36864,0)\nX ModifyGraph rgb('Vsource.SA03008H.20180718.000031')=(65280,55296,0)\nX ModifyGraph rgb('Lockin0.SA03008H.20180718.000031')=(57344,65280,0)\nX ModifyGraph rgb('Lockin1.SA03008H.20180718.000031')=(37376,65280,0)\nX ModifyGraph rgb('Lockin2.SA03008H.20180718.000031')=(18944,65280,0)\nX ModifyGraph rgb('Lockin3.SA03008H.20180718.000031')=(512,65280,0)\nX ModifyGraph rgb('Lockin4.SA03008H.20180718.000031')=(0,65280,17920)\nX ModifyGraph rgb('Lockin5.SA03008H.20180718.000031')=(0,65280,36352)\nX ModifyGraph rgb('B_rate.SA03008H.20180718.000031')=(0,65280,54784)\nX ModifyGraph rgb('DC0.SA03008H.20180718.000031')=(0,57856,65280)\nX ModifyGraph rgb('DC1.SA03008H.20180718.000031')=(0,39424,65280)\nX ModifyGraph rgb('DC2.SA03008H.20180718.000031')=(0,20992,65280)\nX ModifyGraph rgb('DC3.SA03008H.20180718.000031')=(0,2560,65280)\nX ModifyGraph rgb('DC4.SA03008H.20180718.000031')=(17408,0,65280)\nX ModifyGraph rgb('DC5.SA03008H.20180718.000031')=(35840,0,65280)\nX ModifyGraph rgb('DC6.SA03008H.20180718.000031')=(54272,0,65280)\nX ModifyGraph rgb('DC7.SA03008H.20180718.000031')=(65280,0,58368)\nX Legend/C/N=text0/J \"\\\\s('time.SA03008H.20180718.000031') time\\r\\\\s('temp.SA03008H.20180718.000031') temp\\r\\\\s('B.SA03008H.20180718.000031') B\\r\\\\s('Vsource.SA03008H.20180718.000031') Vsource\\r\\\\s('Lockin0.SA03008H.20180718.000031') Lockin0\\r\\\\s('Lockin1.SA03008H.20180718.000031') Lockin1\\r\\\\s('Lockin2.SA03008H.20180718.000031') Lockin2\\r\\\\s('Lockin3.SA03008H.20180718.000031') Lockin3\\r\\\\s('Lockin4.SA03008H.20180718.000031') Lockin4\\r\\\\s('Lockin5.SA03008H.20180718.000031') Lockin5\\r\\\\s('B_rate.SA03008H.20180718.000031') B_rate\\r\\\\s('DC0.SA03008H.20180718.000031') DC0\\r\\\\s('DC1.SA03008H.20180718.000031') DC1\\r\\\\s('DC2.SA03008H.20180718.000031') DC2\\r\\\\s('DC3.SA03008H.20180718.000031') DC3\\r\\\\s('DC4.SA03008H.20180718.000031') DC4\\r\\\\s('DC5.SA03008H.20180718.000031') DC5\\r\\\\s('DC6.SA03008H.20180718.000031') DC6\\r\\\\s('DC7.SA03008H.20180718.000031') DC7\"\nX ModifyGraph mirror(bottom)=1\nX ModifyGraph width=216\nX ModifyGraph height={Aspect,0.6}\nX ModifyGraph Log(bottom)=0\nX ModifyGraph Log(left)=0\nX \n", "IGOR\nX// Date: 7/18/2018 5:25 PM\nX// SA03008H\nX// \nX// Source 2 Drain 28 (lockin 1 and 7)\nX// Slow sweeping BG -5 to 5 inc. 0.1V \nX// Fast sweep SG -1 to 1 inc. 0.05V\n\nX// DSA_Vsg1=0.600000\n\nX// \nX// B= 0.000000\n\n\n\n\n\n\n\n\n\n\n\n\n\n\n\n\n\n\n\n\n\n\n\n\n\n\n\n\n\n\n\n\n\n\n\n\n\n\n\n\nX \nX Display/R 'time.SA03008H.20180718.000032'\nX AppendToGraph 'temp.SA03008H.20180718.000032'\nX AppendToGraph 'B.SA03008H.20180718.000032'\nX AppendToGraph 'Vsource.SA03008H.20180718.000032'\nX AppendToGraph 'Lockin0.SA03008H.20180718.000032'\nX AppendToGraph 'Lockin1.SA03008H.20180718.000032'\nX AppendToGraph 'Lockin2.SA03008H.20180718.000032'\nX AppendToGraph 'Lockin3.SA03008H.20180718.000032'\nX AppendToGraph 'Lockin4.SA03008H.20180718.000032'\nX AppendToGraph 'Lockin5.SA03008H.20180718.000032'\nX AppendToGraph 'B_rate.SA03008H.20180718.000032'\nX AppendToGraph 'DC0.SA03008H.20180718.000032'\nX AppendToGraph 'DC1.SA03008H.20180718.000032'\nX AppendToGraph 'DC2.SA03008H.20180718.000032'\nX AppendToGraph 'DC3.SA03008H.20180718.000032'\nX AppendToGraph 'DC4.SA03008H.20180718.000032'\nX AppendToGraph 'DC5.SA03008H.20180718.000032'\nX AppendToGraph 'DC6.SA03008H.20180718.000032'\nX AppendToGraph 'DC7.SA03008H.20180718.000032'\nX Label bottom \"x label\"\nX Label left \"y label\"\nX ModifyGraph rgb('time.SA03008H.20180718.000032')=(65280,0,0)\nX ModifyGraph rgb('temp.SA03008H.20180718.000032')=(65280,18432,0)\nX ModifyGraph rgb('B.SA03008H.20180718.000032')=(65280,36864,0)\nX ModifyGraph rgb('Vsource.SA03008H.20180718.000032')=(65280,55296,0)\nX ModifyGraph rgb('Lockin0.SA03008H.20180718.000032')=(57344,65280,0)\nX ModifyGraph rgb('Lockin1.SA03008H.20180718.000032')=(37376,65280,0)\nX ModifyGraph rgb('Lockin2.SA03008H.20180718.000032')=(18944,65280,0)\nX ModifyGraph rgb('Lockin3.SA03008H.20180718.000032')=(512,65280,0)\nX ModifyGraph rgb('Lockin4.SA03008H.20180718.000032')=(0,65280,17920)\nX ModifyGraph rgb('Lockin5.SA03008H.20180718.000032')=(0,65280,36352)\nX ModifyGraph rgb('B_rate.SA03008H.20180718.000032')=(0,65280,54784)\nX ModifyGraph rgb('DC0.SA03008H.20180718.000032')=(0,57856,65280)\nX ModifyGraph rgb('DC1.SA03008H.20180718.000032')=(0,39424,65280)\nX ModifyGraph rgb('DC2.SA03008H.20180718.000032')=(0,20992,65280)\nX ModifyGraph rgb('DC3.SA03008H.20180718.000032')=(0,2560,65280)\nX ModifyGraph rgb('DC4.SA03008H.20180718.000032')=(17408,0,65280)\nX ModifyGraph rgb('DC5.SA03008H.20180718.000032')=(35840,0,65280)\nX ModifyGraph rgb('DC6.SA03008H.20180718.000032')=(54272,0,65280)\nX ModifyGraph rgb('DC7.SA03008H.20180718.000032')=(65280,0,58368)\nX Legend/C/N=text0/J \"\\\\s('time.SA03008H.20180718.000032') time\\r\\\\s('temp.SA03008H.20180718.000032') temp\\r\\\\s('B.SA03008H.20180718.000032') B\\r\\\\s('Vsource.SA03008H.20180718.000032') Vsource\\r\\\\s('Lockin0.SA03008H.20180718.000032') Lockin0\\r\\\\s('Lockin1.SA03008H.20180718.000032') Lockin1\\r\\\\s('Lockin2.SA03008H.20180718.000032') Lockin2\\r\\\\s('Lockin3.SA03008H.20180718.000032') Lockin3\\r\\\\s('Lockin4.SA03008H.20180718.000032') Lockin4\\r\\\\s('Lockin5.SA03008H.20180718.000032') Lockin5\\r\\\\s('B_rate.SA03008H.20180718.000032') B_rate\\r\\\\s('DC0.SA03008H.20180718.000032') DC0\\r\\\\s('DC1.SA03008H.20180718.000032') DC1\\r\\\\s('DC2.SA03008H.20180718.000032') DC2\\r\\\\s('DC3.SA03008H.20180718.000032') DC3\\r\\\\s('DC4.SA03008H.20180718.000032') DC4\\r\\\\s('DC5.SA03008H.20180718.000032') DC5\\r\\\\s('DC6.SA03008H.20180718.000032') DC6\\r\\\\s('DC7.SA03008H.20180718.000032') DC7\"\nX ModifyGraph mirror(bottom)=1\nX ModifyGraph width=216\nX ModifyGraph height={Aspect,0.6}\nX ModifyGraph Log(bottom)=0\nX ModifyGraph Log(left)=0\nX \n", "IGOR\nX// Date: 7/18/2018 5:25 PM\nX// SA03008H\nX// \nX// Source 2 Drain 28 (lockin 1 and 7)\nX// Slow sweeping BG -5 to 5 inc. 0.1V \nX// Fast sweep SG -1 to 1 inc. 0.05V\n\nX// DSA_Vsg1=0.650000\n\nX// \nX// B= 0.000000\n\n\n\n\n\n\n\n\n\n\n\n\n\n\n\n\n\n\n\n\n\n\n\n\n\n\n\n\n\n\n\n\n\n\n\n\n\n\n\n\nX \nX Display/R 'time.SA03008H.20180718.000033'\nX AppendToGraph 'temp.SA03008H.20180718.000033'\nX AppendToGraph 'B.SA03008H.20180718.000033'\nX AppendToGraph 'Vsource.SA03008H.20180718.000033'\nX AppendToGraph 'Lockin0.SA03008H.20180718.000033'\nX AppendToGraph 'Lockin1.SA03008H.20180718.000033'\nX AppendToGraph 'Lockin2.SA03008H.20180718.000033'\nX AppendToGraph 'Lockin3.SA03008H.20180718.000033'\nX AppendToGraph 'Lockin4.SA03008H.20180718.000033'\nX AppendToGraph 'Lockin5.SA03008H.20180718.000033'\nX AppendToGraph 'B_rate.SA03008H.20180718.000033'\nX AppendToGraph 'DC0.SA03008H.20180718.000033'\nX AppendToGraph 'DC1.SA03008H.20180718.000033'\nX AppendToGraph 'DC2.SA03008H.20180718.000033'\nX AppendToGraph 'DC3.SA03008H.20180718.000033'\nX AppendToGraph 'DC4.SA03008H.20180718.000033'\nX AppendToGraph 'DC5.SA03008H.20180718.000033'\nX AppendToGraph 'DC6.SA03008H.20180718.000033'\nX AppendToGraph 'DC7.SA03008H.20180718.000033'\nX Label bottom \"x label\"\nX Label left \"y label\"\nX ModifyGraph rgb('time.SA03008H.20180718.000033')=(65280,0,0)\nX ModifyGraph rgb('temp.SA03008H.20180718.000033')=(65280,18432,0)\nX ModifyGraph rgb('B.SA03008H.20180718.000033')=(65280,36864,0)\nX ModifyGraph rgb('Vsource.SA03008H.20180718.000033')=(65280,55296,0)\nX ModifyGraph rgb('Lockin0.SA03008H.20180718.000033')=(57344,65280,0)\nX ModifyGraph rgb('Lockin1.SA03008H.20180718.000033')=(37376,65280,0)\nX ModifyGraph rgb('Lockin2.SA03008H.20180718.000033')=(18944,65280,0)\nX ModifyGraph rgb('Lockin3.SA03008H.20180718.000033')=(512,65280,0)\nX ModifyGraph rgb('Lockin4.SA03008H.20180718.000033')=(0,65280,17920)\nX ModifyGraph rgb('Lockin5.SA03008H.20180718.000033')=(0,65280,36352)\nX ModifyGraph rgb('B_rate.SA03008H.20180718.000033')=(0,65280,54784)\nX ModifyGraph rgb('DC0.SA03008H.20180718.000033')=(0,57856,65280)\nX ModifyGraph rgb('DC1.SA03008H.20180718.000033')=(0,39424,65280)\nX ModifyGraph rgb('DC2.SA03008H.20180718.000033')=(0,20992,65280)\nX ModifyGraph rgb('DC3.SA03008H.20180718.000033')=(0,2560,65280)\nX ModifyGraph rgb('DC4.SA03008H.20180718.000033')=(17408,0,65280)\nX ModifyGraph rgb('DC5.SA03008H.20180718.000033')=(35840,0,65280)\nX ModifyGraph rgb('DC6.SA03008H.20180718.000033')=(54272,0,65280)\nX ModifyGraph rgb('DC7.SA03008H.20180718.000033')=(65280,0,58368)\nX Legend/C/N=text0/J \"\\\\s('time.SA03008H.20180718.000033') time\\r\\\\s('temp.SA03008H.20180718.000033') temp\\r\\\\s('B.SA03008H.20180718.000033') B\\r\\\\s('Vsource.SA03008H.20180718.000033') Vsource\\r\\\\s('Lockin0.SA03008H.20180718.000033') Lockin0\\r\\\\s('Lockin1.SA03008H.20180718.000033') Lockin1\\r\\\\s('Lockin2.SA03008H.20180718.000033') Lockin2\\r\\\\s('Lockin3.SA03008H.20180718.000033') Lockin3\\r\\\\s('Lockin4.SA03008H.20180718.000033') Lockin4\\r\\\\s('Lockin5.SA03008H.20180718.000033') Lockin5\\r\\\\s('B_rate.SA03008H.20180718.000033') B_rate\\r\\\\s('DC0.SA03008H.20180718.000033') DC0\\r\\\\s('DC1.SA03008H.20180718.000033') DC1\\r\\\\s('DC2.SA03008H.20180718.000033') DC2\\r\\\\s('DC3.SA03008H.20180718.000033') DC3\\r\\\\s('DC4.SA03008H.20180718.000033') DC4\\r\\\\s('DC5.SA03008H.20180718.000033') DC5\\r\\\\s('DC6.SA03008H.20180718.000033') DC6\\r\\\\s('DC7.SA03008H.20180718.000033') DC7\"\nX ModifyGraph mirror(bottom)=1\nX ModifyGraph width=216\nX ModifyGraph height={Aspect,0.6}\nX ModifyGraph Log(bottom)=0\nX ModifyGraph Log(left)=0\nX \n", "IGOR\nX// Date: 7/18/2018 5:25 PM\nX// SA03008H\nX// \nX// Source 2 Drain 28 (lockin 1 and 7)\nX// Slow sweeping BG -5 to 5 inc. 0.1V \nX// Fast sweep SG -1 to 1 inc. 0.05V\n\nX// DSA_Vsg1=0.700000\n\nX// \nX// B= 0.000000\n\n\n\n\n\n\n\n\n\n\n\n\n\n\n\n\n\n\n\n\n\n\n\n\n\n\n\n\n\n\n\n\n\n\n\n\n\n\n\n\nX \nX Display/R 'time.SA03008H.20180718.000034'\nX AppendToGraph 'temp.SA03008H.20180718.000034'\nX AppendToGraph 'B.SA03008H.20180718.000034'\nX AppendToGraph 'Vsource.SA03008H.20180718.000034'\nX AppendToGraph 'Lockin0.SA03008H.20180718.000034'\nX AppendToGraph 'Lockin1.SA03008H.20180718.000034'\nX AppendToGraph 'Lockin2.SA03008H.20180718.000034'\nX AppendToGraph 'Lockin3.SA03008H.20180718.000034'\nX AppendToGraph 'Lockin4.SA03008H.20180718.000034'\nX AppendToGraph 'Lockin5.SA03008H.20180718.000034'\nX AppendToGraph 'B_rate.SA03008H.20180718.000034'\nX AppendToGraph 'DC0.SA03008H.20180718.000034'\nX AppendToGraph 'DC1.SA03008H.20180718.000034'\nX AppendToGraph 'DC2.SA03008H.20180718.000034'\nX AppendToGraph 'DC3.SA03008H.20180718.000034'\nX AppendToGraph 'DC4.SA03008H.20180718.000034'\nX AppendToGraph 'DC5.SA03008H.20180718.000034'\nX AppendToGraph 'DC6.SA03008H.20180718.000034'\nX AppendToGraph 'DC7.SA03008H.20180718.000034'\nX Label bottom \"x label\"\nX Label left \"y label\"\nX ModifyGraph rgb('time.SA03008H.20180718.000034')=(65280,0,0)\nX ModifyGraph rgb('temp.SA03008H.20180718.000034')=(65280,18432,0)\nX ModifyGraph rgb('B.SA03008H.20180718.000034')=(65280,36864,0)\nX ModifyGraph rgb('Vsource.SA03008H.20180718.000034')=(65280,55296,0)\nX ModifyGraph rgb('Lockin0.SA03008H.20180718.000034')=(57344,65280,0)\nX ModifyGraph rgb('Lockin1.SA03008H.20180718.000034')=(37376,65280,0)\nX ModifyGraph rgb('Lockin2.SA03008H.20180718.000034')=(18944,65280,0)\nX ModifyGraph rgb('Lockin3.SA03008H.20180718.000034')=(512,65280,0)\nX ModifyGraph rgb('Lockin4.SA03008H.20180718.000034')=(0,65280,17920)\nX ModifyGraph rgb('Lockin5.SA03008H.20180718.000034')=(0,65280,36352)\nX ModifyGraph rgb('B_rate.SA03008H.20180718.000034')=(0,65280,54784)\nX ModifyGraph rgb('DC0.SA03008H.20180718.000034')=(0,57856,65280)\nX ModifyGraph rgb('DC1.SA03008H.20180718.000034')=(0,39424,65280)\nX ModifyGraph rgb('DC2.SA03008H.20180718.000034')=(0,20992,65280)\nX ModifyGraph rgb('DC3.SA03008H.20180718.000034')=(0,2560,65280)\nX ModifyGraph rgb('DC4.SA03008H.20180718.000034')=(17408,0,65280)\nX ModifyGraph rgb('DC5.SA03008H.20180718.000034')=(35840,0,65280)\nX ModifyGraph rgb('DC6.SA03008H.20180718.000034')=(54272,0,65280)\nX ModifyGraph rgb('DC7.SA03008H.20180718.000034')=(65280,0,58368)\nX Legend/C/N=text0/J \"\\\\s('time.SA03008H.20180718.000034') time\\r\\\\s('temp.SA03008H.20180718.000034') temp\\r\\\\s('B.SA03008H.20180718.000034') B\\r\\\\s('Vsource.SA03008H.20180718.000034') Vsource\\r\\\\s('Lockin0.SA03008H.20180718.000034') Lockin0\\r\\\\s('Lockin1.SA03008H.20180718.000034') Lockin1\\r\\\\s('Lockin2.SA03008H.20180718.000034') Lockin2\\r\\\\s('Lockin3.SA03008H.20180718.000034') Lockin3\\r\\\\s('Lockin4.SA03008H.20180718.000034') Lockin4\\r\\\\s('Lockin5.SA03008H.20180718.000034') Lockin5\\r\\\\s('B_rate.SA03008H.20180718.000034') B_rate\\r\\\\s('DC0.SA03008H.20180718.000034') DC0\\r\\\\s('DC1.SA03008H.20180718.000034') DC1\\r\\\\s('DC2.SA03008H.20180718.000034') DC2\\r\\\\s('DC3.SA03008H.20180718.000034') DC3\\r\\\\s('DC4.SA03008H.20180718.000034') DC4\\r\\\\s('DC5.SA03008H.20180718.000034') DC5\\r\\\\s('DC6.SA03008H.20180718.000034') DC6\\r\\\\s('DC7.SA03008H.20180718.000034') DC7\"\nX ModifyGraph mirror(bottom)=1\nX ModifyGraph width=216\nX ModifyGraph height={Aspect,0.6}\nX ModifyGraph Log(bottom)=0\nX ModifyGraph Log(left)=0\nX \n", "IGOR\nX// Date: 7/18/2018 5:25 PM\nX// SA03008H\nX// \nX// Source 2 Drain 28 (lockin 1 and 7)\nX// Slow sweeping BG -5 to 5 inc. 0.1V \nX// Fast sweep SG -1 to 1 inc. 0.05V\n\nX// DSA_Vsg1=0.750000\n\nX// \nX// B= 0.000000\n\n\n\n\n\n\n\n\n\n\n\n\n\n\n\n\n\n\n\n\n\n\n\n\n\n\n\n\n\n\n\n\n\n\n\n\n\n\n\n\nX \nX Display/R 'time.SA03008H.20180718.000035'\nX AppendToGraph 'temp.SA03008H.20180718.000035'\nX AppendToGraph 'B.SA03008H.20180718.000035'\nX AppendToGraph 'Vsource.SA03008H.20180718.000035'\nX AppendToGraph 'Lockin0.SA03008H.20180718.000035'\nX AppendToGraph 'Lockin1.SA03008H.20180718.000035'\nX AppendToGraph 'Lockin2.SA03008H.20180718.000035'\nX AppendToGraph 'Lockin3.SA03008H.20180718.000035'\nX AppendToGraph 'Lockin4.SA03008H.20180718.000035'\nX AppendToGraph 'Lockin5.SA03008H.20180718.000035'\nX AppendToGraph 'B_rate.SA03008H.20180718.000035'\nX AppendToGraph 'DC0.SA03008H.20180718.000035'\nX AppendToGraph 'DC1.SA03008H.20180718.000035'\nX AppendToGraph 'DC2.SA03008H.20180718.000035'\nX AppendToGraph 'DC3.SA03008H.20180718.000035'\nX AppendToGraph 'DC4.SA03008H.20180718.000035'\nX AppendToGraph 'DC5.SA03008H.20180718.000035'\nX AppendToGraph 'DC6.SA03008H.20180718.000035'\nX AppendToGraph 'DC7.SA03008H.20180718.000035'\nX Label bottom \"x label\"\nX Label left \"y label\"\nX ModifyGraph rgb('time.SA03008H.20180718.000035')=(65280,0,0)\nX ModifyGraph rgb('temp.SA03008H.20180718.000035')=(65280,18432,0)\nX ModifyGraph rgb('B.SA03008H.20180718.000035')=(65280,36864,0)\nX ModifyGraph rgb('Vsource.SA03008H.20180718.000035')=(65280,55296,0)\nX ModifyGraph rgb('Lockin0.SA03008H.20180718.000035')=(57344,65280,0)\nX ModifyGraph rgb('Lockin1.SA03008H.20180718.000035')=(37376,65280,0)\nX ModifyGraph rgb('Lockin2.SA03008H.20180718.000035')=(18944,65280,0)\nX ModifyGraph rgb('Lockin3.SA03008H.20180718.000035')=(512,65280,0)\nX ModifyGraph rgb('Lockin4.SA03008H.20180718.000035')=(0,65280,17920)\nX ModifyGraph rgb('Lockin5.SA03008H.20180718.000035')=(0,65280,36352)\nX ModifyGraph rgb('B_rate.SA03008H.20180718.000035')=(0,65280,54784)\nX ModifyGraph rgb('DC0.SA03008H.20180718.000035')=(0,57856,65280)\nX ModifyGraph rgb('DC1.SA03008H.20180718.000035')=(0,39424,65280)\nX ModifyGraph rgb('DC2.SA03008H.20180718.000035')=(0,20992,65280)\nX ModifyGraph rgb('DC3.SA03008H.20180718.000035')=(0,2560,65280)\nX ModifyGraph rgb('DC4.SA03008H.20180718.000035')=(17408,0,65280)\nX ModifyGraph rgb('DC5.SA03008H.20180718.000035')=(35840,0,65280)\nX ModifyGraph rgb('DC6.SA03008H.20180718.000035')=(54272,0,65280)\nX ModifyGraph rgb('DC7.SA03008H.20180718.000035')=(65280,0,58368)\nX Legend/C/N=text0/J \"\\\\s('time.SA03008H.20180718.000035') time\\r\\\\s('temp.SA03008H.20180718.000035') temp\\r\\\\s('B.SA03008H.20180718.000035') B\\r\\\\s('Vsource.SA03008H.20180718.000035') Vsource\\r\\\\s('Lockin0.SA03008H.20180718.000035') Lockin0\\r\\\\s('Lockin1.SA03008H.20180718.000035') Lockin1\\r\\\\s('Lockin2.SA03008H.20180718.000035') Lockin2\\r\\\\s('Lockin3.SA03008H.20180718.000035') Lockin3\\r\\\\s('Lockin4.SA03008H.20180718.000035') Lockin4\\r\\\\s('Lockin5.SA03008H.20180718.000035') Lockin5\\r\\\\s('B_rate.SA03008H.20180718.000035') B_rate\\r\\\\s('DC0.SA03008H.20180718.000035') DC0\\r\\\\s('DC1.SA03008H.20180718.000035') DC1\\r\\\\s('DC2.SA03008H.20180718.000035') DC2\\r\\\\s('DC3.SA03008H.20180718.000035') DC3\\r\\\\s('DC4.SA03008H.20180718.000035') DC4\\r\\\\s('DC5.SA03008H.20180718.000035') DC5\\r\\\\s('DC6.SA03008H.20180718.000035') DC6\\r\\\\s('DC7.SA03008H.20180718.000035') DC7\"\nX ModifyGraph mirror(bottom)=1\nX ModifyGraph width=216\nX ModifyGraph height={Aspect,0.6}\nX ModifyGraph Log(bottom)=0\nX ModifyGraph Log(left)=0\nX \n", "IGOR\nX// Date: 7/18/2018 5:25 PM\nX// SA03008H\nX// \nX// Source 2 Drain 28 (lockin 1 and 7)\nX// Slow sweeping BG -5 to 5 inc. 0.1V \nX// Fast sweep SG -1 to 1 inc. 0.05V\n\nX// DSA_Vsg1=0.800000\n\nX// \nX// B= 0.000000\n\n\n\n\n\n\n\n\n\n\n\n\n\n\n\n\n\n\n\n\n\n\n\n\n\n\n\n\n\n\n\n\n\n\n\n\n\n\n\n\nX \nX Display/R 'time.SA03008H.20180718.000036'\nX AppendToGraph 'temp.SA03008H.20180718.000036'\nX AppendToGraph 'B.SA03008H.20180718.000036'\nX AppendToGraph 'Vsource.SA03008H.20180718.000036'\nX AppendToGraph 'Lockin0.SA03008H.20180718.000036'\nX AppendToGraph 'Lockin1.SA03008H.20180718.000036'\nX AppendToGraph 'Lockin2.SA03008H.20180718.000036'\nX AppendToGraph 'Lockin3.SA03008H.20180718.000036'\nX AppendToGraph 'Lockin4.SA03008H.20180718.000036'\nX AppendToGraph 'Lockin5.SA03008H.20180718.000036'\nX AppendToGraph 'B_rate.SA03008H.20180718.000036'\nX AppendToGraph 'DC0.SA03008H.20180718.000036'\nX AppendToGraph 'DC1.SA03008H.20180718.000036'\nX AppendToGraph 'DC2.SA03008H.20180718.000036'\nX AppendToGraph 'DC3.SA03008H.20180718.000036'\nX AppendToGraph 'DC4.SA03008H.20180718.000036'\nX AppendToGraph 'DC5.SA03008H.20180718.000036'\nX AppendToGraph 'DC6.SA03008H.20180718.000036'\nX AppendToGraph 'DC7.SA03008H.20180718.000036'\nX Label bottom \"x label\"\nX Label left \"y label\"\nX ModifyGraph rgb('time.SA03008H.20180718.000036')=(65280,0,0)\nX ModifyGraph rgb('temp.SA03008H.20180718.000036')=(65280,18432,0)\nX ModifyGraph rgb('B.SA03008H.20180718.000036')=(65280,36864,0)\nX ModifyGraph rgb('Vsource.SA03008H.20180718.000036')=(65280,55296,0)\nX ModifyGraph rgb('Lockin0.SA03008H.20180718.000036')=(57344,65280,0)\nX ModifyGraph rgb('Lockin1.SA03008H.20180718.000036')=(37376,65280,0)\nX ModifyGraph rgb('Lockin2.SA03008H.20180718.000036')=(18944,65280,0)\nX ModifyGraph rgb('Lockin3.SA03008H.20180718.000036')=(512,65280,0)\nX ModifyGraph rgb('Lockin4.SA03008H.20180718.000036')=(0,65280,17920)\nX ModifyGraph rgb('Lockin5.SA03008H.20180718.000036')=(0,65280,36352)\nX ModifyGraph rgb('B_rate.SA03008H.20180718.000036')=(0,65280,54784)\nX ModifyGraph rgb('DC0.SA03008H.20180718.000036')=(0,57856,65280)\nX ModifyGraph rgb('DC1.SA03008H.20180718.000036')=(0,39424,65280)\nX ModifyGraph rgb('DC2.SA03008H.20180718.000036')=(0,20992,65280)\nX ModifyGraph rgb('DC3.SA03008H.20180718.000036')=(0,2560,65280)\nX ModifyGraph rgb('DC4.SA03008H.20180718.000036')=(17408,0,65280)\nX ModifyGraph rgb('DC5.SA03008H.20180718.000036')=(35840,0,65280)\nX ModifyGraph rgb('DC6.SA03008H.20180718.000036')=(54272,0,65280)\nX ModifyGraph rgb('DC7.SA03008H.20180718.000036')=(65280,0,58368)\nX Legend/C/N=text0/J \"\\\\s('time.SA03008H.20180718.000036') time\\r\\\\s('temp.SA03008H.20180718.000036') temp\\r\\\\s('B.SA03008H.20180718.000036') B\\r\\\\s('Vsource.SA03008H.20180718.000036') Vsource\\r\\\\s('Lockin0.SA03008H.20180718.000036') Lockin0\\r\\\\s('Lockin1.SA03008H.20180718.000036') Lockin1\\r\\\\s('Lockin2.SA03008H.20180718.000036') Lockin2\\r\\\\s('Lockin3.SA03008H.20180718.000036') Lockin3\\r\\\\s('Lockin4.SA03008H.20180718.000036') Lockin4\\r\\\\s('Lockin5.SA03008H.20180718.000036') Lockin5\\r\\\\s('B_rate.SA03008H.20180718.000036') B_rate\\r\\\\s('DC0.SA03008H.20180718.000036') DC0\\r\\\\s('DC1.SA03008H.20180718.000036') DC1\\r\\\\s('DC2.SA03008H.20180718.000036') DC2\\r\\\\s('DC3.SA03008H.20180718.000036') DC3\\r\\\\s('DC4.SA03008H.20180718.000036') DC4\\r\\\\s('DC5.SA03008H.20180718.000036') DC5\\r\\\\s('DC6.SA03008H.20180718.000036') DC6\\r\\\\s('DC7.SA03008H.20180718.000036') DC7\"\nX ModifyGraph mirror(bottom)=1\nX ModifyGraph width=216\nX ModifyGraph height={Aspect,0.6}\nX ModifyGraph Log(bottom)=0\nX ModifyGraph Log(left)=0\nX \n", "IGOR\nX// Date: 7/18/2018 5:26 PM\nX// SA03008H\nX// \nX// Source 2 Drain 28 (lockin 1 and 7)\nX// Slow sweeping BG -5 to 5 inc. 0.1V \nX// Fast sweep SG -1 to 1 inc. 0.05V\n\nX// DSA_Vsg1=0.850000\n\nX// \nX// B= 0.000000\n\n\n\n\n\n\n\n\n\n\n\n\n\n\n\n\n\n\n\n\n\n\n\n\n\n\n\n\n\n\n\n\n\n\n\n\n\n\n\n\nX \nX Display/R 'time.SA03008H.20180718.000037'\nX AppendToGraph 'temp.SA03008H.20180718.000037'\nX AppendToGraph 'B.SA03008H.20180718.000037'\nX AppendToGraph 'Vsource.SA03008H.20180718.000037'\nX AppendToGraph 'Lockin0.SA03008H.20180718.000037'\nX AppendToGraph 'Lockin1.SA03008H.20180718.000037'\nX AppendToGraph 'Lockin2.SA03008H.20180718.000037'\nX AppendToGraph 'Lockin3.SA03008H.20180718.000037'\nX AppendToGraph 'Lockin4.SA03008H.20180718.000037'\nX AppendToGraph 'Lockin5.SA03008H.20180718.000037'\nX AppendToGraph 'B_rate.SA03008H.20180718.000037'\nX AppendToGraph 'DC0.SA03008H.20180718.000037'\nX AppendToGraph 'DC1.SA03008H.20180718.000037'\nX AppendToGraph 'DC2.SA03008H.20180718.000037'\nX AppendToGraph 'DC3.SA03008H.20180718.000037'\nX AppendToGraph 'DC4.SA03008H.20180718.000037'\nX AppendToGraph 'DC5.SA03008H.20180718.000037'\nX AppendToGraph 'DC6.SA03008H.20180718.000037'\nX AppendToGraph 'DC7.SA03008H.20180718.000037'\nX Label bottom \"x label\"\nX Label left \"y label\"\nX ModifyGraph rgb('time.SA03008H.20180718.000037')=(65280,0,0)\nX ModifyGraph rgb('temp.SA03008H.20180718.000037')=(65280,18432,0)\nX ModifyGraph rgb('B.SA03008H.20180718.000037')=(65280,36864,0)\nX ModifyGraph rgb('Vsource.SA03008H.20180718.000037')=(65280,55296,0)\nX ModifyGraph rgb('Lockin0.SA03008H.20180718.000037')=(57344,65280,0)\nX ModifyGraph rgb('Lockin1.SA03008H.20180718.000037')=(37376,65280,0)\nX ModifyGraph rgb('Lockin2.SA03008H.20180718.000037')=(18944,65280,0)\nX ModifyGraph rgb('Lockin3.SA03008H.20180718.000037')=(512,65280,0)\nX ModifyGraph rgb('Lockin4.SA03008H.20180718.000037')=(0,65280,17920)\nX ModifyGraph rgb('Lockin5.SA03008H.20180718.000037')=(0,65280,36352)\nX ModifyGraph rgb('B_rate.SA03008H.20180718.000037')=(0,65280,54784)\nX ModifyGraph rgb('DC0.SA03008H.20180718.000037')=(0,57856,65280)\nX ModifyGraph rgb('DC1.SA03008H.20180718.000037')=(0,39424,65280)\nX ModifyGraph rgb('DC2.SA03008H.20180718.000037')=(0,20992,65280)\nX ModifyGraph rgb('DC3.SA03008H.20180718.000037')=(0,2560,65280)\nX ModifyGraph rgb('DC4.SA03008H.20180718.000037')=(17408,0,65280)\nX ModifyGraph rgb('DC5.SA03008H.20180718.000037')=(35840,0,65280)\nX ModifyGraph rgb('DC6.SA03008H.20180718.000037')=(54272,0,65280)\nX ModifyGraph rgb('DC7.SA03008H.20180718.000037')=(65280,0,58368)\nX Legend/C/N=text0/J \"\\\\s('time.SA03008H.20180718.000037') time\\r\\\\s('temp.SA03008H.20180718.000037') temp\\r\\\\s('B.SA03008H.20180718.000037') B\\r\\\\s('Vsource.SA03008H.20180718.000037') Vsource\\r\\\\s('Lockin0.SA03008H.20180718.000037') Lockin0\\r\\\\s('Lockin1.SA03008H.20180718.000037') Lockin1\\r\\\\s('Lockin2.SA03008H.20180718.000037') Lockin2\\r\\\\s('Lockin3.SA03008H.20180718.000037') Lockin3\\r\\\\s('Lockin4.SA03008H.20180718.000037') Lockin4\\r\\\\s('Lockin5.SA03008H.20180718.000037') Lockin5\\r\\\\s('B_rate.SA03008H.20180718.000037') B_rate\\r\\\\s('DC0.SA03008H.20180718.000037') DC0\\r\\\\s('DC1.SA03008H.20180718.000037') DC1\\r\\\\s('DC2.SA03008H.20180718.000037') DC2\\r\\\\s('DC3.SA03008H.20180718.000037') DC3\\r\\\\s('DC4.SA03008H.20180718.000037') DC4\\r\\\\s('DC5.SA03008H.20180718.000037') DC5\\r\\\\s('DC6.SA03008H.20180718.000037') DC6\\r\\\\s('DC7.SA03008H.20180718.000037') DC7\"\nX ModifyGraph mirror(bottom)=1\nX ModifyGraph width=216\nX ModifyGraph height={Aspect,0.6}\nX ModifyGraph Log(bottom)=0\nX ModifyGraph Log(left)=0\nX \n", "IGOR\nX// Date: 7/18/2018 5:26 PM\nX// SA03008H\nX// \nX// Source 2 Drain 28 (lockin 1 and 7)\nX// Slow sweeping BG -5 to 5 inc. 0.1V \nX// Fast sweep SG -1 to 1 inc. 0.05V\n\nX// DSA_Vsg1=0.900000\n\nX// \nX// B= 0.000000\n\n\n\n\n\n\n\n\n\n\n\n\n\n\n\n\n\n\n\n\n\n\n\n\n\n\n\n\n\n\n\n\n\n\n\n\n\n\n\n\nX \nX Display/R 'time.SA03008H.20180718.000038'\nX AppendToGraph 'temp.SA03008H.20180718.000038'\nX AppendToGraph 'B.SA03008H.20180718.000038'\nX AppendToGraph 'Vsource.SA03008H.20180718.000038'\nX AppendToGraph 'Lockin0.SA03008H.20180718.000038'\nX AppendToGraph 'Lockin1.SA03008H.20180718.000038'\nX AppendToGraph 'Lockin2.SA03008H.20180718.000038'\nX AppendToGraph 'Lockin3.SA03008H.20180718.000038'\nX AppendToGraph 'Lockin4.SA03008H.20180718.000038'\nX AppendToGraph 'Lockin5.SA03008H.20180718.000038'\nX AppendToGraph 'B_rate.SA03008H.20180718.000038'\nX AppendToGraph 'DC0.SA03008H.20180718.000038'\nX AppendToGraph 'DC1.SA03008H.20180718.000038'\nX AppendToGraph 'DC2.SA03008H.20180718.000038'\nX AppendToGraph 'DC3.SA03008H.20180718.000038'\nX AppendToGraph 'DC4.SA03008H.20180718.000038'\nX AppendToGraph 'DC5.SA03008H.20180718.000038'\nX AppendToGraph 'DC6.SA03008H.20180718.000038'\nX AppendToGraph 'DC7.SA03008H.20180718.000038'\nX Label bottom \"x label\"\nX Label left \"y label\"\nX ModifyGraph rgb('time.SA03008H.20180718.000038')=(65280,0,0)\nX ModifyGraph rgb('temp.SA03008H.20180718.000038')=(65280,18432,0)\nX ModifyGraph rgb('B.SA03008H.20180718.000038')=(65280,36864,0)\nX ModifyGraph rgb('Vsource.SA03008H.20180718.000038')=(65280,55296,0)\nX ModifyGraph rgb('Lockin0.SA03008H.20180718.000038')=(57344,65280,0)\nX ModifyGraph rgb('Lockin1.SA03008H.20180718.000038')=(37376,65280,0)\nX ModifyGraph rgb('Lockin2.SA03008H.20180718.000038')=(18944,65280,0)\nX ModifyGraph rgb('Lockin3.SA03008H.20180718.000038')=(512,65280,0)\nX ModifyGraph rgb('Lockin4.SA03008H.20180718.000038')=(0,65280,17920)\nX ModifyGraph rgb('Lockin5.SA03008H.20180718.000038')=(0,65280,36352)\nX ModifyGraph rgb('B_rate.SA03008H.20180718.000038')=(0,65280,54784)\nX ModifyGraph rgb('DC0.SA03008H.20180718.000038')=(0,57856,65280)\nX ModifyGraph rgb('DC1.SA03008H.20180718.000038')=(0,39424,65280)\nX ModifyGraph rgb('DC2.SA03008H.20180718.000038')=(0,20992,65280)\nX ModifyGraph rgb('DC3.SA03008H.20180718.000038')=(0,2560,65280)\nX ModifyGraph rgb('DC4.SA03008H.20180718.000038')=(17408,0,65280)\nX ModifyGraph rgb('DC5.SA03008H.20180718.000038')=(35840,0,65280)\nX ModifyGraph rgb('DC6.SA03008H.20180718.000038')=(54272,0,65280)\nX ModifyGraph rgb('DC7.SA03008H.20180718.000038')=(65280,0,58368)\nX Legend/C/N=text0/J \"\\\\s('time.SA03008H.20180718.000038') time\\r\\\\s('temp.SA03008H.20180718.000038') temp\\r\\\\s('B.SA03008H.20180718.000038') B\\r\\\\s('Vsource.SA03008H.20180718.000038') Vsource\\r\\\\s('Lockin0.SA03008H.20180718.000038') Lockin0\\r\\\\s('Lockin1.SA03008H.20180718.000038') Lockin1\\r\\\\s('Lockin2.SA03008H.20180718.000038') Lockin2\\r\\\\s('Lockin3.SA03008H.20180718.000038') Lockin3\\r\\\\s('Lockin4.SA03008H.20180718.000038') Lockin4\\r\\\\s('Lockin5.SA03008H.20180718.000038') Lockin5\\r\\\\s('B_rate.SA03008H.20180718.000038') B_rate\\r\\\\s('DC0.SA03008H.20180718.000038') DC0\\r\\\\s('DC1.SA03008H.20180718.000038') DC1\\r\\\\s('DC2.SA03008H.20180718.000038') DC2\\r\\\\s('DC3.SA03008H.20180718.000038') DC3\\r\\\\s('DC4.SA03008H.20180718.000038') DC4\\r\\\\s('DC5.SA03008H.20180718.000038') DC5\\r\\\\s('DC6.SA03008H.20180718.000038') DC6\\r\\\\s('DC7.SA03008H.20180718.000038') DC7\"\nX ModifyGraph mirror(bottom)=1\nX ModifyGraph width=216\nX ModifyGraph height={Aspect,0.6}\nX ModifyGraph Log(bottom)=0\nX ModifyGraph Log(left)=0\nX \n", "IGOR\nX// Date: 7/18/2018 5:26 PM\nX// SA03008H\nX// \nX// Source 2 Drain 28 (lockin 1 and 7)\nX// Slow sweeping BG -5 to 5 inc. 0.1V \nX// Fast sweep SG -1 to 1 inc. 0.05V\n\nX// DSA_Vsg1=0.950000\n\nX// \nX// B= 0.000000\n\n\n\n\n\n\n\n\n\n\n\n\n\n\n\n\n\n\n\n\n\n\n\n\n\n\n\n\n\n\n\n\n\n\n\n\n\n\n\n\nX \nX Display/R 'time.SA03008H.20180718.000039'\nX AppendToGraph 'temp.SA03008H.20180718.000039'\nX AppendToGraph 'B.SA03008H.20180718.000039'\nX AppendToGraph 'Vsource.SA03008H.20180718.000039'\nX AppendToGraph 'Lockin0.SA03008H.20180718.000039'\nX AppendToGraph 'Lockin1.SA03008H.20180718.000039'\nX AppendToGraph 'Lockin2.SA03008H.20180718.000039'\nX AppendToGraph 'Lockin3.SA03008H.20180718.000039'\nX AppendToGraph 'Lockin4.SA03008H.20180718.000039'\nX AppendToGraph 'Lockin5.SA03008H.20180718.000039'\nX AppendToGraph 'B_rate.SA03008H.20180718.000039'\nX AppendToGraph 'DC0.SA03008H.20180718.000039'\nX AppendToGraph 'DC1.SA03008H.20180718.000039'\nX AppendToGraph 'DC2.SA03008H.20180718.000039'\nX AppendToGraph 'DC3.SA03008H.20180718.000039'\nX AppendToGraph 'DC4.SA03008H.20180718.000039'\nX AppendToGraph 'DC5.SA03008H.20180718.000039'\nX AppendToGraph 'DC6.SA03008H.20180718.000039'\nX AppendToGraph 'DC7.SA03008H.20180718.000039'\nX Label bottom \"x label\"\nX Label left \"y label\"\nX ModifyGraph rgb('time.SA03008H.20180718.000039')=(65280,0,0)\nX ModifyGraph rgb('temp.SA03008H.20180718.000039')=(65280,18432,0)\nX ModifyGraph rgb('B.SA03008H.20180718.000039')=(65280,36864,0)\nX ModifyGraph rgb('Vsource.SA03008H.20180718.000039')=(65280,55296,0)\nX ModifyGraph rgb('Lockin0.SA03008H.20180718.000039')=(57344,65280,0)\nX ModifyGraph rgb('Lockin1.SA03008H.20180718.000039')=(37376,65280,0)\nX ModifyGraph rgb('Lockin2.SA03008H.20180718.000039')=(18944,65280,0)\nX ModifyGraph rgb('Lockin3.SA03008H.20180718.000039')=(512,65280,0)\nX ModifyGraph rgb('Lockin4.SA03008H.20180718.000039')=(0,65280,17920)\nX ModifyGraph rgb('Lockin5.SA03008H.20180718.000039')=(0,65280,36352)\nX ModifyGraph rgb('B_rate.SA03008H.20180718.000039')=(0,65280,54784)\nX ModifyGraph rgb('DC0.SA03008H.20180718.000039')=(0,57856,65280)\nX ModifyGraph rgb('DC1.SA03008H.20180718.000039')=(0,39424,65280)\nX ModifyGraph rgb('DC2.SA03008H.20180718.000039')=(0,20992,65280)\nX ModifyGraph rgb('DC3.SA03008H.20180718.000039')=(0,2560,65280)\nX ModifyGraph rgb('DC4.SA03008H.20180718.000039')=(17408,0,65280)\nX ModifyGraph rgb('DC5.SA03008H.20180718.000039')=(35840,0,65280)\nX ModifyGraph rgb('DC6.SA03008H.20180718.000039')=(54272,0,65280)\nX ModifyGraph rgb('DC7.SA03008H.20180718.000039')=(65280,0,58368)\nX Legend/C/N=text0/J \"\\\\s('time.SA03008H.20180718.000039') time\\r\\\\s('temp.SA03008H.20180718.000039') temp\\r\\\\s('B.SA03008H.20180718.000039') B\\r\\\\s('Vsource.SA03008H.20180718.000039') Vsource\\r\\\\s('Lockin0.SA03008H.20180718.000039') Lockin0\\r\\\\s('Lockin1.SA03008H.20180718.000039') Lockin1\\r\\\\s('Lockin2.SA03008H.20180718.000039') Lockin2\\r\\\\s('Lockin3.SA03008H.20180718.000039') Lockin3\\r\\\\s('Lockin4.SA03008H.20180718.000039') Lockin4\\r\\\\s('Lockin5.SA03008H.20180718.000039') Lockin5\\r\\\\s('B_rate.SA03008H.20180718.000039') B_rate\\r\\\\s('DC0.SA03008H.20180718.000039') DC0\\r\\\\s('DC1.SA03008H.20180718.000039') DC1\\r\\\\s('DC2.SA03008H.20180718.000039') DC2\\r\\\\s('DC3.SA03008H.20180718.000039') DC3\\r\\\\s('DC4.SA03008H.20180718.000039') DC4\\r\\\\s('DC5.SA03008H.20180718.000039') DC5\\r\\\\s('DC6.SA03008H.20180718.000039') DC6\\r\\\\s('DC7.SA03008H.20180718.000039') DC7\"\nX ModifyGraph mirror(bottom)=1\nX ModifyGraph width=216\nX ModifyGraph height={Aspect,0.6}\nX ModifyGraph Log(bottom)=0\nX ModifyGraph Log(left)=0\nX \n", "IGOR\nX// Date: 7/18/2018 5:26 PM\nX// SA03008H\nX// \nX// Source 2 Drain 28 (lockin 1 and 7)\nX// Slow sweeping BG -5 to 5 inc. 0.1V \nX// Fast sweep SG -1 to 1 inc. 0.05V\n\nX// DSA_Vsg1=1.000000\n\nX// \nX// B= 0.000000\n\n\n\n\n\n\n\n\n\n\n\n\n\n\n\n\n\n\n\n\n\n\n\n\n\n\n\n\n\n\n\n\n\n\n\n\n\n\n\n\nX \nX Display/R 'time.SA03008H.20180718.000040'\nX AppendToGraph 'temp.SA03008H.20180718.000040'\nX AppendToGraph 'B.SA03008H.20180718.000040'\nX AppendToGraph 'Vsource.SA03008H.20180718.000040'\nX AppendToGraph 'Lockin0.SA03008H.20180718.000040'\nX AppendToGraph 'Lockin1.SA03008H.20180718.000040'\nX AppendToGraph 'Lockin2.SA03008H.20180718.000040'\nX AppendToGraph 'Lockin3.SA03008H.20180718.000040'\nX AppendToGraph 'Lockin4.SA03008H.20180718.000040'\nX AppendToGraph 'Lockin5.SA03008H.20180718.000040'\nX AppendToGraph 'B_rate.SA03008H.20180718.000040'\nX AppendToGraph 'DC0.SA03008H.20180718.000040'\nX AppendToGraph 'DC1.SA03008H.20180718.000040'\nX AppendToGraph 'DC2.SA03008H.20180718.000040'\nX AppendToGraph 'DC3.SA03008H.20180718.000040'\nX AppendToGraph 'DC4.SA03008H.20180718.000040'\nX AppendToGraph 'DC5.SA03008H.20180718.000040'\nX AppendToGraph 'DC6.SA03008H.20180718.000040'\nX AppendToGraph 'DC7.SA03008H.20180718.000040'\nX Label bottom \"x label\"\nX Label left \"y label\"\nX ModifyGraph rgb('time.SA03008H.20180718.000040')=(65280,0,0)\nX ModifyGraph rgb('temp.SA03008H.20180718.000040')=(65280,18432,0)\nX ModifyGraph rgb('B.SA03008H.20180718.000040')=(65280,36864,0)\nX ModifyGraph rgb('Vsource.SA03008H.20180718.000040')=(65280,55296,0)\nX ModifyGraph rgb('Lockin0.SA03008H.20180718.000040')=(57344,65280,0)\nX ModifyGraph rgb('Lockin1.SA03008H.20180718.000040')=(37376,65280,0)\nX ModifyGraph rgb('Lockin2.SA03008H.20180718.000040')=(18944,65280,0)\nX ModifyGraph rgb('Lockin3.SA03008H.20180718.000040')=(512,65280,0)\nX ModifyGraph rgb('Lockin4.SA03008H.20180718.000040')=(0,65280,17920)\nX ModifyGraph rgb('Lockin5.SA03008H.20180718.000040')=(0,65280,36352)\nX ModifyGraph rgb('B_rate.SA03008H.20180718.000040')=(0,65280,54784)\nX ModifyGraph rgb('DC0.SA03008H.20180718.000040')=(0,57856,65280)\nX ModifyGraph rgb('DC1.SA03008H.20180718.000040')=(0,39424,65280)\nX ModifyGraph rgb('DC2.SA03008H.20180718.000040')=(0,20992,65280)\nX ModifyGraph rgb('DC3.SA03008H.20180718.000040')=(0,2560,65280)\nX ModifyGraph rgb('DC4.SA03008H.20180718.000040')=(17408,0,65280)\nX ModifyGraph rgb('DC5.SA03008H.20180718.000040')=(35840,0,65280)\nX ModifyGraph rgb('DC6.SA03008H.20180718.000040')=(54272,0,65280)\nX ModifyGraph rgb('DC7.SA03008H.20180718.000040')=(65280,0,58368)\nX Legend/C/N=text0/J \"\\\\s('time.SA03008H.20180718.000040') time\\r\\\\s('temp.SA03008H.20180718.000040') temp\\r\\\\s('B.SA03008H.20180718.000040') B\\r\\\\s('Vsource.SA03008H.20180718.000040') Vsource\\r\\\\s('Lockin0.SA03008H.20180718.000040') Lockin0\\r\\\\s('Lockin1.SA03008H.20180718.000040') Lockin1\\r\\\\s('Lockin2.SA03008H.20180718.000040') Lockin2\\r\\\\s('Lockin3.SA03008H.20180718.000040') Lockin3\\r\\\\s('Lockin4.SA03008H.20180718.000040') Lockin4\\r\\\\s('Lockin5.SA03008H.20180718.000040') Lockin5\\r\\\\s('B_rate.SA03008H.20180718.000040') B_rate\\r\\\\s('DC0.SA03008H.20180718.000040') DC0\\r\\\\s('DC1.SA03008H.20180718.000040') DC1\\r\\\\s('DC2.SA03008H.20180718.000040') DC2\\r\\\\s('DC3.SA03008H.20180718.000040') DC3\\r\\\\s('DC4.SA03008H.20180718.000040') DC4\\r\\\\s('DC5.SA03008H.20180718.000040') DC5\\r\\\\s('DC6.SA03008H.20180718.000040') DC6\\r\\\\s('DC7.SA03008H.20180718.000040') DC7\"\nX ModifyGraph mirror(bottom)=1\nX ModifyGraph width=216\nX ModifyGraph height={Aspect,0.6}\nX ModifyGraph Log(bottom)=0\nX ModifyGraph Log(left)=0\nX \n", "IGOR\nX// Date: 7/18/2018 5:26 PM\nX// SA03008H\nX// \nX// Source 2 Drain 28 (lockin 1 and 7)\nX// Slow sweeping BG -5 to 5 inc. 0.1V \nX// Fast sweep SG -1 to 1 inc. 0.05V\n\nX// DSA_Vsg1=-1.000000\n\nX// \nX// B= 0.000000\n\n\n\n\n\n\n\n\n\n\n\n\n\n\n\n\n\n\n\n\n\n\n\n\n\n\n\n\n\n\n\n\n\n\n\n\n\n\n\n\nX \nX Display/R 'time.SA03008H.20180718.000041'\nX AppendToGraph 'temp.SA03008H.20180718.000041'\nX AppendToGraph 'B.SA03008H.20180718.000041'\nX AppendToGraph 'Vsource.SA03008H.20180718.000041'\nX AppendToGraph 'Lockin0.SA03008H.20180718.000041'\nX AppendToGraph 'Lockin1.SA03008H.20180718.000041'\nX AppendToGraph 'Lockin2.SA03008H.20180718.000041'\nX AppendToGraph 'Lockin3.SA03008H.20180718.000041'\nX AppendToGraph 'Lockin4.SA03008H.20180718.000041'\nX AppendToGraph 'Lockin5.SA03008H.20180718.000041'\nX AppendToGraph 'B_rate.SA03008H.20180718.000041'\nX AppendToGraph 'DC0.SA03008H.20180718.000041'\nX AppendToGraph 'DC1.SA03008H.20180718.000041'\nX AppendToGraph 'DC2.SA03008H.20180718.000041'\nX AppendToGraph 'DC3.SA03008H.20180718.000041'\nX AppendToGraph 'DC4.SA03008H.20180718.000041'\nX AppendToGraph 'DC5.SA03008H.20180718.000041'\nX AppendToGraph 'DC6.SA03008H.20180718.000041'\nX AppendToGraph 'DC7.SA03008H.20180718.000041'\nX Label bottom \"x label\"\nX Label left \"y label\"\nX ModifyGraph rgb('time.SA03008H.20180718.000041')=(65280,0,0)\nX ModifyGraph rgb('temp.SA03008H.20180718.000041')=(65280,18432,0)\nX ModifyGraph rgb('B.SA03008H.20180718.000041')=(65280,36864,0)\nX ModifyGraph rgb('Vsource.SA03008H.20180718.000041')=(65280,55296,0)\nX ModifyGraph rgb('Lockin0.SA03008H.20180718.000041')=(57344,65280,0)\nX ModifyGraph rgb('Lockin1.SA03008H.20180718.000041')=(37376,65280,0)\nX ModifyGraph rgb('Lockin2.SA03008H.20180718.000041')=(18944,65280,0)\nX ModifyGraph rgb('Lockin3.SA03008H.20180718.000041')=(512,65280,0)\nX ModifyGraph rgb('Lockin4.SA03008H.20180718.000041')=(0,65280,17920)\nX ModifyGraph rgb('Lockin5.SA03008H.20180718.000041')=(0,65280,36352)\nX ModifyGraph rgb('B_rate.SA03008H.20180718.000041')=(0,65280,54784)\nX ModifyGraph rgb('DC0.SA03008H.20180718.000041')=(0,57856,65280)\nX ModifyGraph rgb('DC1.SA03008H.20180718.000041')=(0,39424,65280)\nX ModifyGraph rgb('DC2.SA03008H.20180718.000041')=(0,20992,65280)\nX ModifyGraph rgb('DC3.SA03008H.20180718.000041')=(0,2560,65280)\nX ModifyGraph rgb('DC4.SA03008H.20180718.000041')=(17408,0,65280)\nX ModifyGraph rgb('DC5.SA03008H.20180718.000041')=(35840,0,65280)\nX ModifyGraph rgb('DC6.SA03008H.20180718.000041')=(54272,0,65280)\nX ModifyGraph rgb('DC7.SA03008H.20180718.000041')=(65280,0,58368)\nX Legend/C/N=text0/J \"\\\\s('time.SA03008H.20180718.000041') time\\r\\\\s('temp.SA03008H.20180718.000041') temp\\r\\\\s('B.SA03008H.20180718.000041') B\\r\\\\s('Vsource.SA03008H.20180718.000041') Vsource\\r\\\\s('Lockin0.SA03008H.20180718.000041') Lockin0\\r\\\\s('Lockin1.SA03008H.20180718.000041') Lockin1\\r\\\\s('Lockin2.SA03008H.20180718.000041') Lockin2\\r\\\\s('Lockin3.SA03008H.20180718.000041') Lockin3\\r\\\\s('Lockin4.SA03008H.20180718.000041') Lockin4\\r\\\\s('Lockin5.SA03008H.20180718.000041') Lockin5\\r\\\\s('B_rate.SA03008H.20180718.000041') B_rate\\r\\\\s('DC0.SA03008H.20180718.000041') DC0\\r\\\\s('DC1.SA03008H.20180718.000041') DC1\\r\\\\s('DC2.SA03008H.20180718.000041') DC2\\r\\\\s('DC3.SA03008H.20180718.000041') DC3\\r\\\\s('DC4.SA03008H.20180718.000041') DC4\\r\\\\s('DC5.SA03008H.20180718.000041') DC5\\r\\\\s('DC6.SA03008H.20180718.000041') DC6\\r\\\\s('DC7.SA03008H.20180718.000041') DC7\"\nX ModifyGraph mirror(bottom)=1\nX ModifyGraph width=216\nX ModifyGraph height={Aspect,0.6}\nX ModifyGraph Log(bottom)=0\nX ModifyGraph Log(left)=0\nX \n", "IGOR\nX// Date: 7/18/2018 5:27 PM\nX// SA03008H\nX// \nX// Source 2 Drain 28 (lockin 1 and 7)\nX// Slow sweeping BG -5 to 5 inc. 0.1V \nX// Fast sweep SG -1 to 1 inc. 0.05V\n\nX// DSA_Vsg1=-0.950000\n\nX// \nX// B= 0.000000\n\n\n\n\n\n\n\n\n\n\n\n\n\n\n\n\n\n\n\n\n\n\n\n\n\n\n\n\n\n\n\n\n\n\n\n\n\n\n\n\nX \nX Display/R 'time.SA03008H.20180718.000042'\nX AppendToGraph 'temp.SA03008H.20180718.000042'\nX AppendToGraph 'B.SA03008H.20180718.000042'\nX AppendToGraph 'Vsource.SA03008H.20180718.000042'\nX AppendToGraph 'Lockin0.SA03008H.20180718.000042'\nX AppendToGraph 'Lockin1.SA03008H.20180718.000042'\nX AppendToGraph 'Lockin2.SA03008H.20180718.000042'\nX AppendToGraph 'Lockin3.SA03008H.20180718.000042'\nX AppendToGraph 'Lockin4.SA03008H.20180718.000042'\nX AppendToGraph 'Lockin5.SA03008H.20180718.000042'\nX AppendToGraph 'B_rate.SA03008H.20180718.000042'\nX AppendToGraph 'DC0.SA03008H.20180718.000042'\nX AppendToGraph 'DC1.SA03008H.20180718.000042'\nX AppendToGraph 'DC2.SA03008H.20180718.000042'\nX AppendToGraph 'DC3.SA03008H.20180718.000042'\nX AppendToGraph 'DC4.SA03008H.20180718.000042'\nX AppendToGraph 'DC5.SA03008H.20180718.000042'\nX AppendToGraph 'DC6.SA03008H.20180718.000042'\nX AppendToGraph 'DC7.SA03008H.20180718.000042'\nX Label bottom \"x label\"\nX Label left \"y label\"\nX ModifyGraph rgb('time.SA03008H.20180718.000042')=(65280,0,0)\nX ModifyGraph rgb('temp.SA03008H.20180718.000042')=(65280,18432,0)\nX ModifyGraph rgb('B.SA03008H.20180718.000042')=(65280,36864,0)\nX ModifyGraph rgb('Vsource.SA03008H.20180718.000042')=(65280,55296,0)\nX ModifyGraph rgb('Lockin0.SA03008H.20180718.000042')=(57344,65280,0)\nX ModifyGraph rgb('Lockin1.SA03008H.20180718.000042')=(37376,65280,0)\nX ModifyGraph rgb('Lockin2.SA03008H.20180718.000042')=(18944,65280,0)\nX ModifyGraph rgb('Lockin3.SA03008H.20180718.000042')=(512,65280,0)\nX ModifyGraph rgb('Lockin4.SA03008H.20180718.000042')=(0,65280,17920)\nX ModifyGraph rgb('Lockin5.SA03008H.20180718.000042')=(0,65280,36352)\nX ModifyGraph rgb('B_rate.SA03008H.20180718.000042')=(0,65280,54784)\nX ModifyGraph rgb('DC0.SA03008H.20180718.000042')=(0,57856,65280)\nX ModifyGraph rgb('DC1.SA03008H.20180718.000042')=(0,39424,65280)\nX ModifyGraph rgb('DC2.SA03008H.20180718.000042')=(0,20992,65280)\nX ModifyGraph rgb('DC3.SA03008H.20180718.000042')=(0,2560,65280)\nX ModifyGraph rgb('DC4.SA03008H.20180718.000042')=(17408,0,65280)\nX ModifyGraph rgb('DC5.SA03008H.20180718.000042')=(35840,0,65280)\nX ModifyGraph rgb('DC6.SA03008H.20180718.000042')=(54272,0,65280)\nX ModifyGraph rgb('DC7.SA03008H.20180718.000042')=(65280,0,58368)\nX Legend/C/N=text0/J \"\\\\s('time.SA03008H.20180718.000042') time\\r\\\\s('temp.SA03008H.20180718.000042') temp\\r\\\\s('B.SA03008H.20180718.000042') B\\r\\\\s('Vsource.SA03008H.20180718.000042') Vsource\\r\\\\s('Lockin0.SA03008H.20180718.000042') Lockin0\\r\\\\s('Lockin1.SA03008H.20180718.000042') Lockin1\\r\\\\s('Lockin2.SA03008H.20180718.000042') Lockin2\\r\\\\s('Lockin3.SA03008H.20180718.000042') Lockin3\\r\\\\s('Lockin4.SA03008H.20180718.000042') Lockin4\\r\\\\s('Lockin5.SA03008H.20180718.000042') Lockin5\\r\\\\s('B_rate.SA03008H.20180718.000042') B_rate\\r\\\\s('DC0.SA03008H.20180718.000042') DC0\\r\\\\s('DC1.SA03008H.20180718.000042') DC1\\r\\\\s('DC2.SA03008H.20180718.000042') DC2\\r\\\\s('DC3.SA03008H.20180718.000042') DC3\\r\\\\s('DC4.SA03008H.20180718.000042') DC4\\r\\\\s('DC5.SA03008H.20180718.000042') DC5\\r\\\\s('DC6.SA03008H.20180718.000042') DC6\\r\\\\s('DC7.SA03008H.20180718.000042') DC7\"\nX ModifyGraph mirror(bottom)=1\nX ModifyGraph width=216\nX ModifyGraph height={Aspect,0.6}\nX ModifyGraph Log(bottom)=0\nX ModifyGraph Log(left)=0\nX \n", "IGOR\nX// Date: 7/18/2018 5:27 PM\nX// SA03008H\nX// \nX// Source 2 Drain 28 (lockin 1 and 7)\nX// Slow sweeping BG -5 to 5 inc. 0.1V \nX// Fast sweep SG -1 to 1 inc. 0.05V\n\nX// DSA_Vsg1=-0.900000\n\nX// \nX// B= 0.000000\n\n\n\n\n\n\n\n\n\n\n\n\n\n\n\n\n\n\n\n\n\n\n\n\n\n\n\n\n\n\n\n\n\n\n\n\n\n\n\n\nX \nX Display/R 'time.SA03008H.20180718.000043'\nX AppendToGraph 'temp.SA03008H.20180718.000043'\nX AppendToGraph 'B.SA03008H.20180718.000043'\nX AppendToGraph 'Vsource.SA03008H.20180718.000043'\nX AppendToGraph 'Lockin0.SA03008H.20180718.000043'\nX AppendToGraph 'Lockin1.SA03008H.20180718.000043'\nX AppendToGraph 'Lockin2.SA03008H.20180718.000043'\nX AppendToGraph 'Lockin3.SA03008H.20180718.000043'\nX AppendToGraph 'Lockin4.SA03008H.20180718.000043'\nX AppendToGraph 'Lockin5.SA03008H.20180718.000043'\nX AppendToGraph 'B_rate.SA03008H.20180718.000043'\nX AppendToGraph 'DC0.SA03008H.20180718.000043'\nX AppendToGraph 'DC1.SA03008H.20180718.000043'\nX AppendToGraph 'DC2.SA03008H.20180718.000043'\nX AppendToGraph 'DC3.SA03008H.20180718.000043'\nX AppendToGraph 'DC4.SA03008H.20180718.000043'\nX AppendToGraph 'DC5.SA03008H.20180718.000043'\nX AppendToGraph 'DC6.SA03008H.20180718.000043'\nX AppendToGraph 'DC7.SA03008H.20180718.000043'\nX Label bottom \"x label\"\nX Label left \"y label\"\nX ModifyGraph rgb('time.SA03008H.20180718.000043')=(65280,0,0)\nX ModifyGraph rgb('temp.SA03008H.20180718.000043')=(65280,18432,0)\nX ModifyGraph rgb('B.SA03008H.20180718.000043')=(65280,36864,0)\nX ModifyGraph rgb('Vsource.SA03008H.20180718.000043')=(65280,55296,0)\nX ModifyGraph rgb('Lockin0.SA03008H.20180718.000043')=(57344,65280,0)\nX ModifyGraph rgb('Lockin1.SA03008H.20180718.000043')=(37376,65280,0)\nX ModifyGraph rgb('Lockin2.SA03008H.20180718.000043')=(18944,65280,0)\nX ModifyGraph rgb('Lockin3.SA03008H.20180718.000043')=(512,65280,0)\nX ModifyGraph rgb('Lockin4.SA03008H.20180718.000043')=(0,65280,17920)\nX ModifyGraph rgb('Lockin5.SA03008H.20180718.000043')=(0,65280,36352)\nX ModifyGraph rgb('B_rate.SA03008H.20180718.000043')=(0,65280,54784)\nX ModifyGraph rgb('DC0.SA03008H.20180718.000043')=(0,57856,65280)\nX ModifyGraph rgb('DC1.SA03008H.20180718.000043')=(0,39424,65280)\nX ModifyGraph rgb('DC2.SA03008H.20180718.000043')=(0,20992,65280)\nX ModifyGraph rgb('DC3.SA03008H.20180718.000043')=(0,2560,65280)\nX ModifyGraph rgb('DC4.SA03008H.20180718.000043')=(17408,0,65280)\nX ModifyGraph rgb('DC5.SA03008H.20180718.000043')=(35840,0,65280)\nX ModifyGraph rgb('DC6.SA03008H.20180718.000043')=(54272,0,65280)\nX ModifyGraph rgb('DC7.SA03008H.20180718.000043')=(65280,0,58368)\nX Legend/C/N=text0/J \"\\\\s('time.SA03008H.20180718.000043') time\\r\\\\s('temp.SA03008H.20180718.000043') temp\\r\\\\s('B.SA03008H.20180718.000043') B\\r\\\\s('Vsource.SA03008H.20180718.000043') Vsource\\r\\\\s('Lockin0.SA03008H.20180718.000043') Lockin0\\r\\\\s('Lockin1.SA03008H.20180718.000043') Lockin1\\r\\\\s('Lockin2.SA03008H.20180718.000043') Lockin2\\r\\\\s('Lockin3.SA03008H.20180718.000043') Lockin3\\r\\\\s('Lockin4.SA03008H.20180718.000043') Lockin4\\r\\\\s('Lockin5.SA03008H.20180718.000043') Lockin5\\r\\\\s('B_rate.SA03008H.20180718.000043') B_rate\\r\\\\s('DC0.SA03008H.20180718.000043') DC0\\r\\\\s('DC1.SA03008H.20180718.000043') DC1\\r\\\\s('DC2.SA03008H.20180718.000043') DC2\\r\\\\s('DC3.SA03008H.20180718.000043') DC3\\r\\\\s('DC4.SA03008H.20180718.000043') DC4\\r\\\\s('DC5.SA03008H.20180718.000043') DC5\\r\\\\s('DC6.SA03008H.20180718.000043') DC6\\r\\\\s('DC7.SA03008H.20180718.000043') DC7\"\nX ModifyGraph mirror(bottom)=1\nX ModifyGraph width=216\nX ModifyGraph height={Aspect,0.6}\nX ModifyGraph Log(bottom)=0\nX ModifyGraph Log(left)=0\nX \n", "IGOR\nX// Date: 7/18/2018 5:27 PM\nX// SA03008H\nX// \nX// Source 2 Drain 28 (lockin 1 and 7)\nX// Slow sweeping BG -5 to 5 inc. 0.1V \nX// Fast sweep SG -1 to 1 inc. 0.05V\n\nX// DSA_Vsg1=-0.850000\n\nX// \nX// B= 0.000000\n\n\n\n\n\n\n\n\n\n\n\n\n\n\n\n\n\n\n\n\n\n\n\n\n\n\n\n\n\n\n\n\n\n\n\n\n\n\n\n\nX \nX Display/R 'time.SA03008H.20180718.000044'\nX AppendToGraph 'temp.SA03008H.20180718.000044'\nX AppendToGraph 'B.SA03008H.20180718.000044'\nX AppendToGraph 'Vsource.SA03008H.20180718.000044'\nX AppendToGraph 'Lockin0.SA03008H.20180718.000044'\nX AppendToGraph 'Lockin1.SA03008H.20180718.000044'\nX AppendToGraph 'Lockin2.SA03008H.20180718.000044'\nX AppendToGraph 'Lockin3.SA03008H.20180718.000044'\nX AppendToGraph 'Lockin4.SA03008H.20180718.000044'\nX AppendToGraph 'Lockin5.SA03008H.20180718.000044'\nX AppendToGraph 'B_rate.SA03008H.20180718.000044'\nX AppendToGraph 'DC0.SA03008H.20180718.000044'\nX AppendToGraph 'DC1.SA03008H.20180718.000044'\nX AppendToGraph 'DC2.SA03008H.20180718.000044'\nX AppendToGraph 'DC3.SA03008H.20180718.000044'\nX AppendToGraph 'DC4.SA03008H.20180718.000044'\nX AppendToGraph 'DC5.SA03008H.20180718.000044'\nX AppendToGraph 'DC6.SA03008H.20180718.000044'\nX AppendToGraph 'DC7.SA03008H.20180718.000044'\nX Label bottom \"x label\"\nX Label left \"y label\"\nX ModifyGraph rgb('time.SA03008H.20180718.000044')=(65280,0,0)\nX ModifyGraph rgb('temp.SA03008H.20180718.000044')=(65280,18432,0)\nX ModifyGraph rgb('B.SA03008H.20180718.000044')=(65280,36864,0)\nX ModifyGraph rgb('Vsource.SA03008H.20180718.000044')=(65280,55296,0)\nX ModifyGraph rgb('Lockin0.SA03008H.20180718.000044')=(57344,65280,0)\nX ModifyGraph rgb('Lockin1.SA03008H.20180718.000044')=(37376,65280,0)\nX ModifyGraph rgb('Lockin2.SA03008H.20180718.000044')=(18944,65280,0)\nX ModifyGraph rgb('Lockin3.SA03008H.20180718.000044')=(512,65280,0)\nX ModifyGraph rgb('Lockin4.SA03008H.20180718.000044')=(0,65280,17920)\nX ModifyGraph rgb('Lockin5.SA03008H.20180718.000044')=(0,65280,36352)\nX ModifyGraph rgb('B_rate.SA03008H.20180718.000044')=(0,65280,54784)\nX ModifyGraph rgb('DC0.SA03008H.20180718.000044')=(0,57856,65280)\nX ModifyGraph rgb('DC1.SA03008H.20180718.000044')=(0,39424,65280)\nX ModifyGraph rgb('DC2.SA03008H.20180718.000044')=(0,20992,65280)\nX ModifyGraph rgb('DC3.SA03008H.20180718.000044')=(0,2560,65280)\nX ModifyGraph rgb('DC4.SA03008H.20180718.000044')=(17408,0,65280)\nX ModifyGraph rgb('DC5.SA03008H.20180718.000044')=(35840,0,65280)\nX ModifyGraph rgb('DC6.SA03008H.20180718.000044')=(54272,0,65280)\nX ModifyGraph rgb('DC7.SA03008H.20180718.000044')=(65280,0,58368)\nX Legend/C/N=text0/J \"\\\\s('time.SA03008H.20180718.000044') time\\r\\\\s('temp.SA03008H.20180718.000044') temp\\r\\\\s('B.SA03008H.20180718.000044') B\\r\\\\s('Vsource.SA03008H.20180718.000044') Vsource\\r\\\\s('Lockin0.SA03008H.20180718.000044') Lockin0\\r\\\\s('Lockin1.SA03008H.20180718.000044') Lockin1\\r\\\\s('Lockin2.SA03008H.20180718.000044') Lockin2\\r\\\\s('Lockin3.SA03008H.20180718.000044') Lockin3\\r\\\\s('Lockin4.SA03008H.20180718.000044') Lockin4\\r\\\\s('Lockin5.SA03008H.20180718.000044') Lockin5\\r\\\\s('B_rate.SA03008H.20180718.000044') B_rate\\r\\\\s('DC0.SA03008H.20180718.000044') DC0\\r\\\\s('DC1.SA03008H.20180718.000044') DC1\\r\\\\s('DC2.SA03008H.20180718.000044') DC2\\r\\\\s('DC3.SA03008H.20180718.000044') DC3\\r\\\\s('DC4.SA03008H.20180718.000044') DC4\\r\\\\s('DC5.SA03008H.20180718.000044') DC5\\r\\\\s('DC6.SA03008H.20180718.000044') DC6\\r\\\\s('DC7.SA03008H.20180718.000044') DC7\"\nX ModifyGraph mirror(bottom)=1\nX ModifyGraph width=216\nX ModifyGraph height={Aspect,0.6}\nX ModifyGraph Log(bottom)=0\nX ModifyGraph Log(left)=0\nX \n", "IGOR\nX// Date: 7/18/2018 5:27 PM\nX// SA03008H\nX// \nX// Source 2 Drain 28 (lockin 1 and 7)\nX// Slow sweeping BG -5 to 5 inc. 0.1V \nX// Fast sweep SG -1 to 1 inc. 0.05V\n\nX// DSA_Vsg1=-0.800000\n\nX// \nX// B= 0.000000\n\n\n\n\n\n\n\n\n\n\n\n\n\n\n\n\n\n\n\n\n\n\n\n\n\n\n\n\n\n\n\n\n\n\n\n\n\n\n\n\nX \nX Display/R 'time.SA03008H.20180718.000045'\nX AppendToGraph 'temp.SA03008H.20180718.000045'\nX AppendToGraph 'B.SA03008H.20180718.000045'\nX AppendToGraph 'Vsource.SA03008H.20180718.000045'\nX AppendToGraph 'Lockin0.SA03008H.20180718.000045'\nX AppendToGraph 'Lockin1.SA03008H.20180718.000045'\nX AppendToGraph 'Lockin2.SA03008H.20180718.000045'\nX AppendToGraph 'Lockin3.SA03008H.20180718.000045'\nX AppendToGraph 'Lockin4.SA03008H.20180718.000045'\nX AppendToGraph 'Lockin5.SA03008H.20180718.000045'\nX AppendToGraph 'B_rate.SA03008H.20180718.000045'\nX AppendToGraph 'DC0.SA03008H.20180718.000045'\nX AppendToGraph 'DC1.SA03008H.20180718.000045'\nX AppendToGraph 'DC2.SA03008H.20180718.000045'\nX AppendToGraph 'DC3.SA03008H.20180718.000045'\nX AppendToGraph 'DC4.SA03008H.20180718.000045'\nX AppendToGraph 'DC5.SA03008H.20180718.000045'\nX AppendToGraph 'DC6.SA03008H.20180718.000045'\nX AppendToGraph 'DC7.SA03008H.20180718.000045'\nX Label bottom \"x label\"\nX Label left \"y label\"\nX ModifyGraph rgb('time.SA03008H.20180718.000045')=(65280,0,0)\nX ModifyGraph rgb('temp.SA03008H.20180718.000045')=(65280,18432,0)\nX ModifyGraph rgb('B.SA03008H.20180718.000045')=(65280,36864,0)\nX ModifyGraph rgb('Vsource.SA03008H.20180718.000045')=(65280,55296,0)\nX ModifyGraph rgb('Lockin0.SA03008H.20180718.000045')=(57344,65280,0)\nX ModifyGraph rgb('Lockin1.SA03008H.20180718.000045')=(37376,65280,0)\nX ModifyGraph rgb('Lockin2.SA03008H.20180718.000045')=(18944,65280,0)\nX ModifyGraph rgb('Lockin3.SA03008H.20180718.000045')=(512,65280,0)\nX ModifyGraph rgb('Lockin4.SA03008H.20180718.000045')=(0,65280,17920)\nX ModifyGraph rgb('Lockin5.SA03008H.20180718.000045')=(0,65280,36352)\nX ModifyGraph rgb('B_rate.SA03008H.20180718.000045')=(0,65280,54784)\nX ModifyGraph rgb('DC0.SA03008H.20180718.000045')=(0,57856,65280)\nX ModifyGraph rgb('DC1.SA03008H.20180718.000045')=(0,39424,65280)\nX ModifyGraph rgb('DC2.SA03008H.20180718.000045')=(0,20992,65280)\nX ModifyGraph rgb('DC3.SA03008H.20180718.000045')=(0,2560,65280)\nX ModifyGraph rgb('DC4.SA03008H.20180718.000045')=(17408,0,65280)\nX ModifyGraph rgb('DC5.SA03008H.20180718.000045')=(35840,0,65280)\nX ModifyGraph rgb('DC6.SA03008H.20180718.000045')=(54272,0,65280)\nX ModifyGraph rgb('DC7.SA03008H.20180718.000045')=(65280,0,58368)\nX Legend/C/N=text0/J \"\\\\s('time.SA03008H.20180718.000045') time\\r\\\\s('temp.SA03008H.20180718.000045') temp\\r\\\\s('B.SA03008H.20180718.000045') B\\r\\\\s('Vsource.SA03008H.20180718.000045') Vsource\\r\\\\s('Lockin0.SA03008H.20180718.000045') Lockin0\\r\\\\s('Lockin1.SA03008H.20180718.000045') Lockin1\\r\\\\s('Lockin2.SA03008H.20180718.000045') Lockin2\\r\\\\s('Lockin3.SA03008H.20180718.000045') Lockin3\\r\\\\s('Lockin4.SA03008H.20180718.000045') Lockin4\\r\\\\s('Lockin5.SA03008H.20180718.000045') Lockin5\\r\\\\s('B_rate.SA03008H.20180718.000045') B_rate\\r\\\\s('DC0.SA03008H.20180718.000045') DC0\\r\\\\s('DC1.SA03008H.20180718.000045') DC1\\r\\\\s('DC2.SA03008H.20180718.000045') DC2\\r\\\\s('DC3.SA03008H.20180718.000045') DC3\\r\\\\s('DC4.SA03008H.20180718.000045') DC4\\r\\\\s('DC5.SA03008H.20180718.000045') DC5\\r\\\\s('DC6.SA03008H.20180718.000045') DC6\\r\\\\s('DC7.SA03008H.20180718.000045') DC7\"\nX ModifyGraph mirror(bottom)=1\nX ModifyGraph width=216\nX ModifyGraph height={Aspect,0.6}\nX ModifyGraph Log(bottom)=0\nX ModifyGraph Log(left)=0\nX \n", "IGOR\nX// Date: 7/18/2018 5:27 PM\nX// SA03008H\nX// \nX// Source 2 Drain 28 (lockin 1 and 7)\nX// Slow sweeping BG -5 to 5 inc. 0.1V \nX// Fast sweep SG -1 to 1 inc. 0.05V\n\nX// DSA_Vsg1=-0.750000\n\nX// \nX// B= 0.000000\n\n\n\n\n\n\n\n\n\n\n\n\n\n\n\n\n\n\n\n\n\n\n\n\n\n\n\n\n\n\n\n\n\n\n\n\n\n\n\n\nX \nX Display/R 'time.SA03008H.20180718.000046'\nX AppendToGraph 'temp.SA03008H.20180718.000046'\nX AppendToGraph 'B.SA03008H.20180718.000046'\nX AppendToGraph 'Vsource.SA03008H.20180718.000046'\nX AppendToGraph 'Lockin0.SA03008H.20180718.000046'\nX AppendToGraph 'Lockin1.SA03008H.20180718.000046'\nX AppendToGraph 'Lockin2.SA03008H.20180718.000046'\nX AppendToGraph 'Lockin3.SA03008H.20180718.000046'\nX AppendToGraph 'Lockin4.SA03008H.20180718.000046'\nX AppendToGraph 'Lockin5.SA03008H.20180718.000046'\nX AppendToGraph 'B_rate.SA03008H.20180718.000046'\nX AppendToGraph 'DC0.SA03008H.20180718.000046'\nX AppendToGraph 'DC1.SA03008H.20180718.000046'\nX AppendToGraph 'DC2.SA03008H.20180718.000046'\nX AppendToGraph 'DC3.SA03008H.20180718.000046'\nX AppendToGraph 'DC4.SA03008H.20180718.000046'\nX AppendToGraph 'DC5.SA03008H.20180718.000046'\nX AppendToGraph 'DC6.SA03008H.20180718.000046'\nX AppendToGraph 'DC7.SA03008H.20180718.000046'\nX Label bottom \"x label\"\nX Label left \"y label\"\nX ModifyGraph rgb('time.SA03008H.20180718.000046')=(65280,0,0)\nX ModifyGraph rgb('temp.SA03008H.20180718.000046')=(65280,18432,0)\nX ModifyGraph rgb('B.SA03008H.20180718.000046')=(65280,36864,0)\nX ModifyGraph rgb('Vsource.SA03008H.20180718.000046')=(65280,55296,0)\nX ModifyGraph rgb('Lockin0.SA03008H.20180718.000046')=(57344,65280,0)\nX ModifyGraph rgb('Lockin1.SA03008H.20180718.000046')=(37376,65280,0)\nX ModifyGraph rgb('Lockin2.SA03008H.20180718.000046')=(18944,65280,0)\nX ModifyGraph rgb('Lockin3.SA03008H.20180718.000046')=(512,65280,0)\nX ModifyGraph rgb('Lockin4.SA03008H.20180718.000046')=(0,65280,17920)\nX ModifyGraph rgb('Lockin5.SA03008H.20180718.000046')=(0,65280,36352)\nX ModifyGraph rgb('B_rate.SA03008H.20180718.000046')=(0,65280,54784)\nX ModifyGraph rgb('DC0.SA03008H.20180718.000046')=(0,57856,65280)\nX ModifyGraph rgb('DC1.SA03008H.20180718.000046')=(0,39424,65280)\nX ModifyGraph rgb('DC2.SA03008H.20180718.000046')=(0,20992,65280)\nX ModifyGraph rgb('DC3.SA03008H.20180718.000046')=(0,2560,65280)\nX ModifyGraph rgb('DC4.SA03008H.20180718.000046')=(17408,0,65280)\nX ModifyGraph rgb('DC5.SA03008H.20180718.000046')=(35840,0,65280)\nX ModifyGraph rgb('DC6.SA03008H.20180718.000046')=(54272,0,65280)\nX ModifyGraph rgb('DC7.SA03008H.20180718.000046')=(65280,0,58368)\nX Legend/C/N=text0/J \"\\\\s('time.SA03008H.20180718.000046') time\\r\\\\s('temp.SA03008H.20180718.000046') temp\\r\\\\s('B.SA03008H.20180718.000046') B\\r\\\\s('Vsource.SA03008H.20180718.000046') Vsource\\r\\\\s('Lockin0.SA03008H.20180718.000046') Lockin0\\r\\\\s('Lockin1.SA03008H.20180718.000046') Lockin1\\r\\\\s('Lockin2.SA03008H.20180718.000046') Lockin2\\r\\\\s('Lockin3.SA03008H.20180718.000046') Lockin3\\r\\\\s('Lockin4.SA03008H.20180718.000046') Lockin4\\r\\\\s('Lockin5.SA03008H.20180718.000046') Lockin5\\r\\\\s('B_rate.SA03008H.20180718.000046') B_rate\\r\\\\s('DC0.SA03008H.20180718.000046') DC0\\r\\\\s('DC1.SA03008H.20180718.000046') DC1\\r\\\\s('DC2.SA03008H.20180718.000046') DC2\\r\\\\s('DC3.SA03008H.20180718.000046') DC3\\r\\\\s('DC4.SA03008H.20180718.000046') DC4\\r\\\\s('DC5.SA03008H.20180718.000046') DC5\\r\\\\s('DC6.SA03008H.20180718.000046') DC6\\r\\\\s('DC7.SA03008H.20180718.000046') DC7\"\nX ModifyGraph mirror(bottom)=1\nX ModifyGraph width=216\nX ModifyGraph height={Aspect,0.6}\nX ModifyGraph Log(bottom)=0\nX ModifyGraph Log(left)=0\nX \n", "IGOR\nX// Date: 7/18/2018 5:28 PM\nX// SA03008H\nX// \nX// Source 2 Drain 28 (lockin 1 and 7)\nX// Slow sweeping BG -5 to 5 inc. 0.1V \nX// Fast sweep SG -1 to 1 inc. 0.05V\n\nX// DSA_Vsg1=-0.700000\n\nX// \nX// B= 0.000000\n\n\n\n\n\n\n\n\n\n\n\n\n\n\n\n\n\n\n\n\n\n\n\n\n\n\n\n\n\n\n\n\n\n\n\n\n\n\n\n\nX \nX Display/R 'time.SA03008H.20180718.000047'\nX AppendToGraph 'temp.SA03008H.20180718.000047'\nX AppendToGraph 'B.SA03008H.20180718.000047'\nX AppendToGraph 'Vsource.SA03008H.20180718.000047'\nX AppendToGraph 'Lockin0.SA03008H.20180718.000047'\nX AppendToGraph 'Lockin1.SA03008H.20180718.000047'\nX AppendToGraph 'Lockin2.SA03008H.20180718.000047'\nX AppendToGraph 'Lockin3.SA03008H.20180718.000047'\nX AppendToGraph 'Lockin4.SA03008H.20180718.000047'\nX AppendToGraph 'Lockin5.SA03008H.20180718.000047'\nX AppendToGraph 'B_rate.SA03008H.20180718.000047'\nX AppendToGraph 'DC0.SA03008H.20180718.000047'\nX AppendToGraph 'DC1.SA03008H.20180718.000047'\nX AppendToGraph 'DC2.SA03008H.20180718.000047'\nX AppendToGraph 'DC3.SA03008H.20180718.000047'\nX AppendToGraph 'DC4.SA03008H.20180718.000047'\nX AppendToGraph 'DC5.SA03008H.20180718.000047'\nX AppendToGraph 'DC6.SA03008H.20180718.000047'\nX AppendToGraph 'DC7.SA03008H.20180718.000047'\nX Label bottom \"x label\"\nX Label left \"y label\"\nX ModifyGraph rgb('time.SA03008H.20180718.000047')=(65280,0,0)\nX ModifyGraph rgb('temp.SA03008H.20180718.000047')=(65280,18432,0)\nX ModifyGraph rgb('B.SA03008H.20180718.000047')=(65280,36864,0)\nX ModifyGraph rgb('Vsource.SA03008H.20180718.000047')=(65280,55296,0)\nX ModifyGraph rgb('Lockin0.SA03008H.20180718.000047')=(57344,65280,0)\nX ModifyGraph rgb('Lockin1.SA03008H.20180718.000047')=(37376,65280,0)\nX ModifyGraph rgb('Lockin2.SA03008H.20180718.000047')=(18944,65280,0)\nX ModifyGraph rgb('Lockin3.SA03008H.20180718.000047')=(512,65280,0)\nX ModifyGraph rgb('Lockin4.SA03008H.20180718.000047')=(0,65280,17920)\nX ModifyGraph rgb('Lockin5.SA03008H.20180718.000047')=(0,65280,36352)\nX ModifyGraph rgb('B_rate.SA03008H.20180718.000047')=(0,65280,54784)\nX ModifyGraph rgb('DC0.SA03008H.20180718.000047')=(0,57856,65280)\nX ModifyGraph rgb('DC1.SA03008H.20180718.000047')=(0,39424,65280)\nX ModifyGraph rgb('DC2.SA03008H.20180718.000047')=(0,20992,65280)\nX ModifyGraph rgb('DC3.SA03008H.20180718.000047')=(0,2560,65280)\nX ModifyGraph rgb('DC4.SA03008H.20180718.000047')=(17408,0,65280)\nX ModifyGraph rgb('DC5.SA03008H.20180718.000047')=(35840,0,65280)\nX ModifyGraph rgb('DC6.SA03008H.20180718.000047')=(54272,0,65280)\nX ModifyGraph rgb('DC7.SA03008H.20180718.000047')=(65280,0,58368)\nX Legend/C/N=text0/J \"\\\\s('time.SA03008H.20180718.000047') time\\r\\\\s('temp.SA03008H.20180718.000047') temp\\r\\\\s('B.SA03008H.20180718.000047') B\\r\\\\s('Vsource.SA03008H.20180718.000047') Vsource\\r\\\\s('Lockin0.SA03008H.20180718.000047') Lockin0\\r\\\\s('Lockin1.SA03008H.20180718.000047') Lockin1\\r\\\\s('Lockin2.SA03008H.20180718.000047') Lockin2\\r\\\\s('Lockin3.SA03008H.20180718.000047') Lockin3\\r\\\\s('Lockin4.SA03008H.20180718.000047') Lockin4\\r\\\\s('Lockin5.SA03008H.20180718.000047') Lockin5\\r\\\\s('B_rate.SA03008H.20180718.000047') B_rate\\r\\\\s('DC0.SA03008H.20180718.000047') DC0\\r\\\\s('DC1.SA03008H.20180718.000047') DC1\\r\\\\s('DC2.SA03008H.20180718.000047') DC2\\r\\\\s('DC3.SA03008H.20180718.000047') DC3\\r\\\\s('DC4.SA03008H.20180718.000047') DC4\\r\\\\s('DC5.SA03008H.20180718.000047') DC5\\r\\\\s('DC6.SA03008H.20180718.000047') DC6\\r\\\\s('DC7.SA03008H.20180718.000047') DC7\"\nX ModifyGraph mirror(bottom)=1\nX ModifyGraph width=216\nX ModifyGraph height={Aspect,0.6}\nX ModifyGraph Log(bottom)=0\nX ModifyGraph Log(left)=0\nX \n", "IGOR\nX// Date: 7/18/2018 5:28 PM\nX// SA03008H\nX// \nX// Source 2 Drain 28 (lockin 1 and 7)\nX// Slow sweeping BG -5 to 5 inc. 0.1V \nX// Fast sweep SG -1 to 1 inc. 0.05V\n\nX// DSA_Vsg1=-0.650000\n\nX// \nX// B= 0.000000\n\n\n\n\n\n\n\n\n\n\n\n\n\n\n\n\n\n\n\n\n\n\n\n\n\n\n\n\n\n\n\n\n\n\n\n\n\n\n\n\nX \nX Display/R 'time.SA03008H.20180718.000048'\nX AppendToGraph 'temp.SA03008H.20180718.000048'\nX AppendToGraph 'B.SA03008H.20180718.000048'\nX AppendToGraph 'Vsource.SA03008H.20180718.000048'\nX AppendToGraph 'Lockin0.SA03008H.20180718.000048'\nX AppendToGraph 'Lockin1.SA03008H.20180718.000048'\nX AppendToGraph 'Lockin2.SA03008H.20180718.000048'\nX AppendToGraph 'Lockin3.SA03008H.20180718.000048'\nX AppendToGraph 'Lockin4.SA03008H.20180718.000048'\nX AppendToGraph 'Lockin5.SA03008H.20180718.000048'\nX AppendToGraph 'B_rate.SA03008H.20180718.000048'\nX AppendToGraph 'DC0.SA03008H.20180718.000048'\nX AppendToGraph 'DC1.SA03008H.20180718.000048'\nX AppendToGraph 'DC2.SA03008H.20180718.000048'\nX AppendToGraph 'DC3.SA03008H.20180718.000048'\nX AppendToGraph 'DC4.SA03008H.20180718.000048'\nX AppendToGraph 'DC5.SA03008H.20180718.000048'\nX AppendToGraph 'DC6.SA03008H.20180718.000048'\nX AppendToGraph 'DC7.SA03008H.20180718.000048'\nX Label bottom \"x label\"\nX Label left \"y label\"\nX ModifyGraph rgb('time.SA03008H.20180718.000048')=(65280,0,0)\nX ModifyGraph rgb('temp.SA03008H.20180718.000048')=(65280,18432,0)\nX ModifyGraph rgb('B.SA03008H.20180718.000048')=(65280,36864,0)\nX ModifyGraph rgb('Vsource.SA03008H.20180718.000048')=(65280,55296,0)\nX ModifyGraph rgb('Lockin0.SA03008H.20180718.000048')=(57344,65280,0)\nX ModifyGraph rgb('Lockin1.SA03008H.20180718.000048')=(37376,65280,0)\nX ModifyGraph rgb('Lockin2.SA03008H.20180718.000048')=(18944,65280,0)\nX ModifyGraph rgb('Lockin3.SA03008H.20180718.000048')=(512,65280,0)\nX ModifyGraph rgb('Lockin4.SA03008H.20180718.000048')=(0,65280,17920)\nX ModifyGraph rgb('Lockin5.SA03008H.20180718.000048')=(0,65280,36352)\nX ModifyGraph rgb('B_rate.SA03008H.20180718.000048')=(0,65280,54784)\nX ModifyGraph rgb('DC0.SA03008H.20180718.000048')=(0,57856,65280)\nX ModifyGraph rgb('DC1.SA03008H.20180718.000048')=(0,39424,65280)\nX ModifyGraph rgb('DC2.SA03008H.20180718.000048')=(0,20992,65280)\nX ModifyGraph rgb('DC3.SA03008H.20180718.000048')=(0,2560,65280)\nX ModifyGraph rgb('DC4.SA03008H.20180718.000048')=(17408,0,65280)\nX ModifyGraph rgb('DC5.SA03008H.20180718.000048')=(35840,0,65280)\nX ModifyGraph rgb('DC6.SA03008H.20180718.000048')=(54272,0,65280)\nX ModifyGraph rgb('DC7.SA03008H.20180718.000048')=(65280,0,58368)\nX Legend/C/N=text0/J \"\\\\s('time.SA03008H.20180718.000048') time\\r\\\\s('temp.SA03008H.20180718.000048') temp\\r\\\\s('B.SA03008H.20180718.000048') B\\r\\\\s('Vsource.SA03008H.20180718.000048') Vsource\\r\\\\s('Lockin0.SA03008H.20180718.000048') Lockin0\\r\\\\s('Lockin1.SA03008H.20180718.000048') Lockin1\\r\\\\s('Lockin2.SA03008H.20180718.000048') Lockin2\\r\\\\s('Lockin3.SA03008H.20180718.000048') Lockin3\\r\\\\s('Lockin4.SA03008H.20180718.000048') Lockin4\\r\\\\s('Lockin5.SA03008H.20180718.000048') Lockin5\\r\\\\s('B_rate.SA03008H.20180718.000048') B_rate\\r\\\\s('DC0.SA03008H.20180718.000048') DC0\\r\\\\s('DC1.SA03008H.20180718.000048') DC1\\r\\\\s('DC2.SA03008H.20180718.000048') DC2\\r\\\\s('DC3.SA03008H.20180718.000048') DC3\\r\\\\s('DC4.SA03008H.20180718.000048') DC4\\r\\\\s('DC5.SA03008H.20180718.000048') DC5\\r\\\\s('DC6.SA03008H.20180718.000048') DC6\\r\\\\s('DC7.SA03008H.20180718.000048') DC7\"\nX ModifyGraph mirror(bottom)=1\nX ModifyGraph width=216\nX ModifyGraph height={Aspect,0.6}\nX ModifyGraph Log(bottom)=0\nX ModifyGraph Log(left)=0\nX \n", "IGOR\nX// Date: 7/18/2018 5:28 PM\nX// SA03008H\nX// \nX// Source 2 Drain 28 (lockin 1 and 7)\nX// Slow sweeping BG -5 to 5 inc. 0.1V \nX// Fast sweep SG -1 to 1 inc. 0.05V\n\nX// DSA_Vsg1=-0.600000\n\nX// \nX// B= 0.000000\n\n\n\n\n\n\n\n\n\n\n\n\n\n\n\n\n\n\n\n\n\n\n\n\n\n\n\n\n\n\n\n\n\n\n\n\n\n\n\n\nX \nX Display/R 'time.SA03008H.20180718.000049'\nX AppendToGraph 'temp.SA03008H.20180718.000049'\nX AppendToGraph 'B.SA03008H.20180718.000049'\nX AppendToGraph 'Vsource.SA03008H.20180718.000049'\nX AppendToGraph 'Lockin0.SA03008H.20180718.000049'\nX AppendToGraph 'Lockin1.SA03008H.20180718.000049'\nX AppendToGraph 'Lockin2.SA03008H.20180718.000049'\nX AppendToGraph 'Lockin3.SA03008H.20180718.000049'\nX AppendToGraph 'Lockin4.SA03008H.20180718.000049'\nX AppendToGraph 'Lockin5.SA03008H.20180718.000049'\nX AppendToGraph 'B_rate.SA03008H.20180718.000049'\nX AppendToGraph 'DC0.SA03008H.20180718.000049'\nX AppendToGraph 'DC1.SA03008H.20180718.000049'\nX AppendToGraph 'DC2.SA03008H.20180718.000049'\nX AppendToGraph 'DC3.SA03008H.20180718.000049'\nX AppendToGraph 'DC4.SA03008H.20180718.000049'\nX AppendToGraph 'DC5.SA03008H.20180718.000049'\nX AppendToGraph 'DC6.SA03008H.20180718.000049'\nX AppendToGraph 'DC7.SA03008H.20180718.000049'\nX Label bottom \"x label\"\nX Label left \"y label\"\nX ModifyGraph rgb('time.SA03008H.20180718.000049')=(65280,0,0)\nX ModifyGraph rgb('temp.SA03008H.20180718.000049')=(65280,18432,0)\nX ModifyGraph rgb('B.SA03008H.20180718.000049')=(65280,36864,0)\nX ModifyGraph rgb('Vsource.SA03008H.20180718.000049')=(65280,55296,0)\nX ModifyGraph rgb('Lockin0.SA03008H.20180718.000049')=(57344,65280,0)\nX ModifyGraph rgb('Lockin1.SA03008H.20180718.000049')=(37376,65280,0)\nX ModifyGraph rgb('Lockin2.SA03008H.20180718.000049')=(18944,65280,0)\nX ModifyGraph rgb('Lockin3.SA03008H.20180718.000049')=(512,65280,0)\nX ModifyGraph rgb('Lockin4.SA03008H.20180718.000049')=(0,65280,17920)\nX ModifyGraph rgb('Lockin5.SA03008H.20180718.000049')=(0,65280,36352)\nX ModifyGraph rgb('B_rate.SA03008H.20180718.000049')=(0,65280,54784)\nX ModifyGraph rgb('DC0.SA03008H.20180718.000049')=(0,57856,65280)\nX ModifyGraph rgb('DC1.SA03008H.20180718.000049')=(0,39424,65280)\nX ModifyGraph rgb('DC2.SA03008H.20180718.000049')=(0,20992,65280)\nX ModifyGraph rgb('DC3.SA03008H.20180718.000049')=(0,2560,65280)\nX ModifyGraph rgb('DC4.SA03008H.20180718.000049')=(17408,0,65280)\nX ModifyGraph rgb('DC5.SA03008H.20180718.000049')=(35840,0,65280)\nX ModifyGraph rgb('DC6.SA03008H.20180718.000049')=(54272,0,65280)\nX ModifyGraph rgb('DC7.SA03008H.20180718.000049')=(65280,0,58368)\nX Legend/C/N=text0/J \"\\\\s('time.SA03008H.20180718.000049') time\\r\\\\s('temp.SA03008H.20180718.000049') temp\\r\\\\s('B.SA03008H.20180718.000049') B\\r\\\\s('Vsource.SA03008H.20180718.000049') Vsource\\r\\\\s('Lockin0.SA03008H.20180718.000049') Lockin0\\r\\\\s('Lockin1.SA03008H.20180718.000049') Lockin1\\r\\\\s('Lockin2.SA03008H.20180718.000049') Lockin2\\r\\\\s('Lockin3.SA03008H.20180718.000049') Lockin3\\r\\\\s('Lockin4.SA03008H.20180718.000049') Lockin4\\r\\\\s('Lockin5.SA03008H.20180718.000049') Lockin5\\r\\\\s('B_rate.SA03008H.20180718.000049') B_rate\\r\\\\s('DC0.SA03008H.20180718.000049') DC0\\r\\\\s('DC1.SA03008H.20180718.000049') DC1\\r\\\\s('DC2.SA03008H.20180718.000049') DC2\\r\\\\s('DC3.SA03008H.20180718.000049') DC3\\r\\\\s('DC4.SA03008H.20180718.000049') DC4\\r\\\\s('DC5.SA03008H.20180718.000049') DC5\\r\\\\s('DC6.SA03008H.20180718.000049') DC6\\r\\\\s('DC7.SA03008H.20180718.000049') DC7\"\nX ModifyGraph mirror(bottom)=1\nX ModifyGraph width=216\nX ModifyGraph height={Aspect,0.6}\nX ModifyGraph Log(bottom)=0\nX ModifyGraph Log(left)=0\nX \n"], 13 "ITX sizes (#itx, #chan, #samp)":i32[](array[numeric]), 15 "clean names":string[](array[string]))   [LabVIEW 2016]
uses:
  <vilib>/addons/WireFlow/_WF_ProgressBar.llb/ProgressBar_WireFlow.lvclass
  <userlib>/_OpenG.lib/file/file.llb/Convert File Extension (Path)__ogtk.vi
  <userlib>/_OpenG.lib/file/file.llb/File Exists - Scalar__ogtk.vi
  <userlib>/LevyLab/LV to ITX/LVtoITX.lvclass
panel:
  out "#itx":i32
  out "error out":errorcluster
  in  "error in":errorcluster
  out "total megabyte estimate":dbl=72.479248046875
  out "WF-ProgressBar out":refnum<class "ProgressBar_WireFlow.lvclass">
  in  "Generate Folder Index File?":bool
  in  "Use Folder Index File?":bool
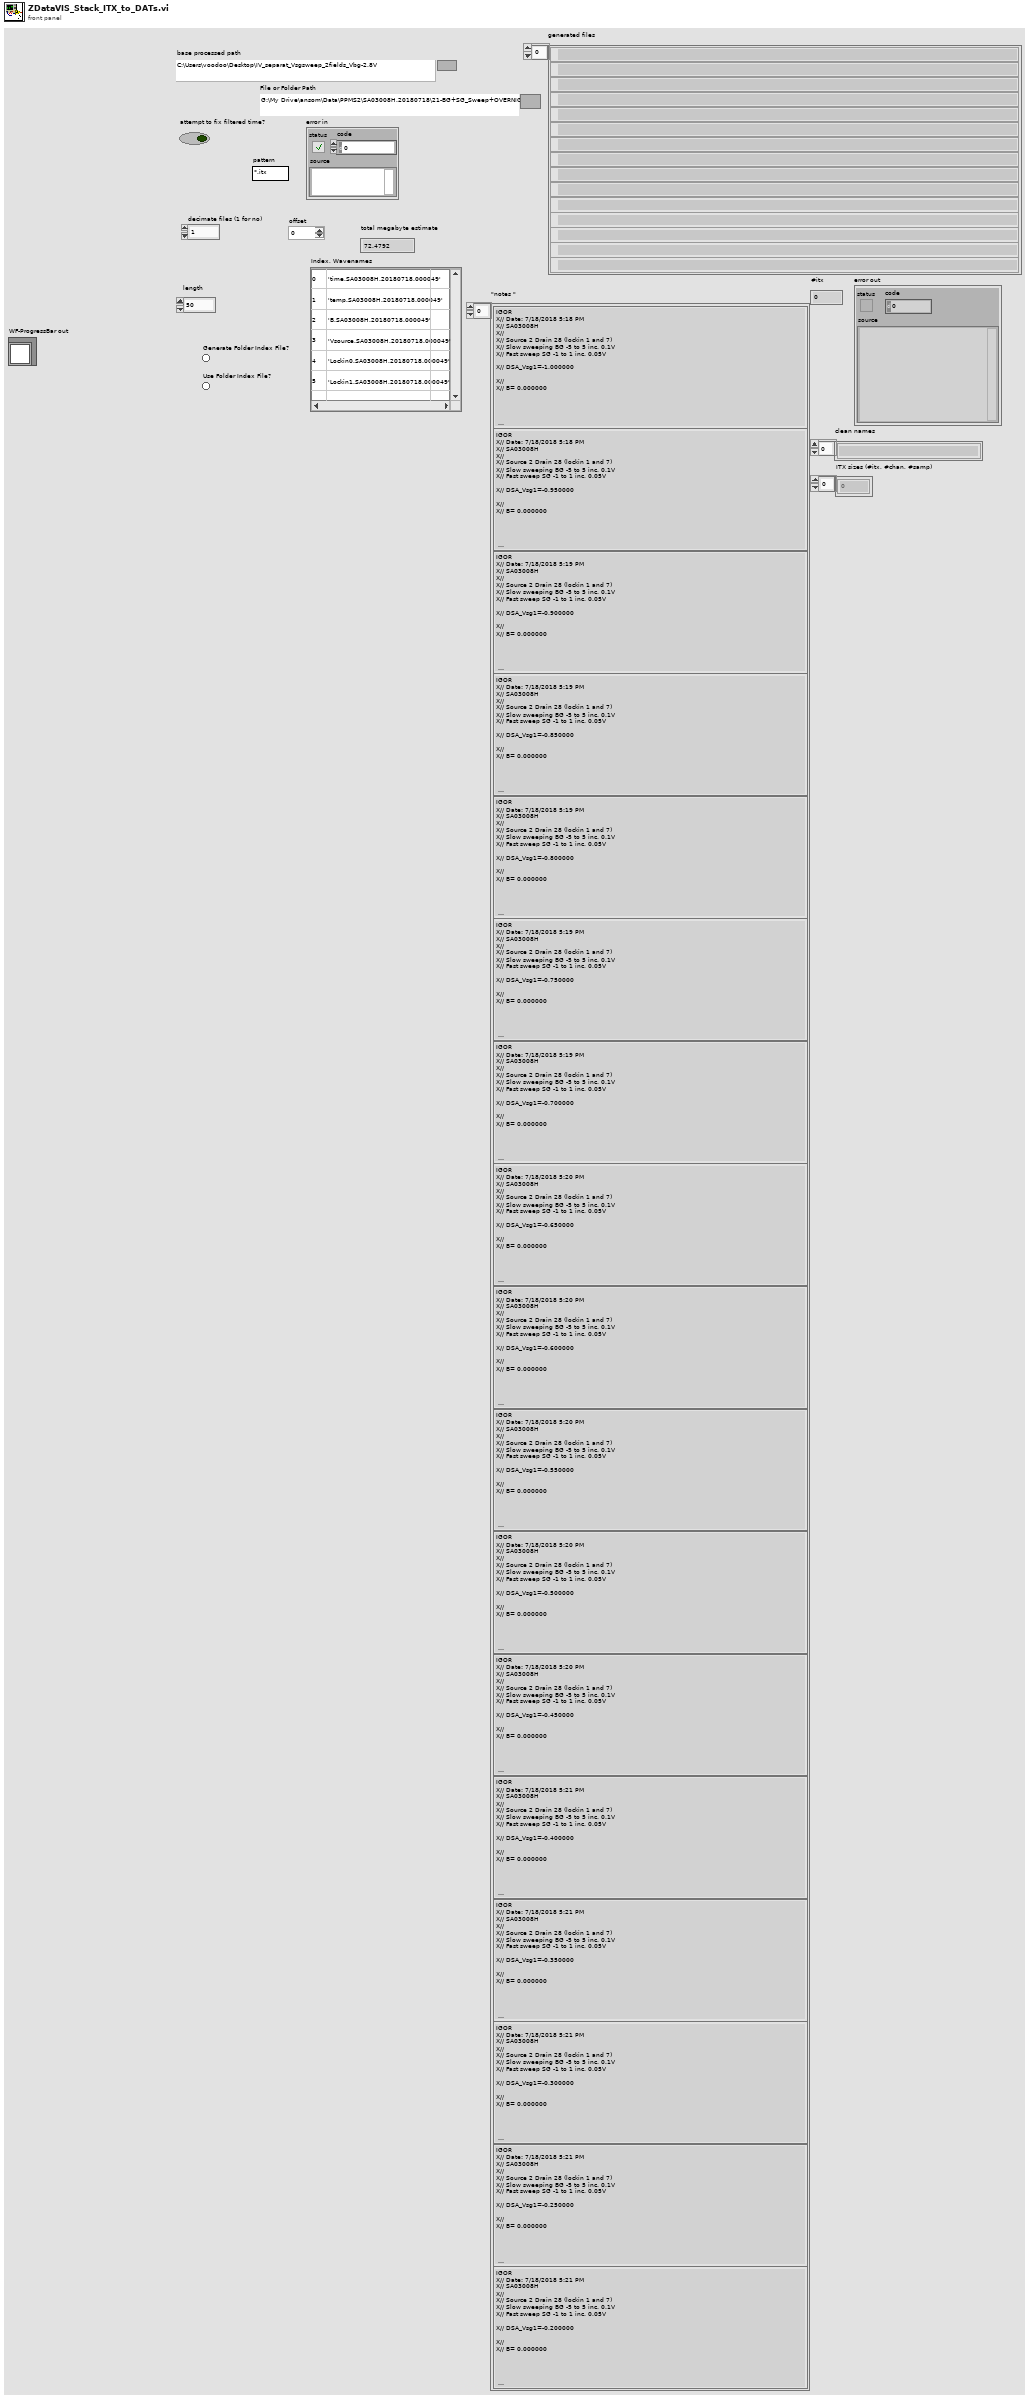
[diagram p1: front panel]
types:
  T1 = enum16{"open", "replace", "create", "open or create", "replace or create", "replace or create with confirmation"}
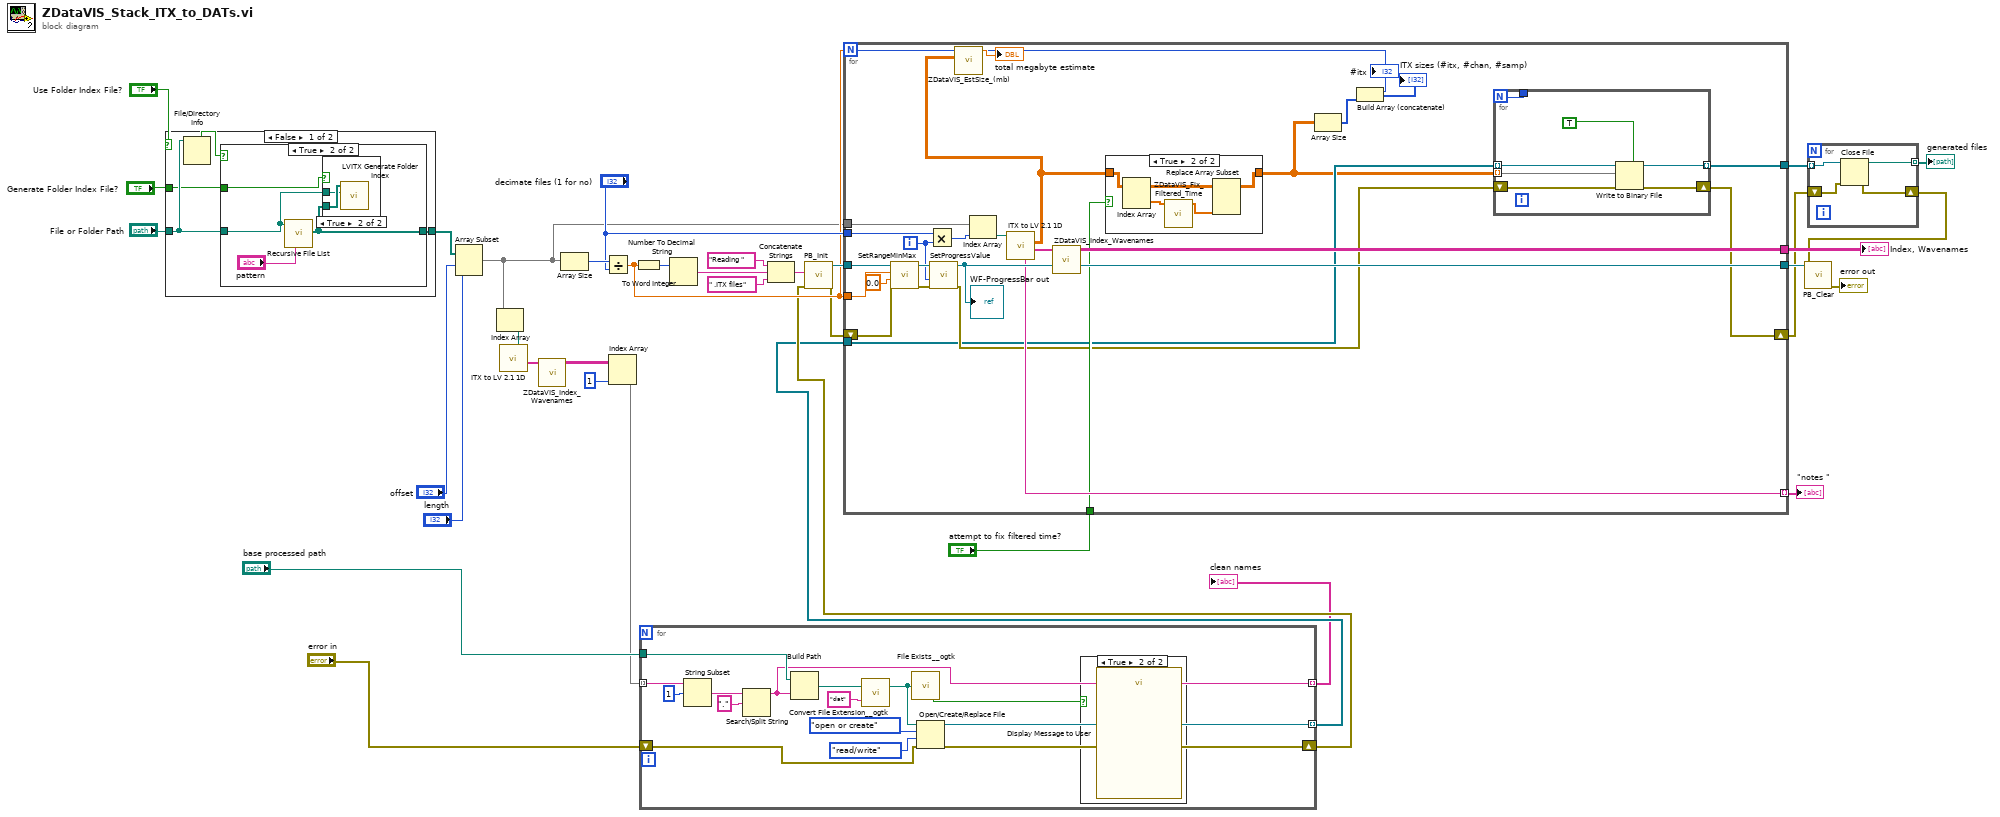
[diagram p0: block diagram]
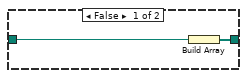
[diagram p4: hidden frame]
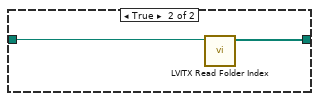
[diagram p6: hidden frame]
diagram:
  n1 = case shown="False" "Use Folder Index File?" {
    tunnel: [w38 w49] -> w31
    tunnel: "File or Folder Path" -> [w40 w50]
    tunnel: "Generate Folder Index File?" -> [w37 _]
    frame False {
      n2 = File/Directory Info(path=w40) -> (directory=w39:bool)  [unwired: 1 in, 6 out]
      n3 = case shown="True" w39 {
        tunnel: [w42 w45] -> w38
        tunnel: w40 -> [w41 w44]
        tunnel: w37 -> [_ w43]
        frame False {
          n4 = Build Array(w41) -> (w42:path[])
        }
        frame True {
          n5 = call <vilib>:"Recursive File List.vi"("pattern"="pattern", "Folder Path"=w44) -> ("All Files in Dir"=w45:path[])  [unwired: 5 in, 4 out]
          n6 = case shown="True" w43 {
            tunnel: w45 -> [_ w48]
            tunnel: w44 -> [_ w47]
            frame False {
            }
            frame True {
              n7 = call <userlib>:"LVITX Generate Folder Index.vi"("File or Folder Path"=w47, "All Files in Dir"=w48) -> ()  [unwired: 10 in]
            }
          }
        }
      }
    }
    frame True {
      n8 = call <userlib>:"LVITX Read Folder Index.vi"("File or Folder Path"=w50) -> ("Array"=w49:path[])  [unwired: 10 in]
    }
  }
  n9 = Array Subset(array=w31, index="offset", length="length") -> (w17:path[])
  n10 = Index Array(array=w17) -> (element=w16:path)  [unwired: 1 in]
  n11 = call <userlib>:"ITX to LV 2.1 1D.vi"("file (use dialog)"=w16) -> ("wave names"=w15:string[])  [unwired: 6 in, 4 out]
  n12 = call "ZDataVIS_Index_Wavenames.vi"("wave names"=w15) -> ("Index, Wavenames"=w13:string[][])  [unwired: 10 in]
  n13 = Array Size(array=w17) -> (size(s)=w32:i32)
  n14 = Divide(x=w32, y="decimate files (1 for no)") -> (x/y=w21:dbl)
  n15 = Index Array(array=w13, index (col)=1 ("disabled index (col)")) -> (element=w11:string[])  [unwired: 1 in]
  n16 = To Word Integer(number=w21) -> (16bit integer=w24:i16)
  n17 = for {
    tunnel: "base processed path" -> [w64]
    shift-right: [w54] -> w8
    shift-left: "error in" -> [w65]
    tunnel: w11 -> [w57] mode=indexing
    tunnel: [w55] -> w1 mode=indexing
    tunnel: [w53] -> w7 mode=indexing
    n18 = String Subset(string=w57, offset (0)=1) -> (substring=w56:string)  [unwired: 1 in]
    n19 = Search/Split String(string=w56, search string/char (-)=".") -> (substring before match=w55:string)  [unwired: 1 in, 2 out]
    n20 = Build Path(base path=w64, name or relative path=w55) -> (appended path=w63:path)
    n21 = call-poly <userlib>:"Convert File Extension__ogtk.vi"("new ending (none)"="dat", "file name"=w63) -> ("new filename"=w52:path)  [unwired: 1 out]
    n22 = call-poly <userlib>:"File Exists__ogtk.vi"("file path"=w52) -> ("exists"=w51:bool)  [unwired: 6 in, 1 out]
    n23 = Open/Create/Replace File(file path (use dialog)=w52, error in=w65, operation (0:open)=T1."open or create", access (0:read/write)=enum16{"read/write", "read-only", "write-only"}."read/write") -> (refnum out=w53:refnum<file>, error out=w54:errorcluster)  [unwired: 2 in, 1 out]
    n24 = case shown="True" w51 {
      frame False {
      }
      frame True {
        n25 = call "Display Message to User"() -> ()  [unwired: 10 in, 2 out]
      }
    }
  }
  "clean names" <- w1
  n26 = Number To Decimal String(number=w24) -> (decimal integer string=w23:string)  [unwired: 1 in]
  n27 = Concatenate Strings("Reading " ("title (\"Progress\")"), w23, " .ITX files" ("title (\"Progress\")")) -> (w22:string)
  n28 = call <vilib>:"PB_Init.vi"("error in (no error)"=w8, "title (\"Progress\")"=w22) -> ("error out"=w9:errorcluster, "WF-ProgressBar out"=w27:refnum<class "ProgressBar_WireFlow.lvclass">)  [unwired: 8 in]
  n29 = for {
    N: w21 -> [w68]
    tunnel: "decimate files (1 for no)" -> [w91]
    tunnel: w17 -> [w90]
    tunnel: [w86] -> w29
    tunnel: [w82] -> w28
    tunnel: w27 -> [w81]
    tunnel: w21 -> [w80]
    tunnel: [w78] -> w20 mode=indexing
    tunnel: "attempt to fix filtered time?" -> [w76]
    shift-right: [w73] -> w4
    shift-left: w9 -> [w74]
    tunnel: w7 -> [w71]
    tunnel: [w70] -> w5
    i -> [w79]
    n30 = call-dynamic "SetRangeMinMax.vi"("error in (no error)"=w74, "Min (0)"=0.0, "Max (1)"=w80, "WF-ProgressBar in"=w81) -> ("error out"=w84:errorcluster, "WF-ProgressBar out"=w83:refnum<class "ProgressBar_WireFlow.lvclass">)  [unwired: 6 in]
    n31 = Multiply(x=w91, y=w79) -> (x*y=w87:i32)
    n32 = call-dynamic "SetProgressValue.vi"("error in (no error)"=w84, "Value"=w79, "WF-ProgressBar in"=w83) -> ("error out"=w72:errorcluster, "WF-ProgressBar out"=w82:refnum<class "ProgressBar_WireFlow.lvclass">)  [unwired: 6 in, 1 out]
    "WF-ProgressBar out" <- w82
    n33 = Index Array(array=w90, index=w87) -> (element=w88:path)
    n34 = call <userlib>:"ITX to LV 2.1 1D.vi"("file (use dialog)"=w88) -> ("wave names"=w89:string[], "1D arrays"=w75:dbl[][], "Notes"=w78:string)  [unwired: 6 in, 2 out]
    n35 = call "ZDataVIS_EstSize_(mb).vi"("1D arrays"=w75, "Numeric"=w68) -> ("total megabyte estimate"=→"total megabyte estimate":dbl)  [unwired: 9 in]
    n36 = call "ZDataVIS_Index_Wavenames.vi"("wave names"=w89) -> ("Index, Wavenames"=w86:string[][])  [unwired: 10 in]
    n37 = case shown="True" w76 {
      tunnel: w75 -> [w99 w102]
      tunnel: [w99 w100] -> w69
      frame False {
      }
      frame True {
        n38 = Index Array(array=w102) -> (element=w103:dbl[])  [unwired: 2 in]
        n39 = call "ZDataVIS_Fix_Filtered_Time.vi"("time array from one itx"=w103) -> ("fixed itx time array"=w101:dbl[])  [unwired: 10 in]
        n40 = Replace Array Subset(array=w102, new element=w101) -> (w100:dbl[][])  [unwired: 2 in]
      }
    }
    n41 = Array Size(array=w69) -> (size(s)=w67:i32[])
    n42 = Build Array (concatenate)(w68, w67) -> (→"ITX sizes (#itx, #chan, #samp)":i32[])
    n43 = for {
      N -> [w96]
      tunnel: w69 -> [w97] mode=indexing
      shift-right: [w98] -> w73
      shift-left: w72 -> [w93]
      tunnel: w71 -> [w92] mode=indexing
      tunnel: [w96] -> _
      tunnel: [w95] -> w70 mode=indexing
      n44 = Write to Binary File(file (use dialog)=w92, data=w97, error in=w93, 5:TRUE) -> (refnum out=w95:refnum<file>, error out=w98:errorcluster)  [unwired: 2 in, 1 out]
    }
    "#itx" <- w68
  }
  "Index, Wavenames" <- w29
  "\"notes \"" <- w20
  n45 = for {
    tunnel: w5 -> [w107] mode=indexing
    shift-right: [w105] -> w3
    shift-left: w4 -> [w106]
    tunnel: [w104] -> w2 mode=indexing
    n46 = Close File(refnum=w107, error in=w106) -> (path=w104:path, error out=w105:errorcluster)
  }
  "generated files" <- w2
  n47 = call-dynamic "PB_Clear.vi"("error in (no error)"=w3, "WF-ProgressBar in"=w28) -> ("error out"=→"error out":errorcluster)  [unwired: 8 in, 1 out]
